vi "ParseSpec2.vi"(8 "error in (no error)":errorcluster, 11 "Spec XML":string="<?xml version=\"1.0\" encoding=\"utf-8\"?>\n<Medulla>\n  <Doctype>Result</Doctype>\n  <Checksum>Spec</Checksum>\n  <DriverKey>NA</DriverKey>\n  <SpecId>NA</SpecId>\n  <TransactionId>0</TransactionId>\n  <AccountID>Audinate</AccountID>\n  <SpecName>Fremont_PCB</SpecName>\n  <WorkflowStep>Fremont_PCB</WorkflowStep>\n  <SerialNumber></SerialNumber>\n  <BatchNumber></BatchNumber>\n  <Status></Status>\n  <Comment></Comment>\n  <FirstFail></FirstFail>\n  <Employee></Employee>\n  <LocalMachine></LocalMachine>\n  <ResourceKey></ResourceKey>\n  <Date></Date>\n  <Time></Time>\n  <Duration></Duration>\n  <DUTPosition />\n  <Components></Components>\n  <Attributes></Attributes>\n  <Tests>\n    <Test>\n      <Code>1</Code>\n      <Name>Short_Circuit</Name>\n      <Description>short circuit tests</Description>\n      <Group></Group>\n      <IsGroup>Yes</IsGroup>\n      <Tag>Short_Circuit</Tag>\n      <Method></Method>\n      <Parameter />\n      <DataType></DataType>\n      <Value></Value>\n      <Status></Status>\n      <LimitLo></LimitLo>\n      <LimitHi></LimitHi>\n      <StringMatch></StringMatch>\n      <BooleanMatch></BooleanMatch>\n      <DisplayFormat></DisplayFormat>\n      <Units></Units>\n      <TestTime></TestTime>\n    </Test>\n    <Test>\n      <Code>1.1</Code>\n      <Name>Short_Circuit_Test</Name>\n      <Description>Tests the short circuit</Description>\n      <Group>Short_Circuit</Group>\n      <IsGroup>No</IsGroup>\n      <Tag>Short_Circuit:Short_Circuit_Test</Tag>\n      <Method>Test_Short_Circuit</Method>\n      <Parameter></Parameter>\n      <DataType>Dbl</DataType>\n      <Value></Value>\n      <Status></Status>\n      <LimitLo>-0.5</LimitLo>\n      <LimitHi>2.5</LimitHi>\n      <StringMatch></StringMatch>\n      <BooleanMatch></BooleanMatch>\n      <DisplayFormat>%.1f</DisplayFormat>\n      <Units>_mA</Units>\n      <TestTime></TestTime>\n    </Test>\n    <Test>\n      <Code>2</Code>\n      <Name>Power_On_3V3</Name>\n      <Description>Power on tests</Description>\n      <Group></Group>\n      <IsGroup>Yes</IsGroup>\n      <Tag>Power_On_3V3</Tag>\n      <Method></Method>\n      <Parameter />\n      <DataType></DataType>\n      <Value></Value>\n      <Status></Status>\n      <LimitLo></LimitLo>\n      <LimitHi></LimitHi>\n      <StringMatch></StringMatch>\n      <BooleanMatch></BooleanMatch>\n      <DisplayFormat></DisplayFormat>\n      <Units></Units>\n      <TestTime></TestTime>\n    </Test>\n    <Test>\n      <Code>2.1</Code>\n      <Name>Setup</Name>\n      <Description>Setup power on 3V3</Description>\n      <Group>Power_On_3V3</Group>\n      <IsGroup>No</IsGroup>\n      <Tag>Power_On_3V3:Setup</Tag>\n      <Method>Setup_Power_On</Method>\n      <Parameter></Parameter>\n      <DataType>Boolean</DataType>\n      <Value></Value>\n      <Status></Status>\n      <LimitLo></LimitLo>\n      <LimitHi></LimitHi>\n      <StringMatch></StringMatch>\n      <BooleanMatch>1</BooleanMatch>\n      <DisplayFormat></DisplayFormat>\n      <Units></Units>\n      <TestTime></TestTime>\n    </Test>\n    <Test>\n      <Code>2.2</Code>\n      <Name>Test_3V3_I</Name>\n      <Description>Test the 3V3 line</Description>\n      <Group>Power_On_3V3</Group>\n      <IsGroup>No</IsGroup>\n      <Tag>Power_On_3V3:Test_3V3_I</Tag>\n      <Method>Test_Power_On</Method>\n      <Parameter></Parameter>\n      <DataType>Dbl</DataType>\n      <Value></Value>\n      <Status></Status>\n      <LimitLo>50</LimitLo>\n      <LimitHi>500</LimitHi>\n      <StringMatch></StringMatch>\n      <BooleanMatch></BooleanMatch>\n      <DisplayFormat>%.1f</DisplayFormat>\n      <Units>_mA</Units>\n      <TestTime></TestTime>\n    </Test>\n    <Test>\n      <Code>3</Code>\n      <Name>Program_DUT</Name>\n      <Description>Perform JTAG programming</Description>\n      <Group></Group>\n      <IsGroup>Yes</IsGroup>\n      <Tag>Program_DUT</Tag>\n      <Method></Method>\n      <Parameter />\n      <DataType></DataType>\n      <Value></Value>\n      <Status></Status>\n      <LimitLo></LimitLo>\n      <LimitHi></LimitHi>\n      <StringMatch></StringMatch>\n      <BooleanMatch></BooleanMatch>\n      <DisplayFormat></DisplayFormat>\n      <Units></Units>\n      <TestTime></TestTime>\n    </Test>\n    <Test>\n      <Code>3.1</Code>\n      <Name>JTAG_Image</Name>\n      <Description>Set the FPGA image</Description>\n      <Group>Program_DUT</Group>\n      <IsGroup>No</IsGroup>\n      <Tag>Program_DUT:JTAG_Image</Tag>\n      <Method>ProgramTestImage</Method>\n      <Parameter>fremont_tx.bit</Parameter>\n      <DataType>Boolean</DataType>\n      <Value></Value>\n      <Status></Status>\n      <LimitLo></LimitLo>\n      <LimitHi></LimitHi>\n      <StringMatch></StringMatch>\n      <BooleanMatch>1</BooleanMatch>\n      <DisplayFormat></DisplayFormat>\n      <Units></Units>\n      <TestTime></TestTime>\n    </Test>\n    <Test>\n      <Code>4</Code>\n      <Name>Operating_Current</Name>\n      <Description>Measure the operating V and I</Description>\n      <Group></Group>\n      <IsGroup>Yes</IsGroup>\n      <Tag>Operating_Current</Tag>\n      <Method></Method>\n      <Parameter />\n      <DataType></DataType>\n      <Value></Value>\n      <Status></Status>\n      <LimitLo></LimitLo>\n      <LimitHi></LimitHi>\n      <StringMatch></StringMatch>\n      <BooleanMatch></BooleanMatch>\n      <DisplayFormat></DisplayFormat>\n      <Units></Units>\n      <TestTime></TestTime>\n    </Test>\n    <Test>\n      <Code>4.1</Code>\n      <Name>Test_3V3_V</Name>\n      <Description>Test the 3V3 line V</Description>\n      <Group>Operating_Current</Group>\n      <IsGroup>No</IsGroup>\n      <Tag>Operating_Current:Test_3V3_V</Tag>\n      <Method>Test_Operating_Voltage</Method>\n      <Parameter></Parameter>\n      <DataType>Dbl</DataType>\n      <Value></Value>\n      <Status></Status>\n      <LimitLo>3.2</LimitLo>\n      <LimitHi>3.4</LimitHi>\n      <StringMatch></StringMatch>\n      <BooleanMatch></BooleanMatch>\n      <DisplayFormat>%.2f</DisplayFormat>\n      <Units>_V</Units>\n      <TestTime></TestTime>\n    </Test>\n    <Test>\n      <Code>4.2</Code>\n      <Name>Test_3V3_I</Name>\n      <Description>Test the 3V3 line V</Description>\n      <Group>Operating_Current</Group>\n      <IsGroup>No</IsGroup>\n      <Tag>Opearating_Current:Test_3V3_I</Tag>\n      <Method>Test_Operating_Current</Method>\n      <Parameter></Parameter>\n      <DataType>Dbl</DataType>\n      <Value></Value>\n      <Status></Status>\n      <LimitLo>200</LimitLo>\n      <LimitHi>500</LimitHi>\n      <StringMatch></StringMatch>\n      <BooleanMatch></BooleanMatch>\n      <DisplayFormat>%.1f</DisplayFormat>\n      <Units>_mA</Units>\n      <TestTime></TestTime>\n    </Test>\n    <Test>\n      <Code>5</Code>\n      <Name>RS232_Verification</Name>\n      <Description>Verify that can read serial</Description>\n      <Group></Group>\n      <IsGroup>Yes</IsGroup>\n      <Tag>RS232_Verification</Tag>\n      <Method></Method>\n      <Parameter />\n      <DataType></DataType>\n      <Value></Value>\n      <Status></Status>\n      <LimitLo></LimitLo>\n      <LimitHi></LimitHi>\n      <StringMatch></StringMatch>\n      <BooleanMatch></BooleanMatch>\n      <DisplayFormat></DisplayFormat>\n      <Units></Units>\n      <TestTime></TestTime>\n    </Test>\n    <Test>\n      <Code>5.1</Code>\n      <Name>Set_HIZ</Name>\n      <Description>Check HIZ response</Description>\n      <Group>RS232_Verification</Group>\n      <IsGroup>No</IsGroup>\n      <Tag>RS232_Verification:Set_HIZ</Tag>\n      <Method>RS232_Verification</Method>\n      <Parameter></Parameter>\n      <DataType>Boolean</DataType>\n      <Value></Value>\n      <Status></Status>\n      <LimitLo></LimitLo>\n      <LimitHi></LimitHi>\n      <StringMatch></StringMatch>\n      <BooleanMatch>1</BooleanMatch>\n      <DisplayFormat></DisplayFormat>\n      <Units></Units>\n      <TestTime></TestTime>\n    </Test>\n    <Test>\n      <Code>6</Code>\n      <Name>DDR2_Verification</Name>\n      <Description>DDR2 Verification</Description>\n      <Group></Group>\n      <IsGroup>Yes</IsGroup>\n      <Tag>DDR2_Verification</Tag>\n      <Method></Method>\n      <Parameter />\n      <DataType></DataType>\n      <Value></Value>\n      <Status></Status>\n      <LimitLo></LimitLo>\n      <LimitHi></LimitHi>\n      <StringMatch></StringMatch>\n      <BooleanMatch></BooleanMatch>\n      <DisplayFormat></DisplayFormat>\n      <Units></Units>\n      <TestTime></TestTime>\n    </Test>\n    <Test>\n      <Code>6.1</Code>\n      <Name>DDR2_Memory</Name>\n      <Description>Check DDR2 Mem</Description>\n      <Group>DDR2_Verification</Group>\n      <IsGroup>No</IsGroup>\n      <Tag>DDR2_Verification:DDR2_Memory</Tag>\n      <Method>DDR2_Verification</Method>\n      <Parameter></Parameter>\n      <DataType>Boolean</DataType>\n      <Value></Value>\n      <Status></Status>\n      <LimitLo></LimitLo>\n      <LimitHi></LimitHi>\n      <StringMatch></StringMatch>\n      <BooleanMatch>1</BooleanMatch>\n      <DisplayFormat></DisplayFormat>\n      <Units></Units>\n      <TestTime></TestTime>\n    </Test>\n    <Test>\n      <Code>7</Code>\n      <Name>SPI_Flash</Name>\n      <Description>SPI Flash Programing</Description>\n      <Group></Group>\n      <IsGroup>Yes</IsGroup>\n      <Tag>SPI_Flash</Tag>\n      <Method></Method>\n      <Parameter />\n      <DataType></DataType>\n      <Value></Value>\n      <Status></Status>\n      <LimitLo></LimitLo>\n      <LimitHi></LimitHi>\n      <StringMatch></StringMatch>\n      <BooleanMatch></BooleanMatch>\n      <DisplayFormat></DisplayFormat>\n      <Units></Units>\n      <TestTime></TestTime>\n    </Test>\n    <Test>\n      <Code>7.1</Code>\n      <Name>Program</Name>\n      <Description>Program the fremont</Description>\n      <Group>SPI_Flash</Group>\n      <IsGroup>No</IsGroup>\n      <Tag>SPI_Flash:Program</Tag>\n      <Method>StartFlash</Method>\n      <Parameter>ULL_FREMONT_TX.bin</Parameter>\n      <DataType>Boolean</DataType>\n      <Value></Value>\n      <Status></Status>\n      <LimitLo></LimitLo>\n      <LimitHi></LimitHi>\n      <StringMatch></StringMatch>\n      <BooleanMatch>1</BooleanMatch>\n      <DisplayFormat></DisplayFormat>\n      <Units></Units>\n      <TestTime></TestTime>\n    </Test>\n    <Test>\n      <Code>8</Code>\n      <Name>Frequency_Tests</Name>\n      <Description>Frequency tests</Description>\n      <Group></Group>\n      <IsGroup>Yes</IsGroup>\n      <Tag>Frequency_Tests</Tag>\n      <Method></Method>\n      <Parameter />\n      <DataType></DataType>\n      <Value></Value>\n      <Status></Status>\n      <LimitLo></LimitLo>\n      <LimitHi></LimitHi>\n      <StringMatch></StringMatch>\n      <BooleanMatch></BooleanMatch>\n      <DisplayFormat></DisplayFormat>\n      <Units></Units>\n      <TestTime></TestTime>\n    </Test>\n    <Test>\n      <Code>8.1</Code>\n      <Name>VCXO_0_LF</Name>\n      <Description>frequency test</Description>\n      <Group>Frequency_Tests</Group>\n      <IsGroup>No</IsGroup>\n      <Tag>Frequency_Tests:VCXO_0_LF</Tag>\n      <Method>Frequency_Test_VCXO_0_LF</Method>\n      <Parameter></Parameter>\n      <DataType>Dbl</DataType>\n      <Value></Value>\n      <Status></Status>\n      <LimitLo>983090</LimitLo>\n      <LimitHi>983094</LimitHi>\n      <StringMatch></StringMatch>\n      <BooleanMatch></BooleanMatch>\n      <DisplayFormat>%.0f</DisplayFormat>\n      <Units>_Hz</Units>\n      <TestTime></TestTime>\n    </Test>\n    <Test>\n      <Code>8.2</Code>\n      <Name>VCXO_0_HF</Name>\n      <Description>frequency test</Description>\n      <Group>Frequency_Tests</Group>\n      <IsGroup>No</IsGroup>\n      <Tag>Frequency_Tests:VCXO_0_HF</Tag>\n      <Method>Frequency_Test_VCXO_0_HF</Method>\n      <Parameter></Parameter>\n      <DataType>Dbl</DataType>\n      <Value></Value>\n      <Status></Status>\n      <LimitLo>983090</LimitLo>\n      <LimitHi>983094</LimitHi>\n      <StringMatch></StringMatch>\n      <BooleanMatch></BooleanMatch>\n      <DisplayFormat>%.0f</DisplayFormat>\n      <Units>_Hz</Units>\n      <TestTime></TestTime>\n    </Test>\n    <Test>\n      <Code>8.3</Code>\n      <Name>VCXO_M</Name>\n      <Description>frequency test</Description>\n      <Group>Frequency_Tests</Group>\n      <IsGroup>No</IsGroup>\n      <Tag>Frequency_Tests:VCXO_M</Tag>\n      <Method>Frequency_Test_VCXO_M</Method>\n      <Parameter></Parameter>\n      <DataType>Dbl</DataType>\n      <Value></Value>\n      <Status></Status>\n      <LimitLo>983090</LimitLo>\n      <LimitHi>983094</LimitHi>\n      <StringMatch></StringMatch>\n      <BooleanMatch></BooleanMatch>\n      <DisplayFormat>%.0f</DisplayFormat>\n      <Units>_Hz</Units>\n      <TestTime></TestTime>\n    </Test>\n    <Test>\n      <Code>8.4</Code>\n      <Name>VCXO_H</Name>\n      <Description>frequency test</Description>\n      <Group>Frequency_Tests</Group>\n      <IsGroup>No</IsGroup>\n      <Tag>Frequency_Tests:VCXO_H</Tag>\n      <Method>Frequency_Test_VCXO_H</Method>\n      <Parameter></Parameter>\n      <DataType>Dbl</DataType>\n      <Value></Value>\n      <Status></Status>\n      <LimitLo>983090</LimitLo>\n      <LimitHi>983094</LimitHi>\n      <StringMatch></StringMatch>\n      <BooleanMatch></BooleanMatch>\n      <DisplayFormat>%.0f</DisplayFormat>\n      <Units>_Hz</Units>\n      <TestTime></TestTime>\n    </Test>\n    <Test>\n      <Code>8.5</Code>\n      <Name>VCXO_L</Name>\n      <Description>frequency test</Description>\n      <Group>Frequency_Tests</Group>\n      <IsGroup>No</IsGroup>\n      <Tag>Frequency_Tests:VCXO_L</Tag>\n      <Method>Frequency_Test_VCXO_L</Method>\n      <Parameter></Parameter>\n      <DataType>Dbl</DataType>\n      <Value></Value>\n      <Status></Status>\n      <LimitLo>983090</LimitLo>\n      <LimitHi>983094</LimitHi>\n      <StringMatch></StringMatch>\n      <BooleanMatch></BooleanMatch>\n      <DisplayFormat>%.0f</DisplayFormat>\n      <Units>_Hz</Units>\n      <TestTime></TestTime>\n    </Test>\n    <Test>\n      <Code>8.6</Code>\n      <Name>VCXO_2</Name>\n      <Description>frequency test</Description>\n      <Group>Frequency_Tests</Group>\n      <IsGroup>No</IsGroup>\n      <Tag>Frequency_Tests:VCXO_2</Tag>\n      <Method>Frequency_Test_VCXO_2</Method>\n      <Parameter></Parameter>\n      <DataType>Dbl</DataType>\n      <Value></Value>\n      <Status></Status>\n      <LimitLo>983090</LimitLo>\n      <LimitHi>983094</LimitHi>\n      <StringMatch></StringMatch>\n      <BooleanMatch></BooleanMatch>\n      <DisplayFormat>%.0f</DisplayFormat>\n      <Units>_Hz</Units>\n      <TestTime></TestTime>\n    </Test>\n    <Test>\n      <Code>9</Code>\n      <Name>VCXO_PWM_Resistors</Name>\n      <Description>VCXO_PWM</Description>\n      <Group></Group>\n      <IsGroup>Yes</IsGroup>\n      <Tag>VCXO_PWM</Tag>\n      <Method></Method>\n      <Parameter />\n      <DataType></DataType>\n      <Value></Value>\n      <Status></Status>\n      <LimitLo></LimitLo>\n      <LimitHi></LimitHi>\n      <StringMatch></StringMatch>\n      <BooleanMatch></BooleanMatch>\n      <DisplayFormat></DisplayFormat>\n      <Units></Units>\n      <TestTime></TestTime>\n    </Test>\n    <Test>\n      <Code>9.1</Code>\n      <Name>I_H_H</Name>\n      <Description></Description>\n      <Group>VCXO_PWM</Group>\n      <IsGroup>No</IsGroup>\n      <Tag>VCXO_PWM:I_H_H</Tag>\n      <Method>Test_VCXO_PWM_I_H_H</Method>\n      <Parameter></Parameter>\n      <DataType>Dbl</DataType>\n      <Value></Value>\n      <Status></Status>\n      <LimitLo>1.5</LimitLo>\n      <LimitHi>1.7</LimitHi>\n      <StringMatch></StringMatch>\n      <BooleanMatch></BooleanMatch>\n      <DisplayFormat>%.2f</DisplayFormat>\n      <Units>_V</Units>\n      <TestTime></TestTime>\n    </Test>\n    <Test>\n      <Code>9.2</Code>\n      <Name>I_L_L</Name>\n      <Description></Description>\n      <Group>VCXO_PWM</Group>\n      <IsGroup>No</IsGroup>\n      <Tag>VCXO_PWM:I_L_L</Tag>\n      <Method>Test_VCXO_PWM_I_L_L</Method>\n      <Parameter></Parameter>\n      <DataType>Dbl</DataType>\n      <Value></Value>\n      <Status></Status>\n      <LimitLo>1.5</LimitLo>\n      <LimitHi>1.7</LimitHi>\n      <StringMatch></StringMatch>\n      <BooleanMatch></BooleanMatch>\n      <DisplayFormat>%.2f</DisplayFormat>\n      <Units>_V</Units>\n      <TestTime></TestTime>\n    </Test>\n    <Test>\n      <Code>9.3</Code>\n      <Name>I_H_L</Name>\n      <Description></Description>\n      <Group>VCXO_PWM</Group>\n      <IsGroup>No</IsGroup>\n      <Tag>VCXO_PWM:I_H_L</Tag>\n      <Method>Test_VCXO_PWM_I_H_L</Method>\n      <Parameter></Parameter>\n      <DataType>Dbl</DataType>\n      <Value></Value>\n      <Status></Status>\n      <LimitLo>1.5</LimitLo>\n      <LimitHi>1.7</LimitHi>\n      <StringMatch></StringMatch>\n      <BooleanMatch></BooleanMatch>\n      <DisplayFormat>%.2f</DisplayFormat>\n      <Units>_V</Units>\n      <TestTime></TestTime>\n    </Test>\n    <Test>\n      <Code>9.4</Code>\n      <Name>I_L_H</Name>\n      <Description></Description>\n      <Group>VCXO_PWM</Group>\n      <IsGroup>No</IsGroup>\n      <Tag>VCXO_PWM:I_L_H</Tag>\n      <Method>Test_VCXO_PWM_I_L_H</Method>\n      <Parameter></Parameter>\n      <DataType>Dbl</DataType>\n      <Value></Value>\n      <Status></Status>\n      <LimitLo>1.5</LimitLo>\n      <LimitHi>1.7</LimitHi>\n      <StringMatch></StringMatch>\n      <BooleanMatch></BooleanMatch>\n      <DisplayFormat>%.2f</DisplayFormat>\n      <Units>_V</Units>\n      <TestTime></TestTime>\n    </Test>\n    <Test>\n      <Code>10</Code>\n      <Name>Pin_Tests</Name>\n      <Description>Test all the pins for H and L</Description>\n      <Group></Group>\n      <IsGroup>Yes</IsGroup>\n      <Tag>Pin_Tests</Tag>\n      <Method></Method>\n      <Parameter />\n      <DataType></DataType>\n      <Value></Value>\n      <Status></Status>\n      <LimitLo></LimitLo>\n      <LimitHi></LimitHi>\n      <StringMatch></StringMatch>\n      <BooleanMatch></BooleanMatch>\n      <DisplayFormat></DisplayFormat>\n      <Units></Units>\n      <TestTime></TestTime>\n    </Test>\n    <Test>\n      <Code>10.1</Code>\n      <Name>Setup_Pins</Name>\n      <Description>setup the pin tests </Description>\n      <Group>Pin_Tests</Group>\n      <IsGroup>No</IsGroup>\n      <Tag>Pin_Tests:Setup_Pins</Tag>\n      <Method>Setup_Pin_Tests</Method>\n      <Parameter></Parameter>\n      <DataType>Boolean</DataType>\n      <Value></Value>\n      <Status></Status>\n      <LimitLo></LimitLo>\n      <LimitHi></LimitHi>\n      <StringMatch></StringMatch>\n      <BooleanMatch>1</BooleanMatch>\n      <DisplayFormat></DisplayFormat>\n      <Units></Units>\n      <TestTime></TestTime>\n    </Test>\n    <Test>\n      <Code>10.2</Code>\n      <Name>SELECTOR_1_H</Name>\n      <Description></Description>\n      <Group>Pin_Tests</Group>\n      <IsGroup>No</IsGroup>\n      <Tag>Pin_Tests:SELECTOR_1_H</Tag>\n      <Method>Test_Pin_N_High</Method>\n      <Parameter>CH1</Parameter>\n      <DataType>Dbl</DataType>\n      <Value></Value>\n      <Status></Status>\n      <LimitLo>3.2</LimitLo>\n      <LimitHi>3.4</LimitHi>\n      <StringMatch></StringMatch>\n      <BooleanMatch></BooleanMatch>\n      <DisplayFormat>%.2f</DisplayFormat>\n      <Units>_V</Units>\n      <TestTime></TestTime>\n    </Test>\n    <Test>\n      <Code>10.3</Code>\n      <Name>SELECTOR_1_L</Name>\n      <Description></Description>\n      <Group>Pin_Tests</Group>\n      <IsGroup>No</IsGroup>\n      <Tag>Pin_Tests:SELECTOR_1_L</Tag>\n      <Method>Test_Pin_N_Low</Method>\n      <Parameter>CH1</Parameter>\n      <DataType>Dbl</DataType>\n      <Value></Value>\n      <Status></Status>\n      <LimitLo>0</LimitLo>\n      <LimitHi>0.01</LimitHi>\n      <StringMatch></StringMatch>\n      <BooleanMatch></BooleanMatch>\n      <DisplayFormat>%.2f</DisplayFormat>\n      <Units>_V</Units>\n      <TestTime></TestTime>\n    </Test>\n    <Test>\n      <Code>10.4</Code>\n      <Name>SELECTOR_2_H</Name>\n      <Description></Description>\n      <Group>Pin_Tests</Group>\n      <IsGroup>No</IsGroup>\n      <Tag>Pin_Tests:SELECTOR_2_H</Tag>\n      <Method>Test_Pin_N_High</Method>\n      <Parameter>CH2</Parameter>\n      <DataType>Dbl</DataType>\n      <Value></Value>\n      <Status></Status>\n      <LimitLo>3.2</LimitLo>\n      <LimitHi>3.4</LimitHi>\n      <StringMatch></StringMatch>\n      <BooleanMatch></BooleanMatch>\n      <DisplayFormat>%.2f</DisplayFormat>\n      <Units>_V</Units>\n      <TestTime></TestTime>\n    </Test>\n    <Test>\n      <Code>10.5</Code>\n      <Name>SELECTOR_2_L</Name>\n      <Description></Description>\n      <Group>Pin_Tests</Group>\n      <IsGroup>No</IsGroup>\n      <Tag>Pin_Tests:SELECTOR_2_L</Tag>\n      <Method>Test_Pin_N_Low</Method>\n      <Parameter>CH2</Parameter>\n      <DataType>Dbl</DataType>\n      <Value></Value>\n      <Status></Status>\n      <LimitLo>0</LimitLo>\n      <LimitHi>0.01</LimitHi>\n      <StringMatch></StringMatch>\n      <BooleanMatch></BooleanMatch>\n      <DisplayFormat>%.2f</DisplayFormat>\n      <Units>_V</Units>\n      <TestTime></TestTime>\n    </Test>\n    <Test>\n      <Code>10.6</Code>\n      <Name>SELECTOR_3_H</Name>\n      <Description></Description>\n      <Group>Pin_Tests</Group>\n      <IsGroup>No</IsGroup>\n      <Tag>Pin_Tests:SELECTOR_3_H</Tag>\n      <Method>Test_Pin_N_High</Method>\n      <Parameter>CH3</Parameter>\n      <DataType>Dbl</DataType>\n      <Value></Value>\n      <Status></Status>\n      <LimitLo>3.2</LimitLo>\n      <LimitHi>3.4</LimitHi>\n      <StringMatch></StringMatch>\n      <BooleanMatch></BooleanMatch>\n      <DisplayFormat>%.2f</DisplayFormat>\n      <Units>_V</Units>\n      <TestTime></TestTime>\n    </Test>\n    <Test>\n      <Code>10.7</Code>\n      <Name>SELECTOR_3_L</Name>\n      <Description></Description>\n      <Group>Pin_Tests</Group>\n      <IsGroup>No</IsGroup>\n      <Tag>Pin_Tests:SELECTOR_3_L</Tag>\n      <Method>Test_Pin_N_Low</Method>\n      <Parameter>CH3</Parameter>\n      <DataType>Dbl</DataType>\n      <Value></Value>\n      <Status></Status>\n      <LimitLo>0</LimitLo>\n      <LimitHi>0.01</LimitHi>\n      <StringMatch></StringMatch>\n      <BooleanMatch></BooleanMatch>\n      <DisplayFormat>%.2f</DisplayFormat>\n      <Units>_V</Units>\n      <TestTime></TestTime>\n    </Test>\n    <Test>\n      <Code>10.8</Code>\n      <Name>SELECTOR_4_H</Name>\n      <Description></Description>\n      <Group>Pin_Tests</Group>\n      <IsGroup>No</IsGroup>\n      <Tag>Pin_Tests:SELECTOR_4_H</Tag>\n      <Method>Test_Pin_N_High</Method>\n      <Parameter>CH4</Parameter>\n      <DataType>Dbl</DataType>\n      <Value></Value>\n      <Status></Status>\n      <LimitLo>3.2</LimitLo>\n      <LimitHi>3.4</LimitHi>\n      <StringMatch></StringMatch>\n      <BooleanMatch></BooleanMatch>\n      <DisplayFormat>%.2f</DisplayFormat>\n      <Units>_V</Units>\n      <TestTime></TestTime>\n    </Test>\n    <Test>\n      <Code>10.9</Code>\n      <Name>SELECTOR_4_L</Name>\n      <Description></Description>\n      <Group>Pin_Tests</Group>\n      <IsGroup>No</IsGroup>\n      <Tag>Pin_Tests:SELECTOR_4_L</Tag>\n      <Method>Test_Pin_N_Low</Method>\n      <Parameter>CH4</Parameter>\n      <DataType>Dbl</DataType>\n      <Value></Value>\n      <Status></Status>\n      <LimitLo>0</LimitLo>\n      <LimitHi>0.01</LimitHi>\n      <StringMatch></StringMatch>\n      <BooleanMatch></BooleanMatch>\n      <DisplayFormat>%.2f</DisplayFormat>\n      <Units>_V</Units>\n      <TestTime></TestTime>\n    </Test>\n    <Test>\n      <Code>10.10</Code>\n      <Name>SELECTOR_5_H</Name>\n      <Description></Description>\n      <Group>Pin_Tests</Group>\n      <IsGroup>No</IsGroup>\n      <Tag>Pin_Tests:SELECTOR_5_H</Tag>\n      <Method>Test_Pin_N_High</Method>\n      <Parameter>CH5</Parameter>\n      <DataType>Dbl</DataType>\n      <Value></Value>\n      <Status></Status>\n      <LimitLo>3.2</LimitLo>\n      <LimitHi>3.4</LimitHi>\n      <StringMatch></StringMatch>\n      <BooleanMatch></BooleanMatch>\n      <DisplayFormat>%.2f</DisplayFormat>\n      <Units>_V</Units>\n      <TestTime></TestTime>\n    </Test>\n    <Test>\n      <Code>10.11</Code>\n      <Name>SELECTOR_5_L</Name>\n      <Description></Description>\n      <Group>Pin_Tests</Group>\n      <IsGroup>No</IsGroup>\n      <Tag>Pin_Tests:SELECTOR_5_L</Tag>\n      <Method>Test_Pin_N_Low</Method>\n      <Parameter>CH5</Parameter>\n      <DataType>Dbl</DataType>\n      <Value></Value>\n      <Status></Status>\n      <LimitLo>0</LimitLo>\n      <LimitHi>0.01</LimitHi>\n      <StringMatch></StringMatch>\n      <BooleanMatch></BooleanMatch>\n      <DisplayFormat>%.2f</DisplayFormat>\n      <Units>_V</Units>\n      <TestTime></TestTime>\n    </Test>\n    <Test>\n      <Code>10.12</Code>\n      <Name>SELECTOR_6_H</Name>\n      <Description></Description>\n      <Group>Pin_Tests</Group>\n      <IsGroup>No</IsGroup>\n      <Tag>Pin_Tests:SELECTOR_6_H</Tag>\n      <Method>Test_Pin_N_High</Method>\n      <Parameter>CH6</Parameter>\n      <DataType>Dbl</DataType>\n      <Value></Value>\n      <Status></Status>\n      <LimitLo>3.2</LimitLo>\n      <LimitHi>3.4</LimitHi>\n      <StringMatch></StringMatch>\n      <BooleanMatch></BooleanMatch>\n      <DisplayFormat>%.2f</DisplayFormat>\n      <Units>_V</Units>\n      <TestTime></TestTime>\n    </Test>\n    <Test>\n      <Code>10.13</Code>\n      <Name>SELECTOR_6_L</Name>\n      <Description></Description>\n      <Group>Pin_Tests</Group>\n      <IsGroup>No</IsGroup>\n      <Tag>Pin_Tests:SELECTOR_6_L</Tag>\n      <Method>Test_Pin_N_Low</Method>\n      <Parameter>CH6</Parameter>\n      <DataType>Dbl</DataType>\n      <Value></Value>\n      <Status></Status>\n      <LimitLo>0</LimitLo>\n      <LimitHi>0.01</LimitHi>\n      <StringMatch></StringMatch>\n      <BooleanMatch></BooleanMatch>\n      <DisplayFormat>%.2f</DisplayFormat>\n      <Units>_V</Units>\n      <TestTime></TestTime>\n    </Test>\n    <Test>\n      <Code>10.14</Code>\n      <Name>SELECTOR_7_H</Name>\n      <Description></Description>\n      <Group>Pin_Tests</Group>\n      <IsGroup>No</IsGroup>\n      <Tag>Pin_Tests:SELECTOR_7_H</Tag>\n      <Method>Test_Pin_N_High</Method>\n      <Parameter>CH7</Parameter>\n      <DataType>Dbl</DataType>\n      <Value></Value>\n      <Status></Status>\n      <LimitLo>3.2</LimitLo>\n      <LimitHi>3.4</LimitHi>\n      <StringMatch></StringMatch>\n      <BooleanMatch></BooleanMatch>\n      <DisplayFormat>%.2f</DisplayFormat>\n      <Units>_V</Units>\n      <TestTime></TestTime>\n    </Test>\n    <Test>\n      <Code>10.15</Code>\n      <Name>SELECTOR_7_L</Name>\n      <Description></Description>\n      <Group>Pin_Tests</Group>\n      <IsGroup>No</IsGroup>\n      <Tag>Pin_Tests:SELECTOR_7_L</Tag>\n      <Method>Test_Pin_N_Low</Method>\n      <Parameter>CH7</Parameter>\n      <DataType>Dbl</DataType>\n      <Value></Value>\n      <Status></Status>\n      <LimitLo>0</LimitLo>\n      <LimitHi>0.01</LimitHi>\n      <StringMatch></StringMatch>\n      <BooleanMatch></BooleanMatch>\n      <DisplayFormat>%.2f</DisplayFormat>\n      <Units>_V</Units>\n      <TestTime></TestTime>\n    </Test>\n    <Test>\n      <Code>10.16</Code>\n      <Name>SELECTOR_8_H</Name>\n      <Description></Description>\n      <Group>Pin_Tests</Group>\n      <IsGroup>No</IsGroup>\n      <Tag>Pin_Tests:SELECTOR_8_H</Tag>\n      <Method>Test_Pin_N_High</Method>\n      <Parameter>CH8</Parameter>\n      <DataType>Dbl</DataType>\n      <Value></Value>\n      <Status></Status>\n      <LimitLo>3.2</LimitLo>\n      <LimitHi>3.4</LimitHi>\n      <StringMatch></StringMatch>\n      <BooleanMatch></BooleanMatch>\n      <DisplayFormat>%.2f</DisplayFormat>\n      <Units>_V</Units>\n      <TestTime></TestTime>\n    </Test>\n    <Test>\n      <Code>10.17</Code>\n      <Name>SELECTOR_8_L</Name>\n      <Description></Description>\n      <Group>Pin_Tests</Group>\n      <IsGroup>No</IsGroup>\n      <Tag>Pin_Tests:SELECTOR_8_L</Tag>\n      <Method>Test_Pin_N_Low</Method>\n      <Parameter>CH8</Parameter>\n      <DataType>Dbl</DataType>\n      <Value></Value>\n      <Status></Status>\n      <LimitLo>0</LimitLo>\n      <LimitHi>0.01</LimitHi>\n      <StringMatch></StringMatch>\n      <BooleanMatch></BooleanMatch>\n      <DisplayFormat>%.2f</DisplayFormat>\n      <Units>_V</Units>\n      <TestTime></TestTime>\n    </Test>\n    <Test>\n      <Code>10.18</Code>\n      <Name>SELECTOR_9_H</Name>\n      <Description></Description>\n      <Group>Pin_Tests</Group>\n      <IsGroup>No</IsGroup>\n      <Tag>Pin_Tests:SELECTOR_9_H</Tag>\n      <Method>Test_Pin_N_High</Method>\n      <Parameter>CH9</Parameter>\n      <DataType>Dbl</DataType>\n      <Value></Value>\n      <Status></Status>\n      <LimitLo>3.2</LimitLo>\n      <LimitHi>3.4</LimitHi>\n      <StringMatch></StringMatch>\n      <BooleanMatch></BooleanMatch>\n      <DisplayFormat>%.2f</DisplayFormat>\n      <Units>_V</Units>\n      <TestTime></TestTime>\n    </Test>\n    <Test>\n      <Code>10.19</Code>\n      <Name>SELECTOR_9_L</Name>\n      <Description></Description>\n      <Group>Pin_Tests</Group>\n      <IsGroup>No</IsGroup>\n      <Tag>Pin_Tests:SELECTOR_9_L</Tag>\n      <Method>Test_Pin_N_Low</Method>\n      <Parameter>CH9</Parameter>\n      <DataType>Dbl</DataType>\n      <Value></Value>\n      <Status></Status>\n      <LimitLo>0</LimitLo>\n      <LimitHi>0.01</LimitHi>\n      <StringMatch></StringMatch>\n      <BooleanMatch></BooleanMatch>\n      <DisplayFormat>%.2f</DisplayFormat>\n      <Units>_V</Units>\n      <TestTime></TestTime>\n    </Test>\n    <Test>\n      <Code>10.20</Code>\n      <Name>SELECTOR_10_H</Name>\n      <Description></Description>\n      <Group>Pin_Tests</Group>\n      <IsGroup>No</IsGroup>\n      <Tag>Pin_Tests:SELECTOR_10_H</Tag>\n      <Method>Test_Pin_N_High</Method>\n      <Parameter>CH10</Parameter>\n      <DataType>Dbl</DataType>\n      <Value></Value>\n      <Status></Status>\n      <LimitLo>3.2</LimitLo>\n      <LimitHi>3.4</LimitHi>\n      <StringMatch></StringMatch>\n      <BooleanMatch></BooleanMatch>\n      <DisplayFormat>%.2f</DisplayFormat>\n      <Units>_V</Units>\n      <TestTime></TestTime>\n    </Test>\n    <Test>\n      <Code>10.21</Code>\n      <Name>SELECTOR_10_L</Name>\n      <Description></Description>\n      <Group>Pin_Tests</Group>\n      <IsGroup>No</IsGroup>\n      <Tag>Pin_Tests:SELECTOR_10_L</Tag>\n      <Method>Test_Pin_N_Low</Method>\n      <Parameter>CH10</Parameter>\n      <DataType>Dbl</DataType>\n      <Value></Value>\n      <Status></Status>\n      <LimitLo>0</LimitLo>\n      <LimitHi>0.01</LimitHi>\n      <StringMatch></StringMatch>\n      <BooleanMatch></BooleanMatch>\n      <DisplayFormat>%.2f</DisplayFormat>\n      <Units>_V</Units>\n      <TestTime></TestTime>\n    </Test>\n    <Test>\n      <Code>10.22</Code>\n      <Name>SELECTOR_11_H</Name>\n      <Description></Description>\n      <Group>Pin_Tests</Group>\n      <IsGroup>No</IsGroup>\n      <Tag>Pin_Tests:SELECTOR_11_H</Tag>\n      <Method>Test_Pin_N_High</Method>\n      <Parameter>CH11</Parameter>\n      <DataType>Dbl</DataType>\n      <Value></Value>\n      <Status></Status>\n      <LimitLo>3.2</LimitLo>\n      <LimitHi>3.4</LimitHi>\n      <StringMatch></StringMatch>\n      <BooleanMatch></BooleanMatch>\n      <DisplayFormat>%.2f</DisplayFormat>\n      <Units>_V</Units>\n      <TestTime></TestTime>\n    </Test>\n    <Test>\n      <Code>10.23</Code>\n      <Name>SELECTOR_11_L</Name>\n      <Description></Description>\n      <Group>Pin_Tests</Group>\n      <IsGroup>No</IsGroup>\n      <Tag>Pin_Tests:SELECTOR_11_L</Tag>\n      <Method>Test_Pin_N_Low</Method>\n      <Parameter>CH11</Parameter>\n      <DataType>Dbl</DataType>\n      <Value></Value>\n      <Status></Status>\n      <LimitLo>0</LimitLo>\n      <LimitHi>0.01</LimitHi>\n      <StringMatch></StringMatch>\n      <BooleanMatch></BooleanMatch>\n      <DisplayFormat>%.2f</DisplayFormat>\n      <Units>_V</Units>\n      <TestTime></TestTime>\n    </Test>\n    <Test>\n      <Code>10.24</Code>\n      <Name>SELECTOR_12_H</Name>\n      <Description></Description>\n      <Group>Pin_Tests</Group>\n      <IsGroup>No</IsGroup>\n      <Tag>Pin_Tests:SELECTOR_12_H</Tag>\n      <Method>Test_Pin_N_High</Method>\n      <Parameter>CH12</Parameter>\n      <DataType>Dbl</DataType>\n      <Value></Value>\n      <Status></Status>\n      <LimitLo>3.2</LimitLo>\n      <LimitHi>3.4</LimitHi>\n      <StringMatch></StringMatch>\n      <BooleanMatch></BooleanMatch>\n      <DisplayFormat>%.2f</DisplayFormat>\n      <Units>_V</Units>\n      <TestTime></TestTime>\n    </Test>\n    <Test>\n      <Code>10.25</Code>\n      <Name>SELECTOR_12_L</Name>\n      <Description></Description>\n      <Group>Pin_Tests</Group>\n      <IsGroup>No</IsGroup>\n      <Tag>Pin_Tests:SELECTOR_12_L</Tag>\n      <Method>Test_Pin_N_Low</Method>\n      <Parameter>CH12</Parameter>\n      <DataType>Dbl</DataType>\n      <Value></Value>\n      <Status></Status>\n      <LimitLo>0</LimitLo>\n      <LimitHi>0.01</LimitHi>\n      <StringMatch></StringMatch>\n      <BooleanMatch></BooleanMatch>\n      <DisplayFormat>%.2f</DisplayFormat>\n      <Units>_V</Units>\n      <TestTime></TestTime>\n    </Test>\n    <Test>\n      <Code>10.26</Code>\n      <Name>SELECTOR_13_H</Name>\n      <Description></Description>\n      <Group>Pin_Tests</Group>\n      <IsGroup>No</IsGroup>\n      <Tag>Pin_Tests:SELECTOR_13_H</Tag>\n      <Method>Test_Pin_N_High</Method>\n      <Parameter>CH13</Parameter>\n      <DataType>Dbl</DataType>\n      <Value></Value>\n      <Status></Status>\n      <LimitLo>3.2</LimitLo>\n      <LimitHi>3.4</LimitHi>\n      <StringMatch></StringMatch>\n      <BooleanMatch></BooleanMatch>\n      <DisplayFormat>%.2f</DisplayFormat>\n      <Units>_V</Units>\n      <TestTime></TestTime>\n    </Test>\n    <Test>\n      <Code>10.27</Code>\n      <Name>SELECTOR_13_L</Name>\n      <Description></Description>\n      <Group>Pin_Tests</Group>\n      <IsGroup>No</IsGroup>\n      <Tag>Pin_Tests:SELECTOR_13_L</Tag>\n      <Method>Test_Pin_N_Low</Method>\n      <Parameter>CH13</Parameter>\n      <DataType>Dbl</DataType>\n      <Value></Value>\n      <Status></Status>\n      <LimitLo>0</LimitLo>\n      <LimitHi>0.01</LimitHi>\n      <StringMatch></StringMatch>\n      <BooleanMatch></BooleanMatch>\n      <DisplayFormat>%.2f</DisplayFormat>\n      <Units>_V</Units>\n      <TestTime></TestTime>\n    </Test>\n    <Test>\n      <Code>10.28</Code>\n      <Name>SELECTOR_14_H</Name>\n      <Description></Description>\n      <Group>Pin_Tests</Group>\n      <IsGroup>No</IsGroup>\n      <Tag>Pin_Tests:SELECTOR_14_H</Tag>\n      <Method>Test_Pin_N_High</Method>\n      <Parameter>CH14</Parameter>\n      <DataType>Dbl</DataType>\n      <Value></Value>\n      <Status></Status>\n      <LimitLo>3.2</LimitLo>\n      <LimitHi>3.4</LimitHi>\n      <StringMatch></StringMatch>\n      <BooleanMatch></BooleanMatch>\n      <DisplayFormat>%.2f</DisplayFormat>\n      <Units>_V</Units>\n      <TestTime></TestTime>\n    </Test>\n    <Test>\n      <Code>10.29</Code>\n      <Name>SELECTOR_14_L</Name>\n      <Description></Description>\n      <Group>Pin_Tests</Group>\n      <IsGroup>No</IsGroup>\n      <Tag>Pin_Tests:SELECTOR_14_L</Tag>\n      <Method>Test_Pin_N_Low</Method>\n      <Parameter>CH14</Parameter>\n      <DataType>Dbl</DataType>\n      <Value></Value>\n      <Status></Status>\n      <LimitLo>0</LimitLo>\n      <LimitHi>0.01</LimitHi>\n      <StringMatch></StringMatch>\n      <BooleanMatch></BooleanMatch>\n      <DisplayFormat>%.2f</DisplayFormat>\n      <Units>_V</Units>\n      <TestTime></TestTime>\n    </Test>\n    <Test>\n      <Code>10.30</Code>\n      <Name>SELECTOR_15_H</Name>\n      <Description></Description>\n      <Group>Pin_Tests</Group>\n      <IsGroup>No</IsGroup>\n      <Tag>Pin_Tests:SELECTOR_15_H</Tag>\n      <Method>Test_Pin_N_High</Method>\n      <Parameter>CH15</Parameter>\n      <DataType>Dbl</DataType>\n      <Value></Value>\n      <Status></Status>\n      <LimitLo>3.2</LimitLo>\n      <LimitHi>3.4</LimitHi>\n      <StringMatch></StringMatch>\n      <BooleanMatch></BooleanMatch>\n      <DisplayFormat>%.2f</DisplayFormat>\n      <Units>_V</Units>\n      <TestTime></TestTime>\n    </Test>\n    <Test>\n      <Code>10.31</Code>\n      <Name>SELECTOR_15_L</Name>\n      <Description></Description>\n      <Group>Pin_Tests</Group>\n      <IsGroup>No</IsGroup>\n      <Tag>Pin_Tests:SELECTOR_15_L</Tag>\n      <Method>Test_Pin_N_Low</Method>\n      <Parameter>CH15</Parameter>\n      <DataType>Dbl</DataType>\n      <Value></Value>\n      <Status></Status>\n      <LimitLo>0</LimitLo>\n      <LimitHi>0.01</LimitHi>\n      <StringMatch></StringMatch>\n      <BooleanMatch></BooleanMatch>\n      <DisplayFormat>%.2f</DisplayFormat>\n      <Units>_V</Units>\n      <TestTime></TestTime>\n    </Test>\n    <Test>\n      <Code>10.32</Code>\n      <Name>SELECTOR_16_H</Name>\n      <Description></Description>\n      <Group>Pin_Tests</Group>\n      <IsGroup>No</IsGroup>\n      <Tag>Pin_Tests:SELECTOR_16_H</Tag>\n      <Method>Test_Pin_N_High</Method>\n      <Parameter>CH16</Parameter>\n      <DataType>Dbl</DataType>\n      <Value></Value>\n      <Status></Status>\n      <LimitLo>3.2</LimitLo>\n      <LimitHi>3.4</LimitHi>\n      <StringMatch></StringMatch>\n      <BooleanMatch></BooleanMatch>\n      <DisplayFormat>%.2f</DisplayFormat>\n      <Units>_V</Units>\n      <TestTime></TestTime>\n    </Test>\n    <Test>\n      <Code>10.33</Code>\n      <Name>SELECTOR_16_L</Name>\n      <Description></Description>\n      <Group>Pin_Tests</Group>\n      <IsGroup>No</IsGroup>\n      <Tag>Pin_Tests:SELECTOR_16_L</Tag>\n      <Method>Test_Pin_N_Low</Method>\n      <Parameter>CH16</Parameter>\n      <DataType>Dbl</DataType>\n      <Value></Value>\n      <Status></Status>\n      <LimitLo>0</LimitLo>\n      <LimitHi>0.01</LimitHi>\n      <StringMatch></StringMatch>\n      <BooleanMatch></BooleanMatch>\n      <DisplayFormat>%.2f</DisplayFormat>\n      <Units>_V</Units>\n      <TestTime></TestTime>\n    </Test>\n    <Test>\n      <Code>10.34</Code>\n      <Name>SELECTOR_17_H</Name>\n      <Description></Description>\n      <Group>Pin_Tests</Group>\n      <IsGroup>No</IsGroup>\n      <Tag>Pin_Tests:SELECTOR_17_H</Tag>\n      <Method>Test_Pin_N_High</Method>\n      <Parameter>CH17</Parameter>\n      <DataType>Dbl</DataType>\n      <Value></Value>\n      <Status></Status>\n      <LimitLo>3.2</LimitLo>\n      <LimitHi>3.4</LimitHi>\n      <StringMatch></StringMatch>\n      <BooleanMatch></BooleanMatch>\n      <DisplayFormat>%.2f</DisplayFormat>\n      <Units>_V</Units>\n      <TestTime></TestTime>\n    </Test>\n    <Test>\n      <Code>10.35</Code>\n      <Name>SELECTOR_17_L</Name>\n      <Description></Description>\n      <Group>Pin_Tests</Group>\n      <IsGroup>No</IsGroup>\n      <Tag>Pin_Tests:SELECTOR_17_L</Tag>\n      <Method>Test_Pin_N_Low</Method>\n      <Parameter>CH17</Parameter>\n      <DataType>Dbl</DataType>\n      <Value></Value>\n      <Status></Status>\n      <LimitLo>0</LimitLo>\n      <LimitHi>0.01</LimitHi>\n      <StringMatch></StringMatch>\n      <BooleanMatch></BooleanMatch>\n      <DisplayFormat>%.2f</DisplayFormat>\n      <Units>_V</Units>\n      <TestTime></TestTime>\n    </Test>\n    <Test>\n      <Code>10.36</Code>\n      <Name>SELECTOR_18_H</Name>\n      <Description></Description>\n      <Group>Pin_Tests</Group>\n      <IsGroup>No</IsGroup>\n      <Tag>Pin_Tests:SELECTOR_18_H</Tag>\n      <Method>Test_Pin_N_High</Method>\n      <Parameter>CH18</Parameter>\n      <DataType>Dbl</DataType>\n      <Value></Value>\n      <Status></Status>\n      <LimitLo>3.2</LimitLo>\n      <LimitHi>3.4</LimitHi>\n      <StringMatch></StringMatch>\n      <BooleanMatch></BooleanMatch>\n      <DisplayFormat>%.2f</DisplayFormat>\n      <Units>_V</Units>\n      <TestTime></TestTime>\n    </Test>\n    <Test>\n      <Code>10.37</Code>\n      <Name>SELECTOR_18_L</Name>\n      <Description></Description>\n      <Group>Pin_Tests</Group>\n      <IsGroup>No</IsGroup>\n      <Tag>Pin_Tests:SELECTOR_18_L</Tag>\n      <Method>Test_Pin_N_Low</Method>\n      <Parameter>CH18</Parameter>\n      <DataType>Dbl</DataType>\n      <Value></Value>\n      <Status></Status>\n      <LimitLo>0</LimitLo>\n      <LimitHi>0.01</LimitHi>\n      <StringMatch></StringMatch>\n      <BooleanMatch></BooleanMatch>\n      <DisplayFormat>%.2f</DisplayFormat>\n      <Units>_V</Units>\n      <TestTime></TestTime>\n    </Test>\n    <Test>\n      <Code>10.38</Code>\n      <Name>SELECTOR_19_H</Name>\n      <Description></Description>\n      <Group>Pin_Tests</Group>\n      <IsGroup>No</IsGroup>\n      <Tag>Pin_Tests:SELECTOR_19_H</Tag>\n      <Method>Test_Pin_N_High</Method>\n      <Parameter>CH19</Parameter>\n      <DataType>Dbl</DataType>\n      <Value></Value>\n      <Status></Status>\n      <LimitLo>3.2</LimitLo>\n      <LimitHi>3.4</LimitHi>\n      <StringMatch></StringMatch>\n      <BooleanMatch></BooleanMatch>\n      <DisplayFormat>%.2f</DisplayFormat>\n      <Units>_V</Units>\n      <TestTime></TestTime>\n    </Test>\n    <Test>\n      <Code>10.39</Code>\n      <Name>SELECTOR_19_L</Name>\n      <Description></Description>\n      <Group>Pin_Tests</Group>\n      <IsGroup>No</IsGroup>\n      <Tag>Pin_Tests:SELECTOR_19_L</Tag>\n      <Method>Test_Pin_N_Low</Method>\n      <Parameter>CH19</Parameter>\n      <DataType>Dbl</DataType>\n      <Value></Value>\n      <Status></Status>\n      <LimitLo>0</LimitLo>\n      <LimitHi>0.01</LimitHi>\n      <StringMatch></StringMatch>\n      <BooleanMatch></BooleanMatch>\n      <DisplayFormat>%.2f</DisplayFormat>\n      <Units>_V</Units>\n      <TestTime></TestTime>\n    </Test>\n    <Test>\n      <Code>10.40</Code>\n      <Name>SELECTOR_20_H</Name>\n      <Description></Description>\n      <Group>Pin_Tests</Group>\n      <IsGroup>No</IsGroup>\n      <Tag>Pin_Tests:SELECTOR_20_H</Tag>\n      <Method>Test_Pin_N_High</Method>\n      <Parameter>CH20</Parameter>\n      <DataType>Dbl</DataType>\n      <Value></Value>\n      <Status></Status>\n      <LimitLo>3.2</LimitLo>\n      <LimitHi>3.4</LimitHi>\n      <StringMatch></StringMatch>\n      <BooleanMatch></BooleanMatch>\n      <DisplayFormat>%.2f</DisplayFormat>\n      <Units>_V</Units>\n      <TestTime></TestTime>\n    </Test>\n    <Test>\n      <Code>10.41</Code>\n      <Name>SELECTOR_20_L</Name>\n      <Description></Description>\n      <Group>Pin_Tests</Group>\n      <IsGroup>No</IsGroup>\n      <Tag>Pin_Tests:SELECTOR_20_L</Tag>\n      <Method>Test_Pin_N_Low</Method>\n      <Parameter>CH20</Parameter>\n      <DataType>Dbl</DataType>\n      <Value></Value>\n      <Status></Status>\n      <LimitLo>0</LimitLo>\n      <LimitHi>0.01</LimitHi>\n      <StringMatch></StringMatch>\n      <BooleanMatch></BooleanMatch>\n      <DisplayFormat>%.2f</DisplayFormat>\n      <Units>_V</Units>\n      <TestTime></TestTime>\n    </Test>\n    <Test>\n      <Code>10.42</Code>\n      <Name>SELECTOR_21_H</Name>\n      <Description></Description>\n      <Group>Pin_Tests</Group>\n      <IsGroup>No</IsGroup>\n      <Tag>Pin_Tests:SELECTOR_21_H</Tag>\n      <Method>Test_Pin_N_High</Method>\n      <Parameter>CH21</Parameter>\n      <DataType>Dbl</DataType>\n      <Value></Value>\n      <Status></Status>\n      <LimitLo>3.2</LimitLo>\n      <LimitHi>3.4</LimitHi>\n      <StringMatch></StringMatch>\n      <BooleanMatch></BooleanMatch>\n      <DisplayFormat>%.2f</DisplayFormat>\n      <Units>_V</Units>\n      <TestTime></TestTime>\n    </Test>\n    <Test>\n      <Code>10.43</Code>\n      <Name>SELECTOR_21_L</Name>\n      <Description></Description>\n      <Group>Pin_Tests</Group>\n      <IsGroup>No</IsGroup>\n      <Tag>Pin_Tests:SELECTOR_21_L</Tag>\n      <Method>Test_Pin_N_Low</Method>\n      <Parameter>CH21</Parameter>\n      <DataType>Dbl</DataType>\n      <Value></Value>\n      <Status></Status>\n      <LimitLo>0</LimitLo>\n      <LimitHi>0.01</LimitHi>\n      <StringMatch></StringMatch>\n      <BooleanMatch></BooleanMatch>\n      <DisplayFormat>%.2f</DisplayFormat>\n      <Units>_V</Units>\n      <TestTime></TestTime>\n    </Test>\n    <Test>\n      <Code>10.44</Code>\n      <Name>SELECTOR_22_H</Name>\n      <Description></Description>\n      <Group>Pin_Tests</Group>\n      <IsGroup>No</IsGroup>\n      <Tag>Pin_Tests:SELECTOR_22_H</Tag>\n      <Method>Test_Pin_N_High</Method>\n      <Parameter>CH22</Parameter>\n      <DataType>Dbl</DataType>\n      <Value></Value>\n      <Status></Status>\n      <LimitLo>3.2</LimitLo>\n      <LimitHi>3.4</LimitHi>\n      <StringMatch></StringMatch>\n      <BooleanMatch></BooleanMatch>\n      <DisplayFormat>%.2f</DisplayFormat>\n      <Units>_V</Units>\n      <TestTime></TestTime>\n    </Test>\n    <Test>\n      <Code>10.45</Code>\n      <Name>SELECTOR_22_L</Name>\n      <Description></Description>\n      <Group>Pin_Tests</Group>\n      <IsGroup>No</IsGroup>\n      <Tag>Pin_Tests:SELECTOR_22_L</Tag>\n      <Method>Test_Pin_N_Low</Method>\n      <Parameter>CH22</Parameter>\n      <DataType>Dbl</DataType>\n      <Value></Value>\n      <Status></Status>\n      <LimitLo>0</LimitLo>\n      <LimitHi>0.01</LimitHi>\n      <StringMatch></StringMatch>\n      <BooleanMatch></BooleanMatch>\n      <DisplayFormat>%.2f</DisplayFormat>\n      <Units>_V</Units>\n      <TestTime></TestTime>\n    </Test>\n    <Test>\n      <Code>10.46</Code>\n      <Name>SELECTOR_23_H</Name>\n      <Description></Description>\n      <Group>Pin_Tests</Group>\n      <IsGroup>No</IsGroup>\n      <Tag>Pin_Tests:SELECTOR_23_H</Tag>\n      <Method>Test_Pin_N_High</Method>\n      <Parameter>CH23</Parameter>\n      <DataType>Dbl</DataType>\n      <Value></Value>\n      <Status></Status>\n      <LimitLo>3.2</LimitLo>\n      <LimitHi>3.4</LimitHi>\n      <StringMatch></StringMatch>\n      <BooleanMatch></BooleanMatch>\n      <DisplayFormat>%.2f</DisplayFormat>\n      <Units>_V</Units>\n      <TestTime></TestTime>\n    </Test>\n    <Test>\n      <Code>10.47</Code>\n      <Name>SELECTOR_23_L</Name>\n      <Description></Description>\n      <Group>Pin_Tests</Group>\n      <IsGroup>No</IsGroup>\n      <Tag>Pin_Tests:SELECTOR_23_L</Tag>\n      <Method>Test_Pin_N_Low</Method>\n      <Parameter>CH23</Parameter>\n      <DataType>Dbl</DataType>\n      <Value></Value>\n      <Status></Status>\n      <LimitLo>0</LimitLo>\n      <LimitHi>0.01</LimitHi>\n      <StringMatch></StringMatch>\n      <BooleanMatch></BooleanMatch>\n      <DisplayFormat>%.2f</DisplayFormat>\n      <Units>_V</Units>\n      <TestTime></TestTime>\n    </Test>\n    <Test>\n      <Code>10.48</Code>\n      <Name>SELECTOR_24_H</Name>\n      <Description></Description>\n      <Group>Pin_Tests</Group>\n      <IsGroup>No</IsGroup>\n      <Tag>Pin_Tests:SELECTOR_24_H</Tag>\n      <Method>Test_Pin_N_High</Method>\n      <Parameter>CH24</Parameter>\n      <DataType>Dbl</DataType>\n      <Value></Value>\n      <Status></Status>\n      <LimitLo>3.2</LimitLo>\n      <LimitHi>3.4</LimitHi>\n      <StringMatch></StringMatch>\n      <BooleanMatch></BooleanMatch>\n      <DisplayFormat>%.2f</DisplayFormat>\n      <Units>_V</Units>\n      <TestTime></TestTime>\n    </Test>\n    <Test>\n      <Code>10.49</Code>\n      <Name>SELECTOR_24_L</Name>\n      <Description></Description>\n      <Group>Pin_Tests</Group>\n      <IsGroup>No</IsGroup>\n      <Tag>Pin_Tests:SELECTOR_24_L</Tag>\n      <Method>Test_Pin_N_Low</Method>\n      <Parameter>CH24</Parameter>\n      <DataType>Dbl</DataType>\n      <Value></Value>\n      <Status></Status>\n      <LimitLo>0</LimitLo>\n      <LimitHi>0.01</LimitHi>\n      <StringMatch></StringMatch>\n      <BooleanMatch></BooleanMatch>\n      <DisplayFormat>%.2f</DisplayFormat>\n      <Units>_V</Units>\n      <TestTime></TestTime>\n    </Test>\n    <Test>\n      <Code>10.50</Code>\n      <Name>SELECTOR_25_H</Name>\n      <Description></Description>\n      <Group>Pin_Tests</Group>\n      <IsGroup>No</IsGroup>\n      <Tag>Pin_Tests:SELECTOR_25_H</Tag>\n      <Method>Test_Pin_N_High</Method>\n      <Parameter>CH25</Parameter>\n      <DataType>Dbl</DataType>\n      <Value></Value>\n      <Status></Status>\n      <LimitLo>3.2</LimitLo>\n      <LimitHi>3.4</LimitHi>\n      <StringMatch></StringMatch>\n      <BooleanMatch></BooleanMatch>\n      <DisplayFormat>%.2f</DisplayFormat>\n      <Units>_V</Units>\n      <TestTime></TestTime>\n    </Test>\n    <Test>\n      <Code>10.51</Code>\n      <Name>SELECTOR_25_L</Name>\n      <Description></Description>\n      <Group>Pin_Tests</Group>\n      <IsGroup>No</IsGroup>\n      <Tag>Pin_Tests:SELECTOR_25_L</Tag>\n      <Method>Test_Pin_N_Low</Method>\n      <Parameter>CH25</Parameter>\n      <DataType>Dbl</DataType>\n      <Value></Value>\n      <Status></Status>\n      <LimitLo>0</LimitLo>\n      <LimitHi>0.01</LimitHi>\n      <StringMatch></StringMatch>\n      <BooleanMatch></BooleanMatch>\n      <DisplayFormat>%.2f</DisplayFormat>\n      <Units>_V</Units>\n      <TestTime></TestTime>\n    </Test>\n    <Test>\n      <Code>10.52</Code>\n      <Name>SELECTOR_26_H</Name>\n      <Description></Description>\n      <Group>Pin_Tests</Group>\n      <IsGroup>No</IsGroup>\n      <Tag>Pin_Tests:SELECTOR_26_H</Tag>\n      <Method>Test_Pin_N_High</Method>\n      <Parameter>CH26</Parameter>\n      <DataType>Dbl</DataType>\n      <Value></Value>\n      <Status></Status>\n      <LimitLo>3.2</LimitLo>\n      <LimitHi>3.4</LimitHi>\n      <StringMatch></StringMatch>\n      <BooleanMatch></BooleanMatch>\n      <DisplayFormat>%.2f</DisplayFormat>\n      <Units>_V</Units>\n      <TestTime></TestTime>\n    </Test>\n    <Test>\n      <Code>10.53</Code>\n      <Name>SELECTOR_26_L</Name>\n      <Description></Description>\n      <Group>Pin_Tests</Group>\n      <IsGroup>No</IsGroup>\n      <Tag>Pin_Tests:SELECTOR_26_L</Tag>\n      <Method>Test_Pin_N_Low</Method>\n      <Parameter>CH26</Parameter>\n      <DataType>Dbl</DataType>\n      <Value></Value>\n      <Status></Status>\n      <LimitLo>0</LimitLo>\n      <LimitHi>0.01</LimitHi>\n      <StringMatch></StringMatch>\n      <BooleanMatch></BooleanMatch>\n      <DisplayFormat>%.2f</DisplayFormat>\n      <Units>_V</Units>\n      <TestTime></TestTime>\n    </Test>\n    <Test>\n      <Code>10.54</Code>\n      <Name>SELECTOR_27_H</Name>\n      <Description></Description>\n      <Group>Pin_Tests</Group>\n      <IsGroup>No</IsGroup>\n      <Tag>Pin_Tests:SELECTOR_27_H</Tag>\n      <Method>Test_Pin_N_High</Method>\n      <Parameter>CH27</Parameter>\n      <DataType>Dbl</DataType>\n      <Value></Value>\n      <Status></Status>\n      <LimitLo>3.2</LimitLo>\n      <LimitHi>3.4</LimitHi>\n      <StringMatch></StringMatch>\n      <BooleanMatch></BooleanMatch>\n      <DisplayFormat>%.2f</DisplayFormat>\n      <Units>_V</Units>\n      <TestTime></TestTime>\n    </Test>\n    <Test>\n      <Code>10.55</Code>\n      <Name>SELECTOR_27_L</Name>\n      <Description></Description>\n      <Group>Pin_Tests</Group>\n      <IsGroup>No</IsGroup>\n      <Tag>Pin_Tests:SELECTOR_27_L</Tag>\n      <Method>Test_Pin_N_Low</Method>\n      <Parameter>CH27</Parameter>\n      <DataType>Dbl</DataType>\n      <Value></Value>\n      <Status></Status>\n      <LimitLo>0</LimitLo>\n      <LimitHi>0.01</LimitHi>\n      <StringMatch></StringMatch>\n      <BooleanMatch></BooleanMatch>\n      <DisplayFormat>%.2f</DisplayFormat>\n      <Units>_V</Units>\n      <TestTime></TestTime>\n    </Test>\n    <Test>\n      <Code>10.56</Code>\n      <Name>SELECTOR_28_H</Name>\n      <Description></Description>\n      <Group>Pin_Tests</Group>\n      <IsGroup>No</IsGroup>\n      <Tag>Pin_Tests:SELECTOR_28_H</Tag>\n      <Method>Test_Pin_N_High</Method>\n      <Parameter>CH28</Parameter>\n      <DataType>Dbl</DataType>\n      <Value></Value>\n      <Status></Status>\n      <LimitLo>3.2</LimitLo>\n      <LimitHi>3.4</LimitHi>\n      <StringMatch></StringMatch>\n      <BooleanMatch></BooleanMatch>\n      <DisplayFormat>%.2f</DisplayFormat>\n      <Units>_V</Units>\n      <TestTime></TestTime>\n    </Test>\n    <Test>\n      <Code>10.57</Code>\n      <Name>SELECTOR_28_L</Name>\n      <Description></Description>\n      <Group>Pin_Tests</Group>\n      <IsGroup>No</IsGroup>\n      <Tag>Pin_Tests:SELECTOR_28_L</Tag>\n      <Method>Test_Pin_N_Low</Method>\n      <Parameter>CH28</Parameter>\n      <DataType>Dbl</DataType>\n      <Value></Value>\n      <Status></Status>\n      <LimitLo>0</LimitLo>\n      <LimitHi>0.01</LimitHi>\n      <StringMatch></StringMatch>\n      <BooleanMatch></BooleanMatch>\n      <DisplayFormat>%.2f</DisplayFormat>\n      <Units>_V</Units>\n      <TestTime></TestTime>\n    </Test>\n    <Test>\n      <Code>10.58</Code>\n      <Name>SELECTOR_29_H</Name>\n      <Description></Description>\n      <Group>Pin_Tests</Group>\n      <IsGroup>No</IsGroup>\n      <Tag>Pin_Tests:SELECTOR_29_H</Tag>\n      <Method>Test_Pin_N_High</Method>\n      <Parameter>CH29</Parameter>\n      <DataType>Dbl</DataType>\n      <Value></Value>\n      <Status></Status>\n      <LimitLo>3.2</LimitLo>\n      <LimitHi>3.4</LimitHi>\n      <StringMatch></StringMatch>\n      <BooleanMatch></BooleanMatch>\n      <DisplayFormat>%.2f</DisplayFormat>\n      <Units>_V</Units>\n      <TestTime></TestTime>\n    </Test>\n    <Test>\n      <Code>10.59</Code>\n      <Name>SELECTOR_29_L</Name>\n      <Description></Description>\n      <Group>Pin_Tests</Group>\n      <IsGroup>No</IsGroup>\n      <Tag>Pin_Tests:SELECTOR_29_L</Tag>\n      <Method>Test_Pin_N_Low</Method>\n      <Parameter>CH29</Parameter>\n      <DataType>Dbl</DataType>\n      <Value></Value>\n      <Status></Status>\n      <LimitLo>0</LimitLo>\n      <LimitHi>0.01</LimitHi>\n      <StringMatch></StringMatch>\n      <BooleanMatch></BooleanMatch>\n      <DisplayFormat>%.2f</DisplayFormat>\n      <Units>_V</Units>\n      <TestTime></TestTime>\n    </Test>\n    <Test>\n      <Code>10.60</Code>\n      <Name>SELECTOR_30_H</Name>\n      <Description></Description>\n      <Group>Pin_Tests</Group>\n      <IsGroup>No</IsGroup>\n      <Tag>Pin_Tests:SELECTOR_30_H</Tag>\n      <Method>Test_Pin_N_High</Method>\n      <Parameter>CH30</Parameter>\n      <DataType>Dbl</DataType>\n      <Value></Value>\n      <Status></Status>\n      <LimitLo>3.2</LimitLo>\n      <LimitHi>3.4</LimitHi>\n      <StringMatch></StringMatch>\n      <BooleanMatch></BooleanMatch>\n      <DisplayFormat>%.2f</DisplayFormat>\n      <Units>_V</Units>\n      <TestTime></TestTime>\n    </Test>\n    <Test>\n      <Code>10.61</Code>\n      <Name>SELECTOR_30_L</Name>\n      <Description></Description>\n      <Group>Pin_Tests</Group>\n      <IsGroup>No</IsGroup>\n      <Tag>Pin_Tests:SELECTOR_30_L</Tag>\n      <Method>Test_Pin_N_Low</Method>\n      <Parameter>CH30</Parameter>\n      <DataType>Dbl</DataType>\n      <Value></Value>\n      <Status></Status>\n      <LimitLo>0</LimitLo>\n      <LimitHi>0.01</LimitHi>\n      <StringMatch></StringMatch>\n      <BooleanMatch></BooleanMatch>\n      <DisplayFormat>%.2f</DisplayFormat>\n      <Units>_V</Units>\n      <TestTime></TestTime>\n    </Test>\n    <Test>\n      <Code>10.62</Code>\n      <Name>SELECTOR_31_H</Name>\n      <Description></Description>\n      <Group>Pin_Tests</Group>\n      <IsGroup>No</IsGroup>\n      <Tag>Pin_Tests:SELECTOR_31_H</Tag>\n      <Method>Test_Pin_N_High</Method>\n      <Parameter>CH31</Parameter>\n      <DataType>Dbl</DataType>\n      <Value></Value>\n      <Status></Status>\n      <LimitLo>3.2</LimitLo>\n      <LimitHi>3.4</LimitHi>\n      <StringMatch></StringMatch>\n      <BooleanMatch></BooleanMatch>\n      <DisplayFormat>%.2f</DisplayFormat>\n      <Units>_V</Units>\n      <TestTime></TestTime>\n    </Test>\n    <Test>\n      <Code>10.63</Code>\n      <Name>SELECTOR_31_L</Name>\n      <Description></Description>\n      <Group>Pin_Tests</Group>\n      <IsGroup>No</IsGroup>\n      <Tag>Pin_Tests:SELECTOR_31_L</Tag>\n      <Method>Test_Pin_N_Low</Method>\n      <Parameter>CH31</Parameter>\n      <DataType>Dbl</DataType>\n      <Value></Value>\n      <Status></Status>\n      <LimitLo>0</LimitLo>\n      <LimitHi>0.01</LimitHi>\n      <StringMatch></StringMatch>\n      <BooleanMatch></BooleanMatch>\n      <DisplayFormat>%.2f</DisplayFormat>\n      <Units>_V</Units>\n      <TestTime></TestTime>\n    </Test>\n    <Test>\n      <Code>10.64</Code>\n      <Name>SELECTOR_32_H</Name>\n      <Description></Description>\n      <Group>Pin_Tests</Group>\n      <IsGroup>No</IsGroup>\n      <Tag>Pin_Tests:SELECTOR_32_H</Tag>\n      <Method>Test_Pin_N_High</Method>\n      <Parameter>CH32</Parameter>\n      <DataType>Dbl</DataType>\n      <Value></Value>\n      <Status></Status>\n      <LimitLo>3.2</LimitLo>\n      <LimitHi>3.4</LimitHi>\n      <StringMatch></StringMatch>\n      <BooleanMatch></BooleanMatch>\n      <DisplayFormat>%.2f</DisplayFormat>\n      <Units>_V</Units>\n      <TestTime></TestTime>\n    </Test>\n    <Test>\n      <Code>10.65</Code>\n      <Name>SELECTOR_32_L</Name>\n      <Description></Description>\n      <Group>Pin_Tests</Group>\n      <IsGroup>No</IsGroup>\n      <Tag>Pin_Tests:SELECTOR_32_L</Tag>\n      <Method>Test_Pin_N_Low</Method>\n      <Parameter>CH32</Parameter>\n      <DataType>Dbl</DataType>\n      <Value></Value>\n      <Status></Status>\n      <LimitLo>0</LimitLo>\n      <LimitHi>0.01</LimitHi>\n      <StringMatch></StringMatch>\n      <BooleanMatch></BooleanMatch>\n      <DisplayFormat>%.2f</DisplayFormat>\n      <Units>_V</Units>\n      <TestTime></TestTime>\n    </Test>\n    <Test>\n      <Code>10.66</Code>\n      <Name>SELECTOR_33_H</Name>\n      <Description></Description>\n      <Group>Pin_Tests</Group>\n      <IsGroup>No</IsGroup>\n      <Tag>Pin_Tests:SELECTOR_33_H</Tag>\n      <Method>Test_Pin_N_High</Method>\n      <Parameter>CH33</Parameter>\n      <DataType>Dbl</DataType>\n      <Value></Value>\n      <Status></Status>\n      <LimitLo>3.2</LimitLo>\n      <LimitHi>3.4</LimitHi>\n      <StringMatch></StringMatch>\n      <BooleanMatch></BooleanMatch>\n      <DisplayFormat>%.2f</DisplayFormat>\n      <Units>_V</Units>\n      <TestTime></TestTime>\n    </Test>\n    <Test>\n      <Code>10.67</Code>\n      <Name>SELECTOR_33_L</Name>\n      <Description></Description>\n      <Group>Pin_Tests</Group>\n      <IsGroup>No</IsGroup>\n      <Tag>Pin_Tests:SELECTOR_33_L</Tag>\n      <Method>Test_Pin_N_Low</Method>\n      <Parameter>CH33</Parameter>\n      <DataType>Dbl</DataType>\n      <Value></Value>\n      <Status></Status>\n      <LimitLo>0</LimitLo>\n      <LimitHi>0.01</LimitHi>\n      <StringMatch></StringMatch>\n      <BooleanMatch></BooleanMatch>\n      <DisplayFormat>%.2f</DisplayFormat>\n      <Units>_V</Units>\n      <TestTime></TestTime>\n    </Test>\n    <Test>\n      <Code>10.68</Code>\n      <Name>SELECTOR_34_H</Name>\n      <Description></Description>\n      <Group>Pin_Tests</Group>\n      <IsGroup>No</IsGroup>\n      <Tag>Pin_Tests:SELECTOR_34_H</Tag>\n      <Method>Test_Pin_N_High</Method>\n      <Parameter>CH34</Parameter>\n      <DataType>Dbl</DataType>\n      <Value></Value>\n      <Status></Status>\n      <LimitLo>3.2</LimitLo>\n      <LimitHi>3.4</LimitHi>\n      <StringMatch></StringMatch>\n      <BooleanMatch></BooleanMatch>\n      <DisplayFormat>%.2f</DisplayFormat>\n      <Units>_V</Units>\n      <TestTime></TestTime>\n    </Test>\n    <Test>\n      <Code>10.69</Code>\n      <Name>SELECTOR_34_L</Name>\n      <Description></Description>\n      <Group>Pin_Tests</Group>\n      <IsGroup>No</IsGroup>\n      <Tag>Pin_Tests:SELECTOR_34_L</Tag>\n      <Method>Test_Pin_N_Low</Method>\n      <Parameter>CH34</Parameter>\n      <DataType>Dbl</DataType>\n      <Value></Value>\n      <Status></Status>\n      <LimitLo>0</LimitLo>\n      <LimitHi>0.01</LimitHi>\n      <StringMatch></StringMatch>\n      <BooleanMatch></BooleanMatch>\n      <DisplayFormat>%.2f</DisplayFormat>\n      <Units>_V</Units>\n      <TestTime></TestTime>\n    </Test>\n    <Test>\n      <Code>10.70</Code>\n      <Name>SELECTOR_35_H</Name>\n      <Description></Description>\n      <Group>Pin_Tests</Group>\n      <IsGroup>No</IsGroup>\n      <Tag>Pin_Tests:SELECTOR_35_H</Tag>\n      <Method>Test_Pin_N_High</Method>\n      <Parameter>CH35</Parameter>\n      <DataType>Dbl</DataType>\n      <Value></Value>\n      <Status></Status>\n      <LimitLo>3.2</LimitLo>\n      <LimitHi>3.4</LimitHi>\n      <StringMatch></StringMatch>\n      <BooleanMatch></BooleanMatch>\n      <DisplayFormat>%.2f</DisplayFormat>\n      <Units>_V</Units>\n      <TestTime></TestTime>\n    </Test>\n    <Test>\n      <Code>10.71</Code>\n      <Name>SELECTOR_35_L</Name>\n      <Description></Description>\n      <Group>Pin_Tests</Group>\n      <IsGroup>No</IsGroup>\n      <Tag>Pin_Tests:SELECTOR_35_L</Tag>\n      <Method>Test_Pin_N_Low</Method>\n      <Parameter>CH35</Parameter>\n      <DataType>Dbl</DataType>\n      <Value></Value>\n      <Status></Status>\n      <LimitLo>0</LimitLo>\n      <LimitHi>0.01</LimitHi>\n      <StringMatch></StringMatch>\n      <BooleanMatch></BooleanMatch>\n      <DisplayFormat>%.2f</DisplayFormat>\n      <Units>_V</Units>\n      <TestTime></TestTime>\n    </Test>\n    <Test>\n      <Code>10.72</Code>\n      <Name>SELECTOR_36_H</Name>\n      <Description></Description>\n      <Group>Pin_Tests</Group>\n      <IsGroup>No</IsGroup>\n      <Tag>Pin_Tests:SELECTOR_36_H</Tag>\n      <Method>Test_Pin_N_High</Method>\n      <Parameter>CH36</Parameter>\n      <DataType>Dbl</DataType>\n      <Value></Value>\n      <Status></Status>\n      <LimitLo>3.2</LimitLo>\n      <LimitHi>3.4</LimitHi>\n      <StringMatch></StringMatch>\n      <BooleanMatch></BooleanMatch>\n      <DisplayFormat>%.2f</DisplayFormat>\n      <Units>_V</Units>\n      <TestTime></TestTime>\n    </Test>\n    <Test>\n      <Code>10.73</Code>\n      <Name>SELECTOR_36_L</Name>\n      <Description></Description>\n      <Group>Pin_Tests</Group>\n      <IsGroup>No</IsGroup>\n      <Tag>Pin_Tests:SELECTOR_36_L</Tag>\n      <Method>Test_Pin_N_Low</Method>\n      <Parameter>CH36</Parameter>\n      <DataType>Dbl</DataType>\n      <Value></Value>\n      <Status></Status>\n      <LimitLo>0</LimitLo>\n      <LimitHi>0.01</LimitHi>\n      <StringMatch></StringMatch>\n      <BooleanMatch></BooleanMatch>\n      <DisplayFormat>%.2f</DisplayFormat>\n      <Units>_V</Units>\n      <TestTime></TestTime>\n    </Test>\n    <Test>\n      <Code>10.74</Code>\n      <Name>SELECTOR_37_H</Name>\n      <Description></Description>\n      <Group>Pin_Tests</Group>\n      <IsGroup>No</IsGroup>\n      <Tag>Pin_Tests:SELECTOR_37_H</Tag>\n      <Method>Test_Pin_N_High</Method>\n      <Parameter>CH37</Parameter>\n      <DataType>Dbl</DataType>\n      <Value></Value>\n      <Status></Status>\n      <LimitLo>3.2</LimitLo>\n      <LimitHi>3.4</LimitHi>\n      <StringMatch></StringMatch>\n      <BooleanMatch></BooleanMatch>\n      <DisplayFormat>%.2f</DisplayFormat>\n      <Units>_V</Units>\n      <TestTime></TestTime>\n    </Test>\n    <Test>\n      <Code>10.75</Code>\n      <Name>SELECTOR_37_L</Name>\n      <Description></Description>\n      <Group>Pin_Tests</Group>\n      <IsGroup>No</IsGroup>\n      <Tag>Pin_Tests:SELECTOR_37_L</Tag>\n      <Method>Test_Pin_N_Low</Method>\n      <Parameter>CH37</Parameter>\n      <DataType>Dbl</DataType>\n      <Value></Value>\n      <Status></Status>\n      <LimitLo>0</LimitLo>\n      <LimitHi>0.01</LimitHi>\n      <StringMatch></StringMatch>\n      <BooleanMatch></BooleanMatch>\n      <DisplayFormat>%.2f</DisplayFormat>\n      <Units>_V</Units>\n      <TestTime></TestTime>\n    </Test>\n    <Test>\n      <Code>10.76</Code>\n      <Name>SELECTOR_38_H</Name>\n      <Description></Description>\n      <Group>Pin_Tests</Group>\n      <IsGroup>No</IsGroup>\n      <Tag>Pin_Tests:SELECTOR_38_H</Tag>\n      <Method>Test_Pin_N_High</Method>\n      <Parameter>CH38</Parameter>\n      <DataType>Dbl</DataType>\n      <Value></Value>\n      <Status></Status>\n      <LimitLo>3.2</LimitLo>\n      <LimitHi>3.4</LimitHi>\n      <StringMatch></StringMatch>\n      <BooleanMatch></BooleanMatch>\n      <DisplayFormat>%.2f</DisplayFormat>\n      <Units>_V</Units>\n      <TestTime></TestTime>\n    </Test>\n    <Test>\n      <Code>10.77</Code>\n      <Name>SELECTOR_38_L</Name>\n      <Description></Description>\n      <Group>Pin_Tests</Group>\n      <IsGroup>No</IsGroup>\n      <Tag>Pin_Tests:SELECTOR_38_L</Tag>\n      <Method>Test_Pin_N_Low</Method>\n      <Parameter>CH38</Parameter>\n      <DataType>Dbl</DataType>\n      <Value></Value>\n      <Status></Status>\n      <LimitLo>0</LimitLo>\n      <LimitHi>0.01</LimitHi>\n      <StringMatch></StringMatch>\n      <BooleanMatch></BooleanMatch>\n      <DisplayFormat>%.2f</DisplayFormat>\n      <Units>_V</Units>\n      <TestTime></TestTime>\n    </Test>\n    <Test>\n      <Code>10.78</Code>\n      <Name>SELECTOR_39_H</Name>\n      <Description></Description>\n      <Group>Pin_Tests</Group>\n      <IsGroup>No</IsGroup>\n      <Tag>Pin_Tests:SELECTOR_39_H</Tag>\n      <Method>Test_Pin_N_High</Method>\n      <Parameter>CH39</Parameter>\n      <DataType>Dbl</DataType>\n      <Value></Value>\n      <Status></Status>\n      <LimitLo>3.2</LimitLo>\n      <LimitHi>3.4</LimitHi>\n      <StringMatch></StringMatch>\n      <BooleanMatch></BooleanMatch>\n      <DisplayFormat>%.2f</DisplayFormat>\n      <Units>_V</Units>\n      <TestTime></TestTime>\n    </Test>\n    <Test>\n      <Code>10.79</Code>\n      <Name>SELECTOR_39_L</Name>\n      <Description></Description>\n      <Group>Pin_Tests</Group>\n      <IsGroup>No</IsGroup>\n      <Tag>Pin_Tests:SELECTOR_39_L</Tag>\n      <Method>Test_Pin_N_Low</Method>\n      <Parameter>CH39</Parameter>\n      <DataType>Dbl</DataType>\n      <Value></Value>\n      <Status></Status>\n      <LimitLo>0</LimitLo>\n      <LimitHi>0.01</LimitHi>\n      <StringMatch></StringMatch>\n      <BooleanMatch></BooleanMatch>\n      <DisplayFormat>%.2f</DisplayFormat>\n      <Units>_V</Units>\n      <TestTime></TestTime>\n    </Test>\n    <Test>\n      <Code>10.80</Code>\n      <Name>SELECTOR_40_H</Name>\n      <Description></Description>\n      <Group>Pin_Tests</Group>\n      <IsGroup>No</IsGroup>\n      <Tag>Pin_Tests:SELECTOR_40_H</Tag>\n      <Method>Test_Pin_N_High</Method>\n      <Parameter>CH40</Parameter>\n      <DataType>Dbl</DataType>\n      <Value></Value>\n      <Status></Status>\n      <LimitLo>3.2</LimitLo>\n      <LimitHi>3.4</LimitHi>\n      <StringMatch></StringMatch>\n      <BooleanMatch></BooleanMatch>\n      <DisplayFormat>%.2f</DisplayFormat>\n      <Units>_V</Units>\n      <TestTime></TestTime>\n    </Test>\n    <Test>\n      <Code>10.81</Code>\n      <Name>SELECTOR_40_L</Name>\n      <Description></Description>\n      <Group>Pin_Tests</Group>\n      <IsGroup>No</IsGroup>\n      <Tag>Pin_Tests:SELECTOR_40_L</Tag>\n      <Method>Test_Pin_N_Low</Method>\n      <Parameter>CH40</Parameter>\n      <DataType>Dbl</DataType>\n      <Value></Value>\n      <Status></Status>\n      <LimitLo>0</LimitLo>\n      <LimitHi>0.01</LimitHi>\n      <StringMatch></StringMatch>\n      <BooleanMatch></BooleanMatch>\n      <DisplayFormat>%.2f</DisplayFormat>\n      <Units>_V</Units>\n      <TestTime></TestTime>\n    </Test>\n    <Test>\n      <Code>10.82</Code>\n      <Name>SELECTOR_41_H</Name>\n      <Description></Description>\n      <Group>Pin_Tests</Group>\n      <IsGroup>No</IsGroup>\n      <Tag>Pin_Tests:SELECTOR_41_H</Tag>\n      <Method>Test_Pin_N_High</Method>\n      <Parameter>CH41</Parameter>\n      <DataType>Dbl</DataType>\n      <Value></Value>\n      <Status></Status>\n      <LimitLo>3.2</LimitLo>\n      <LimitHi>3.4</LimitHi>\n      <StringMatch></StringMatch>\n      <BooleanMatch></BooleanMatch>\n      <DisplayFormat>%.2f</DisplayFormat>\n      <Units>_V</Units>\n      <TestTime></TestTime>\n    </Test>\n    <Test>\n      <Code>10.83</Code>\n      <Name>SELECTOR_41_L</Name>\n      <Description></Description>\n      <Group>Pin_Tests</Group>\n      <IsGroup>No</IsGroup>\n      <Tag>Pin_Tests:SELECTOR_41_L</Tag>\n      <Method>Test_Pin_N_Low</Method>\n      <Parameter>CH41</Parameter>\n      <DataType>Dbl</DataType>\n      <Value></Value>\n      <Status></Status>\n      <LimitLo>0</LimitLo>\n      <LimitHi>0.01</LimitHi>\n      <StringMatch></StringMatch>\n      <BooleanMatch></BooleanMatch>\n      <DisplayFormat>%.2f</DisplayFormat>\n      <Units>_V</Units>\n      <TestTime></TestTime>\n    </Test>\n    <Test>\n      <Code>10.84</Code>\n      <Name>SELECTOR_42_H</Name>\n      <Description></Description>\n      <Group>Pin_Tests</Group>\n      <IsGroup>No</IsGroup>\n      <Tag>Pin_Tests:SELECTOR_42_H</Tag>\n      <Method>Test_Pin_N_High</Method>\n      <Parameter>CH42</Parameter>\n      <DataType>Dbl</DataType>\n      <Value></Value>\n      <Status></Status>\n      <LimitLo>3.2</LimitLo>\n      <LimitHi>3.4</LimitHi>\n      <StringMatch></StringMatch>\n      <BooleanMatch></BooleanMatch>\n      <DisplayFormat>%.2f</DisplayFormat>\n      <Units>_V</Units>\n      <TestTime></TestTime>\n    </Test>\n    <Test>\n      <Code>10.85</Code>\n      <Name>SELECTOR_42_L</Name>\n      <Description></Description>\n      <Group>Pin_Tests</Group>\n      <IsGroup>No</IsGroup>\n      <Tag>Pin_Tests:SELECTOR_42_L</Tag>\n      <Method>Test_Pin_N_Low</Method>\n      <Parameter>CH42</Parameter>\n      <DataType>Dbl</DataType>\n      <Value></Value>\n      <Status></Status>\n      <LimitLo>0</LimitLo>\n      <LimitHi>0.01</LimitHi>\n      <StringMatch></StringMatch>\n      <BooleanMatch></BooleanMatch>\n      <DisplayFormat>%.2f</DisplayFormat>\n      <Units>_V</Units>\n      <TestTime></TestTime>\n    </Test>\n    <Test>\n      <Code>10.86</Code>\n      <Name>SELECTOR_43_H</Name>\n      <Description></Description>\n      <Group>Pin_Tests</Group>\n      <IsGroup>No</IsGroup>\n      <Tag>Pin_Tests:SELECTOR_43_H</Tag>\n      <Method>Test_Pin_N_High</Method>\n      <Parameter>CH43</Parameter>\n      <DataType>Dbl</DataType>\n      <Value></Value>\n      <Status></Status>\n      <LimitLo>3.2</LimitLo>\n      <LimitHi>3.4</LimitHi>\n      <StringMatch></StringMatch>\n      <BooleanMatch></BooleanMatch>\n      <DisplayFormat>%.2f</DisplayFormat>\n      <Units>_V</Units>\n      <TestTime></TestTime>\n    </Test>\n    <Test>\n      <Code>10.87</Code>\n      <Name>SELECTOR_43_L</Name>\n      <Description></Description>\n      <Group>Pin_Tests</Group>\n      <IsGroup>No</IsGroup>\n      <Tag>Pin_Tests:SELECTOR_43_L</Tag>\n      <Method>Test_Pin_N_Low</Method>\n      <Parameter>CH43</Parameter>\n      <DataType>Dbl</DataType>\n      <Value></Value>\n      <Status></Status>\n      <LimitLo>0</LimitLo>\n      <LimitHi>0.01</LimitHi>\n      <StringMatch></StringMatch>\n      <BooleanMatch></BooleanMatch>\n      <DisplayFormat>%.2f</DisplayFormat>\n      <Units>_V</Units>\n      <TestTime></TestTime>\n    </Test>\n    <Test>\n      <Code>10.88</Code>\n      <Name>SELECTOR_44_H</Name>\n      <Description></Description>\n      <Group>Pin_Tests</Group>\n      <IsGroup>No</IsGroup>\n      <Tag>Pin_Tests:SELECTOR_44_H</Tag>\n      <Method>Test_Pin_N_High</Method>\n      <Parameter>CH44</Parameter>\n      <DataType>Dbl</DataType>\n      <Value></Value>\n      <Status></Status>\n      <LimitLo>3.2</LimitLo>\n      <LimitHi>3.4</LimitHi>\n      <StringMatch></StringMatch>\n      <BooleanMatch></BooleanMatch>\n      <DisplayFormat>%.2f</DisplayFormat>\n      <Units>_V</Units>\n      <TestTime></TestTime>\n    </Test>\n    <Test>\n      <Code>10.89</Code>\n      <Name>SELECTOR_44_L</Name>\n      <Description></Description>\n      <Group>Pin_Tests</Group>\n      <IsGroup>No</IsGroup>\n      <Tag>Pin_Tests:SELECTOR_44_L</Tag>\n      <Method>Test_Pin_N_Low</Method>\n      <Parameter>CH44</Parameter>\n      <DataType>Dbl</DataType>\n      <Value></Value>\n      <Status></Status>\n      <LimitLo>0</LimitLo>\n      <LimitHi>0.01</LimitHi>\n      <StringMatch></StringMatch>\n      <BooleanMatch></BooleanMatch>\n      <DisplayFormat>%.2f</DisplayFormat>\n      <Units>_V</Units>\n      <TestTime></TestTime>\n    </Test>\n    <Test>\n      <Code>10.90</Code>\n      <Name>SELECTOR_45_H</Name>\n      <Description></Description>\n      <Group>Pin_Tests</Group>\n      <IsGroup>No</IsGroup>\n      <Tag>Pin_Tests:SELECTOR_45_H</Tag>\n      <Method>Test_Pin_N_High</Method>\n      <Parameter>CH45</Parameter>\n      <DataType>Dbl</DataType>\n      <Value></Value>\n      <Status></Status>\n      <LimitLo>3.2</LimitLo>\n      <LimitHi>3.4</LimitHi>\n      <StringMatch></StringMatch>\n      <BooleanMatch></BooleanMatch>\n      <DisplayFormat>%.2f</DisplayFormat>\n      <Units>_V</Units>\n      <TestTime></TestTime>\n    </Test>\n    <Test>\n      <Code>10.91</Code>\n      <Name>SELECTOR_45_L</Name>\n      <Description></Description>\n      <Group>Pin_Tests</Group>\n      <IsGroup>No</IsGroup>\n      <Tag>Pin_Tests:SELECTOR_45_L</Tag>\n      <Method>Test_Pin_N_Low</Method>\n      <Parameter>CH45</Parameter>\n      <DataType>Dbl</DataType>\n      <Value></Value>\n      <Status></Status>\n      <LimitLo>0</LimitLo>\n      <LimitHi>0.01</LimitHi>\n      <StringMatch></StringMatch>\n      <BooleanMatch></BooleanMatch>\n      <DisplayFormat>%.2f</DisplayFormat>\n      <Units>_V</Units>\n      <TestTime></TestTime>\n    </Test>\n    <Test>\n      <Code>10.92</Code>\n      <Name>SELECTOR_46_H</Name>\n      <Description></Description>\n      <Group>Pin_Tests</Group>\n      <IsGroup>No</IsGroup>\n      <Tag>Pin_Tests:SELECTOR_46_H</Tag>\n      <Method>Test_Pin_N_High</Method>\n      <Parameter>CH46</Parameter>\n      <DataType>Dbl</DataType>\n      <Value></Value>\n      <Status></Status>\n      <LimitLo>3.2</LimitLo>\n      <LimitHi>3.4</LimitHi>\n      <StringMatch></StringMatch>\n      <BooleanMatch></BooleanMatch>\n      <DisplayFormat>%.2f</DisplayFormat>\n      <Units>_V</Units>\n      <TestTime></TestTime>\n    </Test>\n    <Test>\n      <Code>10.93</Code>\n      <Name>SELECTOR_46_L</Name>\n      <Description></Description>\n      <Group>Pin_Tests</Group>\n      <IsGroup>No</IsGroup>\n      <Tag>Pin_Tests:SELECTOR_46_L</Tag>\n      <Method>Test_Pin_N_Low</Method>\n      <Parameter>CH46</Parameter>\n      <DataType>Dbl</DataType>\n      <Value></Value>\n      <Status></Status>\n      <LimitLo>0</LimitLo>\n      <LimitHi>0.01</LimitHi>\n      <StringMatch></StringMatch>\n      <BooleanMatch></BooleanMatch>\n      <DisplayFormat>%.2f</DisplayFormat>\n      <Units>_V</Units>\n      <TestTime></TestTime>\n    </Test>\n    <Test>\n      <Code>10.94</Code>\n      <Name>SELECTOR_47_H</Name>\n      <Description></Description>\n      <Group>Pin_Tests</Group>\n      <IsGroup>No</IsGroup>\n      <Tag>Pin_Tests:SELECTOR_47_H</Tag>\n      <Method>Test_Pin_N_High</Method>\n      <Parameter>CH47</Parameter>\n      <DataType>Dbl</DataType>\n      <Value></Value>\n      <Status></Status>\n      <LimitLo>3.2</LimitLo>\n      <LimitHi>3.4</LimitHi>\n      <StringMatch></StringMatch>\n      <BooleanMatch></BooleanMatch>\n      <DisplayFormat>%.2f</DisplayFormat>\n      <Units>_V</Units>\n      <TestTime></TestTime>\n    </Test>\n    <Test>\n      <Code>10.95</Code>\n      <Name>SELECTOR_47_L</Name>\n      <Description></Description>\n      <Group>Pin_Tests</Group>\n      <IsGroup>No</IsGroup>\n      <Tag>Pin_Tests:SELECTOR_47_L</Tag>\n      <Method>Test_Pin_N_Low</Method>\n      <Parameter>CH47</Parameter>\n      <DataType>Dbl</DataType>\n      <Value></Value>\n      <Status></Status>\n      <LimitLo>0</LimitLo>\n      <LimitHi>0.01</LimitHi>\n      <StringMatch></StringMatch>\n      <BooleanMatch></BooleanMatch>\n      <DisplayFormat>%.2f</DisplayFormat>\n      <Units>_V</Units>\n      <TestTime></TestTime>\n    </Test>\n    <Test>\n      <Code>10.96</Code>\n      <Name>SELECTOR_48_H</Name>\n      <Description></Description>\n      <Group>Pin_Tests</Group>\n      <IsGroup>No</IsGroup>\n      <Tag>Pin_Tests:SELECTOR_48_H</Tag>\n      <Method>Test_Pin_N_High</Method>\n      <Parameter>CH48</Parameter>\n      <DataType>Dbl</DataType>\n      <Value></Value>\n      <Status></Status>\n      <LimitLo>3.2</LimitLo>\n      <LimitHi>3.4</LimitHi>\n      <StringMatch></StringMatch>\n      <BooleanMatch></BooleanMatch>\n      <DisplayFormat>%.2f</DisplayFormat>\n      <Units>_V</Units>\n      <TestTime></TestTime>\n    </Test>\n    <Test>\n      <Code>10.97</Code>\n      <Name>SELECTOR_48_L</Name>\n      <Description></Description>\n      <Group>Pin_Tests</Group>\n      <IsGroup>No</IsGroup>\n      <Tag>Pin_Tests:SELECTOR_48_L</Tag>\n      <Method>Test_Pin_N_Low</Method>\n      <Parameter>CH48</Parameter>\n      <DataType>Dbl</DataType>\n      <Value></Value>\n      <Status></Status>\n      <LimitLo>0</LimitLo>\n      <LimitHi>0.01</LimitHi>\n      <StringMatch></StringMatch>\n      <BooleanMatch></BooleanMatch>\n      <DisplayFormat>%.2f</DisplayFormat>\n      <Units>_V</Units>\n      <TestTime></TestTime>\n    </Test>\n    <Test>\n      <Code>10.98</Code>\n      <Name>SELECTOR_49_H</Name>\n      <Description></Description>\n      <Group>Pin_Tests</Group>\n      <IsGroup>No</IsGroup>\n      <Tag>Pin_Tests:SELECTOR_49_H</Tag>\n      <Method>Test_Pin_N_High</Method>\n      <Parameter>CH49</Parameter>\n      <DataType>Dbl</DataType>\n      <Value></Value>\n      <Status></Status>\n      <LimitLo>3.2</LimitLo>\n      <LimitHi>3.4</LimitHi>\n      <StringMatch></StringMatch>\n      <BooleanMatch></BooleanMatch>\n      <DisplayFormat>%.2f</DisplayFormat>\n      <Units>_V</Units>\n      <TestTime></TestTime>\n    </Test>\n    <Test>\n      <Code>10.99</Code>\n      <Name>SELECTOR_49_L</Name>\n      <Description></Description>\n      <Group>Pin_Tests</Group>\n      <IsGroup>No</IsGroup>\n      <Tag>Pin_Tests:SELECTOR_49_L</Tag>\n      <Method>Test_Pin_N_Low</Method>\n      <Parameter>CH49</Parameter>\n      <DataType>Dbl</DataType>\n      <Value></Value>\n      <Status></Status>\n      <LimitLo>0</LimitLo>\n      <LimitHi>0.01</LimitHi>\n      <StringMatch></StringMatch>\n      <BooleanMatch></BooleanMatch>\n      <DisplayFormat>%.2f</DisplayFormat>\n      <Units>_V</Units>\n      <TestTime></TestTime>\n    </Test>\n    <Test>\n      <Code>10.100</Code>\n      <Name>SELECTOR_50_H</Name>\n      <Description></Description>\n      <Group>Pin_Tests</Group>\n      <IsGroup>No</IsGroup>\n      <Tag>Pin_Tests:SELECTOR_50_H</Tag>\n      <Method>Test_Pin_N_High</Method>\n      <Parameter>CH50</Parameter>\n      <DataType>Dbl</DataType>\n      <Value></Value>\n      <Status></Status>\n      <LimitLo>3.2</LimitLo>\n      <LimitHi>3.4</LimitHi>\n      <StringMatch></StringMatch>\n      <BooleanMatch></BooleanMatch>\n      <DisplayFormat>%.2f</DisplayFormat>\n      <Units>_V</Units>\n      <TestTime></TestTime>\n    </Test>\n    <Test>\n      <Code>10.101</Code>\n      <Name>SELECTOR_50_L</Name>\n      <Description></Description>\n      <Group>Pin_Tests</Group>\n      <IsGroup>No</IsGroup>\n      <Tag>Pin_Tests:SELECTOR_50_L</Tag>\n      <Method>Test_Pin_N_Low</Method>\n      <Parameter>CH50</Parameter>\n      <DataType>Dbl</DataType>\n      <Value></Value>\n      <Status></Status>\n      <LimitLo>0</LimitLo>\n      <LimitHi>0.01</LimitHi>\n      <StringMatch></StringMatch>\n      <BooleanMatch></BooleanMatch>\n      <DisplayFormat>%.2f</DisplayFormat>\n      <Units>_V</Units>\n      <TestTime></TestTime>\n    </Test>\n    <Test>\n      <Code>10.102</Code>\n      <Name>SELECTOR_51_H</Name>\n      <Description></Description>\n      <Group>Pin_Tests</Group>\n      <IsGroup>No</IsGroup>\n      <Tag>Pin_Tests:SELECTOR_51_H</Tag>\n      <Method>Test_Pin_N_High</Method>\n      <Parameter>CH51</Parameter>\n      <DataType>Dbl</DataType>\n      <Value></Value>\n      <Status></Status>\n      <LimitLo>3.2</LimitLo>\n      <LimitHi>3.4</LimitHi>\n      <StringMatch></StringMatch>\n      <BooleanMatch></BooleanMatch>\n      <DisplayFormat>%.2f</DisplayFormat>\n      <Units>_V</Units>\n      <TestTime></TestTime>\n    </Test>\n    <Test>\n      <Code>10.103</Code>\n      <Name>SELECTOR_51_L</Name>\n      <Description></Description>\n      <Group>Pin_Tests</Group>\n      <IsGroup>No</IsGroup>\n      <Tag>Pin_Tests:SELECTOR_51_L</Tag>\n      <Method>Test_Pin_N_Low</Method>\n      <Parameter>CH51</Parameter>\n      <DataType>Dbl</DataType>\n      <Value></Value>\n      <Status></Status>\n      <LimitLo>0</LimitLo>\n      <LimitHi>0.01</LimitHi>\n      <StringMatch></StringMatch>\n      <BooleanMatch></BooleanMatch>\n      <DisplayFormat>%.2f</DisplayFormat>\n      <Units>_V</Units>\n      <TestTime></TestTime>\n    </Test>\n    <Test>\n      <Code>10.104</Code>\n      <Name>SELECTOR_52_H</Name>\n      <Description></Description>\n      <Group>Pin_Tests</Group>\n      <IsGroup>No</IsGroup>\n      <Tag>Pin_Tests:SELECTOR_52_H</Tag>\n      <Method>Test_Pin_N_High</Method>\n      <Parameter>CH52</Parameter>\n      <DataType>Dbl</DataType>\n      <Value></Value>\n      <Status></Status>\n      <LimitLo>3.2</LimitLo>\n      <LimitHi>3.4</LimitHi>\n      <StringMatch></StringMatch>\n      <BooleanMatch></BooleanMatch>\n      <DisplayFormat>%.2f</DisplayFormat>\n      <Units>_V</Units>\n      <TestTime></TestTime>\n    </Test>\n    <Test>\n      <Code>10.105</Code>\n      <Name>SELECTOR_52_L</Name>\n      <Description></Description>\n      <Group>Pin_Tests</Group>\n      <IsGroup>No</IsGroup>\n      <Tag>Pin_Tests:SELECTOR_52_L</Tag>\n      <Method>Test_Pin_N_Low</Method>\n      <Parameter>CH52</Parameter>\n      <DataType>Dbl</DataType>\n      <Value></Value>\n      <Status></Status>\n      <LimitLo>0</LimitLo>\n      <LimitHi>0.01</LimitHi>\n      <StringMatch></StringMatch>\n      <BooleanMatch></BooleanMatch>\n      <DisplayFormat>%.2f</DisplayFormat>\n      <Units>_V</Units>\n      <TestTime></TestTime>\n    </Test>\n    <Test>\n      <Code>10.106</Code>\n      <Name>SELECTOR_53_H</Name>\n      <Description></Description>\n      <Group>Pin_Tests</Group>\n      <IsGroup>No</IsGroup>\n      <Tag>Pin_Tests:SELECTOR_53_H</Tag>\n      <Method>Test_Pin_N_High</Method>\n      <Parameter>CH53</Parameter>\n      <DataType>Dbl</DataType>\n      <Value></Value>\n      <Status></Status>\n      <LimitLo>3.2</LimitLo>\n      <LimitHi>3.4</LimitHi>\n      <StringMatch></StringMatch>\n      <BooleanMatch></BooleanMatch>\n      <DisplayFormat>%.2f</DisplayFormat>\n      <Units>_V</Units>\n      <TestTime></TestTime>\n    </Test>\n    <Test>\n      <Code>10.107</Code>\n      <Name>SELECTOR_53_L</Name>\n      <Description></Description>\n      <Group>Pin_Tests</Group>\n      <IsGroup>No</IsGroup>\n      <Tag>Pin_Tests:SELECTOR_53_L</Tag>\n      <Method>Test_Pin_N_Low</Method>\n      <Parameter>CH53</Parameter>\n      <DataType>Dbl</DataType>\n      <Value></Value>\n      <Status></Status>\n      <LimitLo>0</LimitLo>\n      <LimitHi>0.01</LimitHi>\n      <StringMatch></StringMatch>\n      <BooleanMatch></BooleanMatch>\n      <DisplayFormat>%.2f</DisplayFormat>\n      <Units>_V</Units>\n      <TestTime></TestTime>\n    </Test>\n    <Test>\n      <Code>10.108</Code>\n      <Name>SELECTOR_54_H</Name>\n      <Description></Description>\n      <Group>Pin_Tests</Group>\n      <IsGroup>No</IsGroup>\n      <Tag>Pin_Tests:SELECTOR_54_H</Tag>\n      <Method>Test_Pin_N_High</Method>\n      <Parameter>CH54</Parameter>\n      <DataType>Dbl</DataType>\n      <Value></Value>\n      <Status></Status>\n      <LimitLo>3.2</LimitLo>\n      <LimitHi>3.4</LimitHi>\n      <StringMatch></StringMatch>\n      <BooleanMatch></BooleanMatch>\n      <DisplayFormat>%.2f</DisplayFormat>\n      <Units>_V</Units>\n      <TestTime></TestTime>\n    </Test>\n    <Test>\n      <Code>10.109</Code>\n      <Name>SELECTOR_54_L</Name>\n      <Description></Description>\n      <Group>Pin_Tests</Group>\n      <IsGroup>No</IsGroup>\n      <Tag>Pin_Tests:SELECTOR_54_L</Tag>\n      <Method>Test_Pin_N_Low</Method>\n      <Parameter>CH54</Parameter>\n      <DataType>Dbl</DataType>\n      <Value></Value>\n      <Status></Status>\n      <LimitLo>0</LimitLo>\n      <LimitHi>0.01</LimitHi>\n      <StringMatch></StringMatch>\n      <BooleanMatch></BooleanMatch>\n      <DisplayFormat>%.2f</DisplayFormat>\n      <Units>_V</Units>\n      <TestTime></TestTime>\n    </Test>\n    <Test>\n      <Code>10.110</Code>\n      <Name>SELECTOR_55_H</Name>\n      <Description></Description>\n      <Group>Pin_Tests</Group>\n      <IsGroup>No</IsGroup>\n      <Tag>Pin_Tests:SELECTOR_55_H</Tag>\n      <Method>Test_Pin_N_High</Method>\n      <Parameter>CH55</Parameter>\n      <DataType>Dbl</DataType>\n      <Value></Value>\n      <Status></Status>\n      <LimitLo>3.2</LimitLo>\n      <LimitHi>3.4</LimitHi>\n      <StringMatch></StringMatch>\n      <BooleanMatch></BooleanMatch>\n      <DisplayFormat>%.2f</DisplayFormat>\n      <Units>_V</Units>\n      <TestTime></TestTime>\n    </Test>\n    <Test>\n      <Code>10.111</Code>\n      <Name>SELECTOR_55_L</Name>\n      <Description></Description>\n      <Group>Pin_Tests</Group>\n      <IsGroup>No</IsGroup>\n      <Tag>Pin_Tests:SELECTOR_55_L</Tag>\n      <Method>Test_Pin_N_Low</Method>\n      <Parameter>CH55</Parameter>\n      <DataType>Dbl</DataType>\n      <Value></Value>\n      <Status></Status>\n      <LimitLo>0</LimitLo>\n      <LimitHi>0.01</LimitHi>\n      <StringMatch></StringMatch>\n      <BooleanMatch></BooleanMatch>\n      <DisplayFormat>%.2f</DisplayFormat>\n      <Units>_V</Units>\n      <TestTime></TestTime>\n    </Test>\n    <Test>\n      <Code>10.112</Code>\n      <Name>SELECTOR_56_H</Name>\n      <Description></Description>\n      <Group>Pin_Tests</Group>\n      <IsGroup>No</IsGroup>\n      <Tag>Pin_Tests:SELECTOR_56_H</Tag>\n      <Method>Test_Pin_N_High</Method>\n      <Parameter>CH56</Parameter>\n      <DataType>Dbl</DataType>\n      <Value></Value>\n      <Status></Status>\n      <LimitLo>3.2</LimitLo>\n      <LimitHi>3.4</LimitHi>\n      <StringMatch></StringMatch>\n      <BooleanMatch></BooleanMatch>\n      <DisplayFormat>%.2f</DisplayFormat>\n      <Units>_V</Units>\n      <TestTime></TestTime>\n    </Test>\n    <Test>\n      <Code>10.113</Code>\n      <Name>SELECTOR_56_L</Name>\n      <Description></Description>\n      <Group>Pin_Tests</Group>\n      <IsGroup>No</IsGroup>\n      <Tag>Pin_Tests:SELECTOR_56_L</Tag>\n      <Method>Test_Pin_N_Low</Method>\n      <Parameter>CH56</Parameter>\n      <DataType>Dbl</DataType>\n      <Value></Value>\n      <Status></Status>\n      <LimitLo>0</LimitLo>\n      <LimitHi>0.01</LimitHi>\n      <StringMatch></StringMatch>\n      <BooleanMatch></BooleanMatch>\n      <DisplayFormat>%.2f</DisplayFormat>\n      <Units>_V</Units>\n      <TestTime></TestTime>\n    </Test>\n    <Test>\n      <Code>10.114</Code>\n      <Name>SELECTOR_57_H</Name>\n      <Description></Description>\n      <Group>Pin_Tests</Group>\n      <IsGroup>No</IsGroup>\n      <Tag>Pin_Tests:SELECTOR_57_H</Tag>\n      <Method>Test_Pin_N_High</Method>\n      <Parameter>CH57</Parameter>\n      <DataType>Dbl</DataType>\n      <Value></Value>\n      <Status></Status>\n      <LimitLo>3.2</LimitLo>\n      <LimitHi>3.4</LimitHi>\n      <StringMatch></StringMatch>\n      <BooleanMatch></BooleanMatch>\n      <DisplayFormat>%.2f</DisplayFormat>\n      <Units>_V</Units>\n      <TestTime></TestTime>\n    </Test>\n    <Test>\n      <Code>10.115</Code>\n      <Name>SELECTOR_57_L</Name>\n      <Description></Description>\n      <Group>Pin_Tests</Group>\n      <IsGroup>No</IsGroup>\n      <Tag>Pin_Tests:SELECTOR_57_L</Tag>\n      <Method>Test_Pin_N_Low</Method>\n      <Parameter>CH57</Parameter>\n      <DataType>Dbl</DataType>\n      <Value></Value>\n      <Status></Status>\n      <LimitLo>0</LimitLo>\n      <LimitHi>0.01</LimitHi>\n      <StringMatch></StringMatch>\n      <BooleanMatch></BooleanMatch>\n      <DisplayFormat>%.2f</DisplayFormat>\n      <Units>_V</Units>\n      <TestTime></TestTime>\n    </Test>\n    <Test>\n      <Code>10.116</Code>\n      <Name>SELECTOR_58_H</Name>\n      <Description></Description>\n      <Group>Pin_Tests</Group>\n      <IsGroup>No</IsGroup>\n      <Tag>Pin_Tests:SELECTOR_58_H</Tag>\n      <Method>Test_Pin_N_High</Method>\n      <Parameter>CH58</Parameter>\n      <DataType>Dbl</DataType>\n      <Value></Value>\n      <Status></Status>\n      <LimitLo>3.2</LimitLo>\n      <LimitHi>3.4</LimitHi>\n      <StringMatch></StringMatch>\n      <BooleanMatch></BooleanMatch>\n      <DisplayFormat>%.2f</DisplayFormat>\n      <Units>_V</Units>\n      <TestTime></TestTime>\n    </Test>\n    <Test>\n      <Code>10.117</Code>\n      <Name>SELECTOR_58_L</Name>\n      <Description></Description>\n      <Group>Pin_Tests</Group>\n      <IsGroup>No</IsGroup>\n      <Tag>Pin_Tests:SELECTOR_58_L</Tag>\n      <Method>Test_Pin_N_Low</Method>\n      <Parameter>CH58</Parameter>\n      <DataType>Dbl</DataType>\n      <Value></Value>\n      <Status></Status>\n      <LimitLo>0</LimitLo>\n      <LimitHi>0.01</LimitHi>\n      <StringMatch></StringMatch>\n      <BooleanMatch></BooleanMatch>\n      <DisplayFormat>%.2f</DisplayFormat>\n      <Units>_V</Units>\n      <TestTime></TestTime>\n    </Test>\n    <Test>\n      <Code>10.118</Code>\n      <Name>SELECTOR_59_H</Name>\n      <Description></Description>\n      <Group>Pin_Tests</Group>\n      <IsGroup>No</IsGroup>\n      <Tag>Pin_Tests:SELECTOR_59_H</Tag>\n      <Method>Test_Pin_N_High</Method>\n      <Parameter>CH59</Parameter>\n      <DataType>Dbl</DataType>\n      <Value></Value>\n      <Status></Status>\n      <LimitLo>3.2</LimitLo>\n      <LimitHi>3.4</LimitHi>\n      <StringMatch></StringMatch>\n      <BooleanMatch></BooleanMatch>\n      <DisplayFormat>%.2f</DisplayFormat>\n      <Units>_V</Units>\n      <TestTime></TestTime>\n    </Test>\n    <Test>\n      <Code>10.119</Code>\n      <Name>SELECTOR_59_L</Name>\n      <Description></Description>\n      <Group>Pin_Tests</Group>\n      <IsGroup>No</IsGroup>\n      <Tag>Pin_Tests:SELECTOR_59_L</Tag>\n      <Method>Test_Pin_N_Low</Method>\n      <Parameter>CH59</Parameter>\n      <DataType>Dbl</DataType>\n      <Value></Value>\n      <Status></Status>\n      <LimitLo>0</LimitLo>\n      <LimitHi>0.01</LimitHi>\n      <StringMatch></StringMatch>\n      <BooleanMatch></BooleanMatch>\n      <DisplayFormat>%.2f</DisplayFormat>\n      <Units>_V</Units>\n      <TestTime></TestTime>\n    </Test>\n    <Test>\n      <Code>10.120</Code>\n      <Name>SELECTOR_60_H</Name>\n      <Description></Description>\n      <Group>Pin_Tests</Group>\n      <IsGroup>No</IsGroup>\n      <Tag>Pin_Tests:SELECTOR_60_H</Tag>\n      <Method>Test_Pin_N_High</Method>\n      <Parameter>CH60</Parameter>\n      <DataType>Dbl</DataType>\n      <Value></Value>\n      <Status></Status>\n      <LimitLo>3.2</LimitLo>\n      <LimitHi>3.4</LimitHi>\n      <StringMatch></StringMatch>\n      <BooleanMatch></BooleanMatch>\n      <DisplayFormat>%.2f</DisplayFormat>\n      <Units>_V</Units>\n      <TestTime></TestTime>\n    </Test>\n    <Test>\n      <Code>10.121</Code>\n      <Name>SELECTOR_60_L</Name>\n      <Description></Description>\n      <Group>Pin_Tests</Group>\n      <IsGroup>No</IsGroup>\n      <Tag>Pin_Tests:SELECTOR_60_L</Tag>\n      <Method>Test_Pin_N_Low</Method>\n      <Parameter>CH60</Parameter>\n      <DataType>Dbl</DataType>\n      <Value></Value>\n      <Status></Status>\n      <LimitLo>0</LimitLo>\n      <LimitHi>0.01</LimitHi>\n      <StringMatch></StringMatch>\n      <BooleanMatch></BooleanMatch>\n      <DisplayFormat>%.2f</DisplayFormat>\n      <Units>_V</Units>\n      <TestTime></TestTime>\n    </Test>\n    <Test>\n      <Code>10.122</Code>\n      <Name>SELECTOR_61_H</Name>\n      <Description></Description>\n      <Group>Pin_Tests</Group>\n      <IsGroup>No</IsGroup>\n      <Tag>Pin_Tests:SELECTOR_61_H</Tag>\n      <Method>Test_Pin_N_High</Method>\n      <Parameter>CH61</Parameter>\n      <DataType>Dbl</DataType>\n      <Value></Value>\n      <Status></Status>\n      <LimitLo>3.2</LimitLo>\n      <LimitHi>3.4</LimitHi>\n      <StringMatch></StringMatch>\n      <BooleanMatch></BooleanMatch>\n      <DisplayFormat>%.2f</DisplayFormat>\n      <Units>_V</Units>\n      <TestTime></TestTime>\n    </Test>\n    <Test>\n      <Code>10.123</Code>\n      <Name>SELECTOR_61_L</Name>\n      <Description></Description>\n      <Group>Pin_Tests</Group>\n      <IsGroup>No</IsGroup>\n      <Tag>Pin_Tests:SELECTOR_61_L</Tag>\n      <Method>Test_Pin_N_Low</Method>\n      <Parameter>CH61</Parameter>\n      <DataType>Dbl</DataType>\n      <Value></Value>\n      <Status></Status>\n      <LimitLo>0</LimitLo>\n      <LimitHi>0.01</LimitHi>\n      <StringMatch></StringMatch>\n      <BooleanMatch></BooleanMatch>\n      <DisplayFormat>%.2f</DisplayFormat>\n      <Units>_V</Units>\n      <TestTime></TestTime>\n    </Test>\n    <Test>\n      <Code>10.124</Code>\n      <Name>SELECTOR_62_H</Name>\n      <Description></Description>\n      <Group>Pin_Tests</Group>\n      <IsGroup>No</IsGroup>\n      <Tag>Pin_Tests:SELECTOR_62_H</Tag>\n      <Method>Test_Pin_N_High</Method>\n      <Parameter>CH62</Parameter>\n      <DataType>Dbl</DataType>\n      <Value></Value>\n      <Status></Status>\n      <LimitLo>3.2</LimitLo>\n      <LimitHi>3.4</LimitHi>\n      <StringMatch></StringMatch>\n      <BooleanMatch></BooleanMatch>\n      <DisplayFormat>%.2f</DisplayFormat>\n      <Units>_V</Units>\n      <TestTime></TestTime>\n    </Test>\n    <Test>\n      <Code>10.125</Code>\n      <Name>SELECTOR_62_L</Name>\n      <Description></Description>\n      <Group>Pin_Tests</Group>\n      <IsGroup>No</IsGroup>\n      <Tag>Pin_Tests:SELECTOR_62_L</Tag>\n      <Method>Test_Pin_N_Low</Method>\n      <Parameter>CH62</Parameter>\n      <DataType>Dbl</DataType>\n      <Value></Value>\n      <Status></Status>\n      <LimitLo>0</LimitLo>\n      <LimitHi>0.01</LimitHi>\n      <StringMatch></StringMatch>\n      <BooleanMatch></BooleanMatch>\n      <DisplayFormat>%.2f</DisplayFormat>\n      <Units>_V</Units>\n      <TestTime></TestTime>\n    </Test>\n    <Test>\n      <Code>10.126</Code>\n      <Name>SELECTOR_63_H</Name>\n      <Description></Description>\n      <Group>Pin_Tests</Group>\n      <IsGroup>No</IsGroup>\n      <Tag>Pin_Tests:SELECTOR_63_H</Tag>\n      <Method>Test_Pin_N_High</Method>\n      <Parameter>CH63</Parameter>\n      <DataType>Dbl</DataType>\n      <Value></Value>\n      <Status></Status>\n      <LimitLo>3.2</LimitLo>\n      <LimitHi>3.4</LimitHi>\n      <StringMatch></StringMatch>\n      <BooleanMatch></BooleanMatch>\n      <DisplayFormat>%.2f</DisplayFormat>\n      <Units>_V</Units>\n      <TestTime></TestTime>\n    </Test>\n    <Test>\n      <Code>10.127</Code>\n      <Name>SELECTOR_63_L</Name>\n      <Description></Description>\n      <Group>Pin_Tests</Group>\n      <IsGroup>No</IsGroup>\n      <Tag>Pin_Tests:SELECTOR_63_L</Tag>\n      <Method>Test_Pin_N_Low</Method>\n      <Parameter>CH63</Parameter>\n      <DataType>Dbl</DataType>\n      <Value></Value>\n      <Status></Status>\n      <LimitLo>0</LimitLo>\n      <LimitHi>0.01</LimitHi>\n      <StringMatch></StringMatch>\n      <BooleanMatch></BooleanMatch>\n      <DisplayFormat>%.2f</DisplayFormat>\n      <Units>_V</Units>\n      <TestTime></TestTime>\n    </Test>\n    <Test>\n      <Code>10.128</Code>\n      <Name>SELECTOR_64_H</Name>\n      <Description></Description>\n      <Group>Pin_Tests</Group>\n      <IsGroup>No</IsGroup>\n      <Tag>Pin_Tests:SELECTOR_64_H</Tag>\n      <Method>Test_Pin_N_High</Method>\n      <Parameter>CH64</Parameter>\n      <DataType>Dbl</DataType>\n      <Value></Value>\n      <Status></Status>\n      <LimitLo>3.2</LimitLo>\n      <LimitHi>3.4</LimitHi>\n      <StringMatch></StringMatch>\n      <BooleanMatch></BooleanMatch>\n      <DisplayFormat>%.2f</DisplayFormat>\n      <Units>_V</Units>\n      <TestTime></TestTime>\n    </Test>\n    <Test>\n      <Code>10.129</Code>\n      <Name>SELECTOR_64_L</Name>\n      <Description></Description>\n      <Group>Pin_Tests</Group>\n      <IsGroup>No</IsGroup>\n      <Tag>Pin_Tests:SELECTOR_64_L</Tag>\n      <Method>Test_Pin_N_Low</Method>\n      <Parameter>CH64</Parameter>\n      <DataType>Dbl</DataType>\n      <Value></Value>\n      <Status></Status>\n      <LimitLo>0</LimitLo>\n      <LimitHi>0.01</LimitHi>\n      <StringMatch></StringMatch>\n      <BooleanMatch></BooleanMatch>\n      <DisplayFormat>%.2f</DisplayFormat>\n      <Units>_V</Units>\n      <TestTime></TestTime>\n    </Test>\n    <Test>\n      <Code>10.130</Code>\n      <Name>SELECTOR_65_H</Name>\n      <Description></Description>\n      <Group>Pin_Tests</Group>\n      <IsGroup>No</IsGroup>\n      <Tag>Pin_Tests:SELECTOR_65_H</Tag>\n      <Method>Test_Pin_N_High</Method>\n      <Parameter>CH65</Parameter>\n      <DataType>Dbl</DataType>\n      <Value></Value>\n      <Status></Status>\n      <LimitLo>3.2</LimitLo>\n      <LimitHi>3.4</LimitHi>\n      <StringMatch></StringMatch>\n      <BooleanMatch></BooleanMatch>\n      <DisplayFormat>%.2f</DisplayFormat>\n      <Units>_V</Units>\n      <TestTime></TestTime>\n    </Test>\n    <Test>\n      <Code>10.131</Code>\n      <Name>SELECTOR_65_L</Name>\n      <Description></Description>\n      <Group>Pin_Tests</Group>\n      <IsGroup>No</IsGroup>\n      <Tag>Pin_Tests:SELECTOR_65_L</Tag>\n      <Method>Test_Pin_N_Low</Method>\n      <Parameter>CH65</Parameter>\n      <DataType>Dbl</DataType>\n      <Value></Value>\n      <Status></Status>\n      <LimitLo>0</LimitLo>\n      <LimitHi>0.01</LimitHi>\n      <StringMatch></StringMatch>\n      <BooleanMatch></BooleanMatch>\n      <DisplayFormat>%.2f</DisplayFormat>\n      <Units>_V</Units>\n      <TestTime></TestTime>\n    </Test>\n    <Test>\n      <Code>10.132</Code>\n      <Name>SELECTOR_66_H</Name>\n      <Description></Description>\n      <Group>Pin_Tests</Group>\n      <IsGroup>No</IsGroup>\n      <Tag>Pin_Tests:SELECTOR_66_H</Tag>\n      <Method>Test_Pin_N_High</Method>\n      <Parameter>CH66</Parameter>\n      <DataType>Dbl</DataType>\n      <Value></Value>\n      <Status></Status>\n      <LimitLo>3.2</LimitLo>\n      <LimitHi>3.4</LimitHi>\n      <StringMatch></StringMatch>\n      <BooleanMatch></BooleanMatch>\n      <DisplayFormat>%.2f</DisplayFormat>\n      <Units>_V</Units>\n      <TestTime></TestTime>\n    </Test>\n    <Test>\n      <Code>10.133</Code>\n      <Name>SELECTOR_66_L</Name>\n      <Description></Description>\n      <Group>Pin_Tests</Group>\n      <IsGroup>No</IsGroup>\n      <Tag>Pin_Tests:SELECTOR_66_L</Tag>\n      <Method>Test_Pin_N_Low</Method>\n      <Parameter>CH66</Parameter>\n      <DataType>Dbl</DataType>\n      <Value></Value>\n      <Status></Status>\n      <LimitLo>0</LimitLo>\n      <LimitHi>0.01</LimitHi>\n      <StringMatch></StringMatch>\n      <BooleanMatch></BooleanMatch>\n      <DisplayFormat>%.2f</DisplayFormat>\n      <Units>_V</Units>\n      <TestTime></TestTime>\n    </Test>\n    <Test>\n      <Code>10.134</Code>\n      <Name>SELECTOR_67_H</Name>\n      <Description></Description>\n      <Group>Pin_Tests</Group>\n      <IsGroup>No</IsGroup>\n      <Tag>Pin_Tests:SELECTOR_67_H</Tag>\n      <Method>Test_Pin_N_High</Method>\n      <Parameter>CH67</Parameter>\n      <DataType>Dbl</DataType>\n      <Value></Value>\n      <Status></Status>\n      <LimitLo>3.2</LimitLo>\n      <LimitHi>3.4</LimitHi>\n      <StringMatch></StringMatch>\n      <BooleanMatch></BooleanMatch>\n      <DisplayFormat>%.2f</DisplayFormat>\n      <Units>_V</Units>\n      <TestTime></TestTime>\n    </Test>\n    <Test>\n      <Code>10.135</Code>\n      <Name>SELECTOR_67_L</Name>\n      <Description></Description>\n      <Group>Pin_Tests</Group>\n      <IsGroup>No</IsGroup>\n      <Tag>Pin_Tests:SELECTOR_67_L</Tag>\n      <Method>Test_Pin_N_Low</Method>\n      <Parameter>CH67</Parameter>\n      <DataType>Dbl</DataType>\n      <Value></Value>\n      <Status></Status>\n      <LimitLo>0</LimitLo>\n      <LimitHi>0.01</LimitHi>\n      <StringMatch></StringMatch>\n      <BooleanMatch></BooleanMatch>\n      <DisplayFormat>%.2f</DisplayFormat>\n      <Units>_V</Units>\n      <TestTime></TestTime>\n    </Test>\n    <Test>\n      <Code>10.136</Code>\n      <Name>SELECTOR_68_H</Name>\n      <Description></Description>\n      <Group>Pin_Tests</Group>\n      <IsGroup>No</IsGroup>\n      <Tag>Pin_Tests:SELECTOR_68_H</Tag>\n      <Method>Test_Pin_N_High</Method>\n      <Parameter>CH68</Parameter>\n      <DataType>Dbl</DataType>\n      <Value></Value>\n      <Status></Status>\n      <LimitLo>3.2</LimitLo>\n      <LimitHi>3.4</LimitHi>\n      <StringMatch></StringMatch>\n      <BooleanMatch></BooleanMatch>\n      <DisplayFormat>%.2f</DisplayFormat>\n      <Units>_V</Units>\n      <TestTime></TestTime>\n    </Test>\n    <Test>\n      <Code>10.137</Code>\n      <Name>SELECTOR_68_L</Name>\n      <Description></Description>\n      <Group>Pin_Tests</Group>\n      <IsGroup>No</IsGroup>\n      <Tag>Pin_Tests:SELECTOR_68_L</Tag>\n      <Method>Test_Pin_N_Low</Method>\n      <Parameter>CH68</Parameter>\n      <DataType>Dbl</DataType>\n      <Value></Value>\n      <Status></Status>\n      <LimitLo>0</LimitLo>\n      <LimitHi>0.01</LimitHi>\n      <StringMatch></StringMatch>\n      <BooleanMatch></BooleanMatch>\n      <DisplayFormat>%.2f</DisplayFormat>\n      <Units>_V</Units>\n      <TestTime></TestTime>\n    </Test>\n    <Test>\n      <Code>10.138</Code>\n      <Name>SELECTOR_69_H</Name>\n      <Description></Description>\n      <Group>Pin_Tests</Group>\n      <IsGroup>No</IsGroup>\n      <Tag>Pin_Tests:SELECTOR_69_H</Tag>\n      <Method>Test_Pin_N_High</Method>\n      <Parameter>CH69</Parameter>\n      <DataType>Dbl</DataType>\n      <Value></Value>\n      <Status></Status>\n      <LimitLo>3.2</LimitLo>\n      <LimitHi>3.4</LimitHi>\n      <StringMatch></StringMatch>\n      <BooleanMatch></BooleanMatch>\n      <DisplayFormat>%.2f</DisplayFormat>\n      <Units>_V</Units>\n      <TestTime></TestTime>\n    </Test>\n    <Test>\n      <Code>10.139</Code>\n      <Name>SELECTOR_69_L</Name>\n      <Description></Description>\n      <Group>Pin_Tests</Group>\n      <IsGroup>No</IsGroup>\n      <Tag>Pin_Tests:SELECTOR_69_L</Tag>\n      <Method>Test_Pin_N_Low</Method>\n      <Parameter>CH69</Parameter>\n      <DataType>Dbl</DataType>\n      <Value></Value>\n      <Status></Status>\n      <LimitLo>0</LimitLo>\n      <LimitHi>0.01</LimitHi>\n      <StringMatch></StringMatch>\n      <BooleanMatch></BooleanMatch>\n      <DisplayFormat>%.2f</DisplayFormat>\n      <Units>_V</Units>\n      <TestTime></TestTime>\n    </Test>\n    <Test>\n      <Code>10.140</Code>\n      <Name>SELECTOR_70_H</Name>\n      <Description></Description>\n      <Group>Pin_Tests</Group>\n      <IsGroup>No</IsGroup>\n      <Tag>Pin_Tests:SELECTOR_70_H</Tag>\n      <Method>Test_Pin_N_High</Method>\n      <Parameter>CH70</Parameter>\n      <DataType>Dbl</DataType>\n      <Value></Value>\n      <Status></Status>\n      <LimitLo>3.2</LimitLo>\n      <LimitHi>3.4</LimitHi>\n      <StringMatch></StringMatch>\n      <BooleanMatch></BooleanMatch>\n      <DisplayFormat>%.2f</DisplayFormat>\n      <Units>_V</Units>\n      <TestTime></TestTime>\n    </Test>\n    <Test>\n      <Code>10.141</Code>\n      <Name>SELECTOR_70_L</Name>\n      <Description></Description>\n      <Group>Pin_Tests</Group>\n      <IsGroup>No</IsGroup>\n      <Tag>Pin_Tests:SELECTOR_70_L</Tag>\n      <Method>Test_Pin_N_Low</Method>\n      <Parameter>CH70</Parameter>\n      <DataType>Dbl</DataType>\n      <Value></Value>\n      <Status></Status>\n      <LimitLo>0</LimitLo>\n      <LimitHi>0.01</LimitHi>\n      <StringMatch></StringMatch>\n      <BooleanMatch></BooleanMatch>\n      <DisplayFormat>%.2f</DisplayFormat>\n      <Units>_V</Units>\n      <TestTime></TestTime>\n    </Test>\n    <Test>\n      <Code>10.142</Code>\n      <Name>SELECTOR_71_H</Name>\n      <Description></Description>\n      <Group>Pin_Tests</Group>\n      <IsGroup>No</IsGroup>\n      <Tag>Pin_Tests:SELECTOR_71_H</Tag>\n      <Method>Test_Pin_N_High</Method>\n      <Parameter>CH71</Parameter>\n      <DataType>Dbl</DataType>\n      <Value></Value>\n      <Status></Status>\n      <LimitLo>3.2</LimitLo>\n      <LimitHi>3.4</LimitHi>\n      <StringMatch></StringMatch>\n      <BooleanMatch></BooleanMatch>\n      <DisplayFormat>%.2f</DisplayFormat>\n      <Units>_V</Units>\n      <TestTime></TestTime>\n    </Test>\n    <Test>\n      <Code>10.143</Code>\n      <Name>SELECTOR_71_L</Name>\n      <Description></Description>\n      <Group>Pin_Tests</Group>\n      <IsGroup>No</IsGroup>\n      <Tag>Pin_Tests:SELECTOR_71_L</Tag>\n      <Method>Test_Pin_N_Low</Method>\n      <Parameter>CH71</Parameter>\n      <DataType>Dbl</DataType>\n      <Value></Value>\n      <Status></Status>\n      <LimitLo>0</LimitLo>\n      <LimitHi>0.01</LimitHi>\n      <StringMatch></StringMatch>\n      <BooleanMatch></BooleanMatch>\n      <DisplayFormat>%.2f</DisplayFormat>\n      <Units>_V</Units>\n      <TestTime></TestTime>\n    </Test>\n    <Test>\n      <Code>10.144</Code>\n      <Name>SELECTOR_72_H</Name>\n      <Description></Description>\n      <Group>Pin_Tests</Group>\n      <IsGroup>No</IsGroup>\n      <Tag>Pin_Tests:SELECTOR_72_H</Tag>\n      <Method>Test_Pin_N_High</Method>\n      <Parameter>CH72</Parameter>\n      <DataType>Dbl</DataType>\n      <Value></Value>\n      <Status></Status>\n      <LimitLo>3.2</LimitLo>\n      <LimitHi>3.4</LimitHi>\n      <StringMatch></StringMatch>\n      <BooleanMatch></BooleanMatch>\n      <DisplayFormat>%.2f</DisplayFormat>\n      <Units>_V</Units>\n      <TestTime></TestTime>\n    </Test>\n    <Test>\n      <Code>10.145</Code>\n      <Name>SELECTOR_72_L</Name>\n      <Description></Description>\n      <Group>Pin_Tests</Group>\n      <IsGroup>No</IsGroup>\n      <Tag>Pin_Tests:SELECTOR_72_L</Tag>\n      <Method>Test_Pin_N_Low</Method>\n      <Parameter>CH72</Parameter>\n      <DataType>Dbl</DataType>\n      <Value></Value>\n      <Status></Status>\n      <LimitLo>0</LimitLo>\n      <LimitHi>0.01</LimitHi>\n      <StringMatch></StringMatch>\n      <BooleanMatch></BooleanMatch>\n      <DisplayFormat>%.2f</DisplayFormat>\n      <Units>_V</Units>\n      <TestTime></TestTime>\n    </Test>\n    <Test>\n      <Code>10.146</Code>\n      <Name>SELECTOR_73_H</Name>\n      <Description></Description>\n      <Group>Pin_Tests</Group>\n      <IsGroup>No</IsGroup>\n      <Tag>Pin_Tests:SELECTOR_73_H</Tag>\n      <Method>Test_Pin_N_High</Method>\n      <Parameter>CH73</Parameter>\n      <DataType>Dbl</DataType>\n      <Value></Value>\n      <Status></Status>\n      <LimitLo>3.2</LimitLo>\n      <LimitHi>3.4</LimitHi>\n      <StringMatch></StringMatch>\n      <BooleanMatch></BooleanMatch>\n      <DisplayFormat>%.2f</DisplayFormat>\n      <Units>_V</Units>\n      <TestTime></TestTime>\n    </Test>\n    <Test>\n      <Code>10.147</Code>\n      <Name>SELECTOR_73_L</Name>\n      <Description></Description>\n      <Group>Pin_Tests</Group>\n      <IsGroup>No</IsGroup>\n      <Tag>Pin_Tests:SELECTOR_73_L</Tag>\n      <Method>Test_Pin_N_Low</Method>\n      <Parameter>CH73</Parameter>\n      <DataType>Dbl</DataType>\n      <Value></Value>\n      <Status></Status>\n      <LimitLo>0</LimitLo>\n      <LimitHi>0.01</LimitHi>\n      <StringMatch></StringMatch>\n      <BooleanMatch></BooleanMatch>\n      <DisplayFormat>%.2f</DisplayFormat>\n      <Units>_V</Units>\n      <TestTime></TestTime>\n    </Test>\n    <Test>\n      <Code>10.148</Code>\n      <Name>SELECTOR_74_H</Name>\n      <Description></Description>\n      <Group>Pin_Tests</Group>\n      <IsGroup>No</IsGroup>\n      <Tag>Pin_Tests:SELECTOR_74_H</Tag>\n      <Method>Test_Pin_N_High</Method>\n      <Parameter>CH74</Parameter>\n      <DataType>Dbl</DataType>\n      <Value></Value>\n      <Status></Status>\n      <LimitLo>3.2</LimitLo>\n      <LimitHi>3.4</LimitHi>\n      <StringMatch></StringMatch>\n      <BooleanMatch></BooleanMatch>\n      <DisplayFormat>%.2f</DisplayFormat>\n      <Units>_V</Units>\n      <TestTime></TestTime>\n    </Test>\n    <Test>\n      <Code>10.149</Code>\n      <Name>SELECTOR_74_L</Name>\n      <Description></Description>\n      <Group>Pin_Tests</Group>\n      <IsGroup>No</IsGroup>\n      <Tag>Pin_Tests:SELECTOR_74_L</Tag>\n      <Method>Test_Pin_N_Low</Method>\n      <Parameter>CH74</Parameter>\n      <DataType>Dbl</DataType>\n      <Value></Value>\n      <Status></Status>\n      <LimitLo>0</LimitLo>\n      <LimitHi>0.01</LimitHi>\n      <StringMatch></StringMatch>\n      <BooleanMatch></BooleanMatch>\n      <DisplayFormat>%.2f</DisplayFormat>\n      <Units>_V</Units>\n      <TestTime></TestTime>\n    </Test>\n    <Test>\n      <Code>10.150</Code>\n      <Name>SELECTOR_75_H</Name>\n      <Description></Description>\n      <Group>Pin_Tests</Group>\n      <IsGroup>No</IsGroup>\n      <Tag>Pin_Tests:SELECTOR_75_H</Tag>\n      <Method>Test_Pin_N_High</Method>\n      <Parameter>CH75</Parameter>\n      <DataType>Dbl</DataType>\n      <Value></Value>\n      <Status></Status>\n      <LimitLo>3.2</LimitLo>\n      <LimitHi>3.4</LimitHi>\n      <StringMatch></StringMatch>\n      <BooleanMatch></BooleanMatch>\n      <DisplayFormat>%.2f</DisplayFormat>\n      <Units>_V</Units>\n      <TestTime></TestTime>\n    </Test>\n    <Test>\n      <Code>10.151</Code>\n      <Name>SELECTOR_75_L</Name>\n      <Description></Description>\n      <Group>Pin_Tests</Group>\n      <IsGroup>No</IsGroup>\n      <Tag>Pin_Tests:SELECTOR_75_L</Tag>\n      <Method>Test_Pin_N_Low</Method>\n      <Parameter>CH75</Parameter>\n      <DataType>Dbl</DataType>\n      <Value></Value>\n      <Status></Status>\n      <LimitLo>0</LimitLo>\n      <LimitHi>0.01</LimitHi>\n      <StringMatch></StringMatch>\n      <BooleanMatch></BooleanMatch>\n      <DisplayFormat>%.2f</DisplayFormat>\n      <Units>_V</Units>\n      <TestTime></TestTime>\n    </Test>\n    <Test>\n      <Code>10.152</Code>\n      <Name>SELECTOR_76_H</Name>\n      <Description></Description>\n      <Group>Pin_Tests</Group>\n      <IsGroup>No</IsGroup>\n      <Tag>Pin_Tests:SELECTOR_76_H</Tag>\n      <Method>Test_Pin_N_High</Method>\n      <Parameter>CH76</Parameter>\n      <DataType>Dbl</DataType>\n      <Value></Value>\n      <Status></Status>\n      <LimitLo>3.2</LimitLo>\n      <LimitHi>3.4</LimitHi>\n      <StringMatch></StringMatch>\n      <BooleanMatch></BooleanMatch>\n      <DisplayFormat>%.2f</DisplayFormat>\n      <Units>_V</Units>\n      <TestTime></TestTime>\n    </Test>\n    <Test>\n      <Code>10.153</Code>\n      <Name>SELECTOR_76_L</Name>\n      <Description></Description>\n      <Group>Pin_Tests</Group>\n      <IsGroup>No</IsGroup>\n      <Tag>Pin_Tests:SELECTOR_76_L</Tag>\n      <Method>Test_Pin_N_Low</Method>\n      <Parameter>CH76</Parameter>\n      <DataType>Dbl</DataType>\n      <Value></Value>\n      <Status></Status>\n      <LimitLo>0</LimitLo>\n      <LimitHi>0.01</LimitHi>\n      <StringMatch></StringMatch>\n      <BooleanMatch></BooleanMatch>\n      <DisplayFormat>%.2f</DisplayFormat>\n      <Units>_V</Units>\n      <TestTime></TestTime>\n    </Test>\n    <Test>\n      <Code>10.154</Code>\n      <Name>SELECTOR_77_H</Name>\n      <Description></Description>\n      <Group>Pin_Tests</Group>\n      <IsGroup>No</IsGroup>\n      <Tag>Pin_Tests:SELECTOR_77_H</Tag>\n      <Method>Test_Pin_N_High</Method>\n      <Parameter>CH77</Parameter>\n      <DataType>Dbl</DataType>\n      <Value></Value>\n      <Status></Status>\n      <LimitLo>3.2</LimitLo>\n      <LimitHi>3.4</LimitHi>\n      <StringMatch></StringMatch>\n      <BooleanMatch></BooleanMatch>\n      <DisplayFormat>%.2f</DisplayFormat>\n      <Units>_V</Units>\n      <TestTime></TestTime>\n    </Test>\n    <Test>\n      <Code>10.155</Code>\n      <Name>SELECTOR_77_L</Name>\n      <Description></Description>\n      <Group>Pin_Tests</Group>\n      <IsGroup>No</IsGroup>\n      <Tag>Pin_Tests:SELECTOR_77_L</Tag>\n      <Method>Test_Pin_N_Low</Method>\n      <Parameter>CH77</Parameter>\n      <DataType>Dbl</DataType>\n      <Value></Value>\n      <Status></Status>\n      <LimitLo>0</LimitLo>\n      <LimitHi>0.01</LimitHi>\n      <StringMatch></StringMatch>\n      <BooleanMatch></BooleanMatch>\n      <DisplayFormat>%.2f</DisplayFormat>\n      <Units>_V</Units>\n      <TestTime></TestTime>\n    </Test>\n    <Test>\n      <Code>10.156</Code>\n      <Name>SELECTOR_78_H</Name>\n      <Description></Description>\n      <Group>Pin_Tests</Group>\n      <IsGroup>No</IsGroup>\n      <Tag>Pin_Tests:SELECTOR_78_H</Tag>\n      <Method>Test_Pin_N_High</Method>\n      <Parameter>CH78</Parameter>\n      <DataType>Dbl</DataType>\n      <Value></Value>\n      <Status></Status>\n      <LimitLo>3.2</LimitLo>\n      <LimitHi>3.4</LimitHi>\n      <StringMatch></StringMatch>\n      <BooleanMatch></BooleanMatch>\n      <DisplayFormat>%.2f</DisplayFormat>\n      <Units>_V</Units>\n      <TestTime></TestTime>\n    </Test>\n    <Test>\n      <Code>10.157</Code>\n      <Name>SELECTOR_78_L</Name>\n      <Description></Description>\n      <Group>Pin_Tests</Group>\n      <IsGroup>No</IsGroup>\n      <Tag>Pin_Tests:SELECTOR_78_L</Tag>\n      <Method>Test_Pin_N_Low</Method>\n      <Parameter>CH78</Parameter>\n      <DataType>Dbl</DataType>\n      <Value></Value>\n      <Status></Status>\n      <LimitLo>0</LimitLo>\n      <LimitHi>0.01</LimitHi>\n      <StringMatch></StringMatch>\n      <BooleanMatch></BooleanMatch>\n      <DisplayFormat>%.2f</DisplayFormat>\n      <Units>_V</Units>\n      <TestTime></TestTime>\n    </Test>\n    <Test>\n      <Code>10.158</Code>\n      <Name>SELECTOR_79_H</Name>\n      <Description></Description>\n      <Group>Pin_Tests</Group>\n      <IsGroup>No</IsGroup>\n      <Tag>Pin_Tests:SELECTOR_79_H</Tag>\n      <Method>Test_Pin_N_High</Method>\n      <Parameter>CH79</Parameter>\n      <DataType>Dbl</DataType>\n      <Value></Value>\n      <Status></Status>\n      <LimitLo>3.2</LimitLo>\n      <LimitHi>3.4</LimitHi>\n      <StringMatch></StringMatch>\n      <BooleanMatch></BooleanMatch>\n      <DisplayFormat>%.2f</DisplayFormat>\n      <Units>_V</Units>\n      <TestTime></TestTime>\n    </Test>\n    <Test>\n      <Code>10.159</Code>\n      <Name>SELECTOR_79_L</Name>\n      <Description></Description>\n      <Group>Pin_Tests</Group>\n      <IsGroup>No</IsGroup>\n      <Tag>Pin_Tests:SELECTOR_79_L</Tag>\n      <Method>Test_Pin_N_Low</Method>\n      <Parameter>CH79</Parameter>\n      <DataType>Dbl</DataType>\n      <Value></Value>\n      <Status></Status>\n      <LimitLo>0</LimitLo>\n      <LimitHi>0.01</LimitHi>\n      <StringMatch></StringMatch>\n      <BooleanMatch></BooleanMatch>\n      <DisplayFormat>%.2f</DisplayFormat>\n      <Units>_V</Units>\n      <TestTime></TestTime>\n    </Test>\n    <Test>\n      <Code>10.160</Code>\n      <Name>SELECTOR_80_H</Name>\n      <Description></Description>\n      <Group>Pin_Tests</Group>\n      <IsGroup>No</IsGroup>\n      <Tag>Pin_Tests:SELECTOR_80_H</Tag>\n      <Method>Test_Pin_N_High</Method>\n      <Parameter>CH80</Parameter>\n      <DataType>Dbl</DataType>\n      <Value></Value>\n      <Status></Status>\n      <LimitLo>3.2</LimitLo>\n      <LimitHi>3.4</LimitHi>\n      <StringMatch></StringMatch>\n      <BooleanMatch></BooleanMatch>\n      <DisplayFormat>%.2f</DisplayFormat>\n      <Units>_V</Units>\n      <TestTime></TestTime>\n    </Test>\n    <Test>\n      <Code>10.161</Code>\n      <Name>SELECTOR_80_L</Name>\n      <Description></Description>\n      <Group>Pin_Tests</Group>\n      <IsGroup>No</IsGroup>\n      <Tag>Pin_Tests:SELECTOR_80_L</Tag>\n      <Method>Test_Pin_N_Low</Method>\n      <Parameter>CH80</Parameter>\n      <DataType>Dbl</DataType>\n      <Value></Value>\n      <Status></Status>\n      <LimitLo>0</LimitLo>\n      <LimitHi>0.01</LimitHi>\n      <StringMatch></StringMatch>\n      <BooleanMatch></BooleanMatch>\n      <DisplayFormat>%.2f</DisplayFormat>\n      <Units>_V</Units>\n      <TestTime></TestTime>\n    </Test>\n    <Test>\n      <Code>10.162</Code>\n      <Name>SELECTOR_81_H</Name>\n      <Description></Description>\n      <Group>Pin_Tests</Group>\n      <IsGroup>No</IsGroup>\n      <Tag>Pin_Tests:SELECTOR_81_H</Tag>\n      <Method>Test_Pin_N_High</Method>\n      <Parameter>CH81</Parameter>\n      <DataType>Dbl</DataType>\n      <Value></Value>\n      <Status></Status>\n      <LimitLo>3.2</LimitLo>\n      <LimitHi>3.4</LimitHi>\n      <StringMatch></StringMatch>\n      <BooleanMatch></BooleanMatch>\n      <DisplayFormat>%.2f</DisplayFormat>\n      <Units>_V</Units>\n      <TestTime></TestTime>\n    </Test>\n    <Test>\n      <Code>10.163</Code>\n      <Name>SELECTOR_81_L</Name>\n      <Description></Description>\n      <Group>Pin_Tests</Group>\n      <IsGroup>No</IsGroup>\n      <Tag>Pin_Tests:SELECTOR_81_L</Tag>\n      <Method>Test_Pin_N_Low</Method>\n      <Parameter>CH81</Parameter>\n      <DataType>Dbl</DataType>\n      <Value></Value>\n      <Status></Status>\n      <LimitLo>0</LimitLo>\n      <LimitHi>0.01</LimitHi>\n      <StringMatch></StringMatch>\n      <BooleanMatch></BooleanMatch>\n      <DisplayFormat>%.2f</DisplayFormat>\n      <Units>_V</Units>\n      <TestTime></TestTime>\n    </Test>\n    <Test>\n      <Code>10.164</Code>\n      <Name>SELECTOR_82_H</Name>\n      <Description></Description>\n      <Group>Pin_Tests</Group>\n      <IsGroup>No</IsGroup>\n      <Tag>Pin_Tests:SELECTOR_82_H</Tag>\n      <Method>Test_Pin_N_High</Method>\n      <Parameter>CH82</Parameter>\n      <DataType>Dbl</DataType>\n      <Value></Value>\n      <Status></Status>\n      <LimitLo>3.2</LimitLo>\n      <LimitHi>3.4</LimitHi>\n      <StringMatch></StringMatch>\n      <BooleanMatch></BooleanMatch>\n      <DisplayFormat>%.2f</DisplayFormat>\n      <Units>_V</Units>\n      <TestTime></TestTime>\n    </Test>\n    <Test>\n      <Code>10.165</Code>\n      <Name>SELECTOR_82_L</Name>\n      <Description></Description>\n      <Group>Pin_Tests</Group>\n      <IsGroup>No</IsGroup>\n      <Tag>Pin_Tests:SELECTOR_82_L</Tag>\n      <Method>Test_Pin_N_Low</Method>\n      <Parameter>CH82</Parameter>\n      <DataType>Dbl</DataType>\n      <Value></Value>\n      <Status></Status>\n      <LimitLo>0</LimitLo>\n      <LimitHi>0.01</LimitHi>\n      <StringMatch></StringMatch>\n      <BooleanMatch></BooleanMatch>\n      <DisplayFormat>%.2f</DisplayFormat>\n      <Units>_V</Units>\n      <TestTime></TestTime>\n    </Test>\n    <Test>\n      <Code>10.166</Code>\n      <Name>SELECTOR_83_H</Name>\n      <Description></Description>\n      <Group>Pin_Tests</Group>\n      <IsGroup>No</IsGroup>\n      <Tag>Pin_Tests:SELECTOR_83_H</Tag>\n      <Method>Test_Pin_N_High</Method>\n      <Parameter>CH83</Parameter>\n      <DataType>Dbl</DataType>\n      <Value></Value>\n      <Status></Status>\n      <LimitLo>3.2</LimitLo>\n      <LimitHi>3.4</LimitHi>\n      <StringMatch></StringMatch>\n      <BooleanMatch></BooleanMatch>\n      <DisplayFormat>%.2f</DisplayFormat>\n      <Units>_V</Units>\n      <TestTime></TestTime>\n    </Test>\n    <Test>\n      <Code>10.167</Code>\n      <Name>SELECTOR_83_L</Name>\n      <Description></Description>\n      <Group>Pin_Tests</Group>\n      <IsGroup>No</IsGroup>\n      <Tag>Pin_Tests:SELECTOR_83_L</Tag>\n      <Method>Test_Pin_N_Low</Method>\n      <Parameter>CH83</Parameter>\n      <DataType>Dbl</DataType>\n      <Value></Value>\n      <Status></Status>\n      <LimitLo>0</LimitLo>\n      <LimitHi>0.01</LimitHi>\n      <StringMatch></StringMatch>\n      <BooleanMatch></BooleanMatch>\n      <DisplayFormat>%.2f</DisplayFormat>\n      <Units>_V</Units>\n      <TestTime></TestTime>\n    </Test>\n    <Test>\n      <Code>10.168</Code>\n      <Name>SELECTOR_84_H</Name>\n      <Description></Description>\n      <Group>Pin_Tests</Group>\n      <IsGroup>No</IsGroup>\n      <Tag>Pin_Tests:SELECTOR_84_H</Tag>\n      <Method>Test_Pin_N_High</Method>\n      <Parameter>CH84</Parameter>\n      <DataType>Dbl</DataType>\n      <Value></Value>\n      <Status></Status>\n      <LimitLo>3.2</LimitLo>\n      <LimitHi>3.4</LimitHi>\n      <StringMatch></StringMatch>\n      <BooleanMatch></BooleanMatch>\n      <DisplayFormat>%.2f</DisplayFormat>\n      <Units>_V</Units>\n      <TestTime></TestTime>\n    </Test>\n    <Test>\n      <Code>10.169</Code>\n      <Name>SELECTOR_84_L</Name>\n      <Description></Description>\n      <Group>Pin_Tests</Group>\n      <IsGroup>No</IsGroup>\n      <Tag>Pin_Tests:SELECTOR_84_L</Tag>\n      <Method>Test_Pin_N_Low</Method>\n      <Parameter>CH84</Parameter>\n      <DataType>Dbl</DataType>\n      <Value></Value>\n      <Status></Status>\n      <LimitLo>0</LimitLo>\n      <LimitHi>0.01</LimitHi>\n      <StringMatch></StringMatch>\n      <BooleanMatch></BooleanMatch>\n      <DisplayFormat>%.2f</DisplayFormat>\n      <Units>_V</Units>\n      <TestTime></TestTime>\n    </Test>\n    <Test>\n      <Code>10.170</Code>\n      <Name>SELECTOR_85_H</Name>\n      <Description></Description>\n      <Group>Pin_Tests</Group>\n      <IsGroup>No</IsGroup>\n      <Tag>Pin_Tests:SELECTOR_85_H</Tag>\n      <Method>Test_Pin_N_High</Method>\n      <Parameter>CH85</Parameter>\n      <DataType>Dbl</DataType>\n      <Value></Value>\n      <Status></Status>\n      <LimitLo>3.2</LimitLo>\n      <LimitHi>3.4</LimitHi>\n      <StringMatch></StringMatch>\n      <BooleanMatch></BooleanMatch>\n      <DisplayFormat>%.2f</DisplayFormat>\n      <Units>_V</Units>\n      <TestTime></TestTime>\n    </Test>\n    <Test>\n      <Code>10.171</Code>\n      <Name>SELECTOR_85_L</Name>\n      <Description></Description>\n      <Group>Pin_Tests</Group>\n      <IsGroup>No</IsGroup>\n      <Tag>Pin_Tests:SELECTOR_85_L</Tag>\n      <Method>Test_Pin_N_Low</Method>\n      <Parameter>CH85</Parameter>\n      <DataType>Dbl</DataType>\n      <Value></Value>\n      <Status></Status>\n      <LimitLo>0</LimitLo>\n      <LimitHi>0.01</LimitHi>\n      <StringMatch></StringMatch>\n      <BooleanMatch></BooleanMatch>\n      <DisplayFormat>%.2f</DisplayFormat>\n      <Units>_V</Units>\n      <TestTime></TestTime>\n    </Test>\n    <Test>\n      <Code>10.172</Code>\n      <Name>SELECTOR_86_H</Name>\n      <Description></Description>\n      <Group>Pin_Tests</Group>\n      <IsGroup>No</IsGroup>\n      <Tag>Pin_Tests:SELECTOR_86_H</Tag>\n      <Method>Test_Pin_N_High</Method>\n      <Parameter>CH86</Parameter>\n      <DataType>Dbl</DataType>\n      <Value></Value>\n      <Status></Status>\n      <LimitLo>3.2</LimitLo>\n      <LimitHi>3.4</LimitHi>\n      <StringMatch></StringMatch>\n      <BooleanMatch></BooleanMatch>\n      <DisplayFormat>%.2f</DisplayFormat>\n      <Units>_V</Units>\n      <TestTime></TestTime>\n    </Test>\n    <Test>\n      <Code>10.173</Code>\n      <Name>SELECTOR_86_L</Name>\n      <Description></Description>\n      <Group>Pin_Tests</Group>\n      <IsGroup>No</IsGroup>\n      <Tag>Pin_Tests:SELECTOR_86_L</Tag>\n      <Method>Test_Pin_N_Low</Method>\n      <Parameter>CH86</Parameter>\n      <DataType>Dbl</DataType>\n      <Value></Value>\n      <Status></Status>\n      <LimitLo>0</LimitLo>\n      <LimitHi>0.01</LimitHi>\n      <StringMatch></StringMatch>\n      <BooleanMatch></BooleanMatch>\n      <DisplayFormat>%.2f</DisplayFormat>\n      <Units>_V</Units>\n      <TestTime></TestTime>\n    </Test>\n    <Test>\n      <Code>10.174</Code>\n      <Name>SELECTOR_87_H</Name>\n      <Description></Description>\n      <Group>Pin_Tests</Group>\n      <IsGroup>No</IsGroup>\n      <Tag>Pin_Tests:SELECTOR_87_H</Tag>\n      <Method>Test_Pin_N_High</Method>\n      <Parameter>CH87</Parameter>\n      <DataType>Dbl</DataType>\n      <Value></Value>\n      <Status></Status>\n      <LimitLo>3.2</LimitLo>\n      <LimitHi>3.4</LimitHi>\n      <StringMatch></StringMatch>\n      <BooleanMatch></BooleanMatch>\n      <DisplayFormat>%.2f</DisplayFormat>\n      <Units>_V</Units>\n      <TestTime></TestTime>\n    </Test>\n    <Test>\n      <Code>10.175</Code>\n      <Name>SELECTOR_87_L</Name>\n      <Description></Description>\n      <Group>Pin_Tests</Group>\n      <IsGroup>No</IsGroup>\n      <Tag>Pin_Tests:SELECTOR_87_L</Tag>\n      <Method>Test_Pin_N_Low</Method>\n      <Parameter>CH87</Parameter>\n      <DataType>Dbl</DataType>\n      <Value></Value>\n      <Status></Status>\n      <LimitLo>0</LimitLo>\n      <LimitHi>0.01</LimitHi>\n      <StringMatch></StringMatch>\n      <BooleanMatch></BooleanMatch>\n      <DisplayFormat>%.2f</DisplayFormat>\n      <Units>_V</Units>\n      <TestTime></TestTime>\n    </Test>\n    <Test>\n      <Code>10.176</Code>\n      <Name>SELECTOR_88_H</Name>\n      <Description></Description>\n      <Group>Pin_Tests</Group>\n      <IsGroup>No</IsGroup>\n      <Tag>Pin_Tests:SELECTOR_88_H</Tag>\n      <Method>Test_Pin_N_High</Method>\n      <Parameter>CH88</Parameter>\n      <DataType>Dbl</DataType>\n      <Value></Value>\n      <Status></Status>\n      <LimitLo>3.2</LimitLo>\n      <LimitHi>3.4</LimitHi>\n      <StringMatch></StringMatch>\n      <BooleanMatch></BooleanMatch>\n      <DisplayFormat>%.2f</DisplayFormat>\n      <Units>_V</Units>\n      <TestTime></TestTime>\n    </Test>\n    <Test>\n      <Code>10.177</Code>\n      <Name>SELECTOR_88_L</Name>\n      <Description></Description>\n      <Group>Pin_Tests</Group>\n      <IsGroup>No</IsGroup>\n      <Tag>Pin_Tests:SELECTOR_88_L</Tag>\n      <Method>Test_Pin_N_Low</Method>\n      <Parameter>CH88</Parameter>\n      <DataType>Dbl</DataType>\n      <Value></Value>\n      <Status></Status>\n      <LimitLo>0</LimitLo>\n      <LimitHi>0.01</LimitHi>\n      <StringMatch></StringMatch>\n      <BooleanMatch></BooleanMatch>\n      <DisplayFormat>%.2f</DisplayFormat>\n      <Units>_V</Units>\n      <TestTime></TestTime>\n    </Test>\n    <Test>\n      <Code>10.178</Code>\n      <Name>SELECTOR_89_H</Name>\n      <Description></Description>\n      <Group>Pin_Tests</Group>\n      <IsGroup>No</IsGroup>\n      <Tag>Pin_Tests:SELECTOR_89_H</Tag>\n      <Method>Test_Pin_N_High</Method>\n      <Parameter>CH89</Parameter>\n      <DataType>Dbl</DataType>\n      <Value></Value>\n      <Status></Status>\n      <LimitLo>3.2</LimitLo>\n      <LimitHi>3.4</LimitHi>\n      <StringMatch></StringMatch>\n      <BooleanMatch></BooleanMatch>\n      <DisplayFormat>%.2f</DisplayFormat>\n      <Units>_V</Units>\n      <TestTime></TestTime>\n    </Test>\n    <Test>\n      <Code>10.179</Code>\n      <Name>SELECTOR_89_L</Name>\n      <Description></Description>\n      <Group>Pin_Tests</Group>\n      <IsGroup>No</IsGroup>\n      <Tag>Pin_Tests:SELECTOR_89_L</Tag>\n      <Method>Test_Pin_N_Low</Method>\n      <Parameter>CH89</Parameter>\n      <DataType>Dbl</DataType>\n      <Value></Value>\n      <Status></Status>\n      <LimitLo>0</LimitLo>\n      <LimitHi>0.01</LimitHi>\n      <StringMatch></StringMatch>\n      <BooleanMatch></BooleanMatch>\n      <DisplayFormat>%.2f</DisplayFormat>\n      <Units>_V</Units>\n      <TestTime></TestTime>\n    </Test>\n    <Test>\n      <Code>10.180</Code>\n      <Name>SELECTOR_90_H</Name>\n      <Description></Description>\n      <Group>Pin_Tests</Group>\n      <IsGroup>No</IsGroup>\n      <Tag>Pin_Tests:SELECTOR_90_H</Tag>\n      <Method>Test_Pin_N_High</Method>\n      <Parameter>CH90</Parameter>\n      <DataType>Dbl</DataType>\n      <Value></Value>\n      <Status></Status>\n      <LimitLo>3.2</LimitLo>\n      <LimitHi>3.4</LimitHi>\n      <StringMatch></StringMatch>\n      <BooleanMatch></BooleanMatch>\n      <DisplayFormat>%.2f</DisplayFormat>\n      <Units>_V</Units>\n      <TestTime></TestTime>\n    </Test>\n    <Test>\n      <Code>10.181</Code>\n      <Name>SELECTOR_90_L</Name>\n      <Description></Description>\n      <Group>Pin_Tests</Group>\n      <IsGroup>No</IsGroup>\n      <Tag>Pin_Tests:SELECTOR_90_L</Tag>\n      <Method>Test_Pin_N_Low</Method>\n      <Parameter>CH90</Parameter>\n      <DataType>Dbl</DataType>\n      <Value></Value>\n      <Status></Status>\n      <LimitLo>0</LimitLo>\n      <LimitHi>0.01</LimitHi>\n      <StringMatch></StringMatch>\n      <BooleanMatch></BooleanMatch>\n      <DisplayFormat>%.2f</DisplayFormat>\n      <Units>_V</Units>\n      <TestTime></TestTime>\n    </Test>\n    <Test>\n      <Code>10.182</Code>\n      <Name>SELECTOR_91_H</Name>\n      <Description></Description>\n      <Group>Pin_Tests</Group>\n      <IsGroup>No</IsGroup>\n      <Tag>Pin_Tests:SELECTOR_91_H</Tag>\n      <Method>Test_Pin_N_High</Method>\n      <Parameter>CH91</Parameter>\n      <DataType>Dbl</DataType>\n      <Value></Value>\n      <Status></Status>\n      <LimitLo>3.2</LimitLo>\n      <LimitHi>3.4</LimitHi>\n      <StringMatch></StringMatch>\n      <BooleanMatch></BooleanMatch>\n      <DisplayFormat>%.2f</DisplayFormat>\n      <Units>_V</Units>\n      <TestTime></TestTime>\n    </Test>\n    <Test>\n      <Code>10.183</Code>\n      <Name>SELECTOR_91_L</Name>\n      <Description></Description>\n      <Group>Pin_Tests</Group>\n      <IsGroup>No</IsGroup>\n      <Tag>Pin_Tests:SELECTOR_91_L</Tag>\n      <Method>Test_Pin_N_Low</Method>\n      <Parameter>CH91</Parameter>\n      <DataType>Dbl</DataType>\n      <Value></Value>\n      <Status></Status>\n      <LimitLo>0</LimitLo>\n      <LimitHi>0.01</LimitHi>\n      <StringMatch></StringMatch>\n      <BooleanMatch></BooleanMatch>\n      <DisplayFormat>%.2f</DisplayFormat>\n      <Units>_V</Units>\n      <TestTime></TestTime>\n    </Test>\n    <Test>\n      <Code>10.184</Code>\n      <Name>SELECTOR_92_H</Name>\n      <Description></Description>\n      <Group>Pin_Tests</Group>\n      <IsGroup>No</IsGroup>\n      <Tag>Pin_Tests:SELECTOR_92_H</Tag>\n      <Method>Test_Pin_N_High</Method>\n      <Parameter>CH92</Parameter>\n      <DataType>Dbl</DataType>\n      <Value></Value>\n      <Status></Status>\n      <LimitLo>3.2</LimitLo>\n      <LimitHi>3.4</LimitHi>\n      <StringMatch></StringMatch>\n      <BooleanMatch></BooleanMatch>\n      <DisplayFormat>%.2f</DisplayFormat>\n      <Units>_V</Units>\n      <TestTime></TestTime>\n    </Test>\n    <Test>\n      <Code>10.185</Code>\n      <Name>SELECTOR_92_L</Name>\n      <Description></Description>\n      <Group>Pin_Tests</Group>\n      <IsGroup>No</IsGroup>\n      <Tag>Pin_Tests:SELECTOR_92_L</Tag>\n      <Method>Test_Pin_N_Low</Method>\n      <Parameter>CH92</Parameter>\n      <DataType>Dbl</DataType>\n      <Value></Value>\n      <Status></Status>\n      <LimitLo>0</LimitLo>\n      <LimitHi>0.01</LimitHi>\n      <StringMatch></StringMatch>\n      <BooleanMatch></BooleanMatch>\n      <DisplayFormat>%.2f</DisplayFormat>\n      <Units>_V</Units>\n      <TestTime></TestTime>\n    </Test>\n    <Test>\n      <Code>10.186</Code>\n      <Name>SELECTOR_93_H</Name>\n      <Description></Description>\n      <Group>Pin_Tests</Group>\n      <IsGroup>No</IsGroup>\n      <Tag>Pin_Tests:SELECTOR_93_H</Tag>\n      <Method>Test_Pin_N_High</Method>\n      <Parameter>CH93</Parameter>\n      <DataType>Dbl</DataType>\n      <Value></Value>\n      <Status></Status>\n      <LimitLo>3.2</LimitLo>\n      <LimitHi>3.4</LimitHi>\n      <StringMatch></StringMatch>\n      <BooleanMatch></BooleanMatch>\n      <DisplayFormat>%.2f</DisplayFormat>\n      <Units>_V</Units>\n      <TestTime></TestTime>\n    </Test>\n    <Test>\n      <Code>10.187</Code>\n      <Name>SELECTOR_93_L</Name>\n      <Description></Description>\n      <Group>Pin_Tests</Group>\n      <IsGroup>No</IsGroup>\n      <Tag>Pin_Tests:SELECTOR_93_L</Tag>\n      <Method>Test_Pin_N_Low</Method>\n      <Parameter>CH93</Parameter>\n      <DataType>Dbl</DataType>\n      <Value></Value>\n      <Status></Status>\n      <LimitLo>0</LimitLo>\n      <LimitHi>0.01</LimitHi>\n      <StringMatch></StringMatch>\n      <BooleanMatch></BooleanMatch>\n      <DisplayFormat>%.2f</DisplayFormat>\n      <Units>_V</Units>\n      <TestTime></TestTime>\n    </Test>\n    <Test>\n      <Code>10.188</Code>\n      <Name>SELECTOR_94_H</Name>\n      <Description></Description>\n      <Group>Pin_Tests</Group>\n      <IsGroup>No</IsGroup>\n      <Tag>Pin_Tests:SELECTOR_94_H</Tag>\n      <Method>Test_Pin_N_High</Method>\n      <Parameter>CH94</Parameter>\n      <DataType>Dbl</DataType>\n      <Value></Value>\n      <Status></Status>\n      <LimitLo>3.2</LimitLo>\n      <LimitHi>3.4</LimitHi>\n      <StringMatch></StringMatch>\n      <BooleanMatch></BooleanMatch>\n      <DisplayFormat>%.2f</DisplayFormat>\n      <Units>_V</Units>\n      <TestTime></TestTime>\n    </Test>\n    <Test>\n      <Code>10.189</Code>\n      <Name>SELECTOR_94_L</Name>\n      <Description></Description>\n      <Group>Pin_Tests</Group>\n      <IsGroup>No</IsGroup>\n      <Tag>Pin_Tests:SELECTOR_94_L</Tag>\n      <Method>Test_Pin_N_Low</Method>\n      <Parameter>CH94</Parameter>\n      <DataType>Dbl</DataType>\n      <Value></Value>\n      <Status></Status>\n      <LimitLo>0</LimitLo>\n      <LimitHi>0.01</LimitHi>\n      <StringMatch></StringMatch>\n      <BooleanMatch></BooleanMatch>\n      <DisplayFormat>%.2f</DisplayFormat>\n      <Units>_V</Units>\n      <TestTime></TestTime>\n    </Test>\n    <Test>\n      <Code>10.190</Code>\n      <Name>SELECTOR_95_H</Name>\n      <Description></Description>\n      <Group>Pin_Tests</Group>\n      <IsGroup>No</IsGroup>\n      <Tag>Pin_Tests:SELECTOR_95_H</Tag>\n      <Method>Test_Pin_N_High</Method>\n      <Parameter>CH95</Parameter>\n      <DataType>Dbl</DataType>\n      <Value></Value>\n      <Status></Status>\n      <LimitLo>3.2</LimitLo>\n      <LimitHi>3.4</LimitHi>\n      <StringMatch></StringMatch>\n      <BooleanMatch></BooleanMatch>\n      <DisplayFormat>%.2f</DisplayFormat>\n      <Units>_V</Units>\n      <TestTime></TestTime>\n    </Test>\n    <Test>\n      <Code>10.191</Code>\n      <Name>SELECTOR_95_L</Name>\n      <Description></Description>\n      <Group>Pin_Tests</Group>\n      <IsGroup>No</IsGroup>\n      <Tag>Pin_Tests:SELECTOR_95_L</Tag>\n      <Method>Test_Pin_N_Low</Method>\n      <Parameter>CH95</Parameter>\n      <DataType>Dbl</DataType>\n      <Value></Value>\n      <Status></Status>\n      <LimitLo>0</LimitLo>\n      <LimitHi>0.01</LimitHi>\n      <StringMatch></StringMatch>\n      <BooleanMatch></BooleanMatch>\n      <DisplayFormat>%.2f</DisplayFormat>\n      <Units>_V</Units>\n      <TestTime></TestTime>\n    </Test>\n    <Test>\n      <Code>10.192</Code>\n      <Name>SELECTOR_96_H</Name>\n      <Description></Description>\n      <Group>Pin_Tests</Group>\n      <IsGroup>No</IsGroup>\n      <Tag>Pin_Tests:SELECTOR_96_H</Tag>\n      <Method>Test_Pin_N_High</Method>\n      <Parameter>CH96</Parameter>\n      <DataType>Dbl</DataType>\n      <Value></Value>\n      <Status></Status>\n      <LimitLo>3.2</LimitLo>\n      <LimitHi>3.4</LimitHi>\n      <StringMatch></StringMatch>\n      <BooleanMatch></BooleanMatch>\n      <DisplayFormat>%.2f</DisplayFormat>\n      <Units>_V</Units>\n      <TestTime></TestTime>\n    </Test>\n    <Test>\n      <Code>10.193</Code>\n      <Name>SELECTOR_96_L</Name>\n      <Description></Description>\n      <Group>Pin_Tests</Group>\n      <IsGroup>No</IsGroup>\n      <Tag>Pin_Tests:SELECTOR_96_L</Tag>\n      <Method>Test_Pin_N_Low</Method>\n      <Parameter>CH96</Parameter>\n      <DataType>Dbl</DataType>\n      <Value></Value>\n      <Status></Status>\n      <LimitLo>0</LimitLo>\n      <LimitHi>0.01</LimitHi>\n      <StringMatch></StringMatch>\n      <BooleanMatch></BooleanMatch>\n      <DisplayFormat>%.2f</DisplayFormat>\n      <Units>_V</Units>\n      <TestTime></TestTime>\n    </Test>\n    <Test>\n      <Code>10.194</Code>\n      <Name>SELECTOR_97_H</Name>\n      <Description></Description>\n      <Group>Pin_Tests</Group>\n      <IsGroup>No</IsGroup>\n      <Tag>Pin_Tests:SELECTOR_97_H</Tag>\n      <Method>Test_Pin_N_High</Method>\n      <Parameter>CH97</Parameter>\n      <DataType>Dbl</DataType>\n      <Value></Value>\n      <Status></Status>\n      <LimitLo>3.2</LimitLo>\n      <LimitHi>3.4</LimitHi>\n      <StringMatch></StringMatch>\n      <BooleanMatch></BooleanMatch>\n      <DisplayFormat>%.2f</DisplayFormat>\n      <Units>_V</Units>\n      <TestTime></TestTime>\n    </Test>\n    <Test>\n      <Code>10.195</Code>\n      <Name>SELECTOR_97_L</Name>\n      <Description></Description>\n      <Group>Pin_Tests</Group>\n      <IsGroup>No</IsGroup>\n      <Tag>Pin_Tests:SELECTOR_97_L</Tag>\n      <Method>Test_Pin_N_Low</Method>\n      <Parameter>CH97</Parameter>\n      <DataType>Dbl</DataType>\n      <Value></Value>\n      <Status></Status>\n      <LimitLo>0</LimitLo>\n      <LimitHi>0.01</LimitHi>\n      <StringMatch></StringMatch>\n      <BooleanMatch></BooleanMatch>\n      <DisplayFormat>%.2f</DisplayFormat>\n      <Units>_V</Units>\n      <TestTime></TestTime>\n    </Test>\n    <Test>\n      <Code>10.196</Code>\n      <Name>SELECTOR_98_H</Name>\n      <Description></Description>\n      <Group>Pin_Tests</Group>\n      <IsGroup>No</IsGroup>\n      <Tag>Pin_Tests:SELECTOR_98_H</Tag>\n      <Method>Test_Pin_N_High</Method>\n      <Parameter>CH98</Parameter>\n      <DataType>Dbl</DataType>\n      <Value></Value>\n      <Status></Status>\n      <LimitLo>3.2</LimitLo>\n      <LimitHi>3.4</LimitHi>\n      <StringMatch></StringMatch>\n      <BooleanMatch></BooleanMatch>\n      <DisplayFormat>%.2f</DisplayFormat>\n      <Units>_V</Units>\n      <TestTime></TestTime>\n    </Test>\n    <Test>\n      <Code>10.197</Code>\n      <Name>SELECTOR_98_L</Name>\n      <Description></Description>\n      <Group>Pin_Tests</Group>\n      <IsGroup>No</IsGroup>\n      <Tag>Pin_Tests:SELECTOR_98_L</Tag>\n      <Method>Test_Pin_N_Low</Method>\n      <Parameter>CH98</Parameter>\n      <DataType>Dbl</DataType>\n      <Value></Value>\n      <Status></Status>\n      <LimitLo>0</LimitLo>\n      <LimitHi>0.01</LimitHi>\n      <StringMatch></StringMatch>\n      <BooleanMatch></BooleanMatch>\n      <DisplayFormat>%.2f</DisplayFormat>\n      <Units>_V</Units>\n      <TestTime></TestTime>\n    </Test>\n    <Test>\n      <Code>10.198</Code>\n      <Name>SELECTOR_99_H</Name>\n      <Description></Description>\n      <Group>Pin_Tests</Group>\n      <IsGroup>No</IsGroup>\n      <Tag>Pin_Tests:SELECTOR_99_H</Tag>\n      <Method>Test_Pin_N_High</Method>\n      <Parameter>CH99</Parameter>\n      <DataType>Dbl</DataType>\n      <Value></Value>\n      <Status></Status>\n      <LimitLo>3.2</LimitLo>\n      <LimitHi>3.4</LimitHi>\n      <StringMatch></StringMatch>\n      <BooleanMatch></BooleanMatch>\n      <DisplayFormat>%.2f</DisplayFormat>\n      <Units>_V</Units>\n      <TestTime></TestTime>\n    </Test>\n    <Test>\n      <Code>10.199</Code>\n      <Name>SELECTOR_99_L</Name>\n      <Description></Description>\n      <Group>Pin_Tests</Group>\n      <IsGroup>No</IsGroup>\n      <Tag>Pin_Tests:SELECTOR_99_L</Tag>\n      <Method>Test_Pin_N_Low</Method>\n      <Parameter>CH99</Parameter>\n      <DataType>Dbl</DataType>\n      <Value></Value>\n      <Status></Status>\n      <LimitLo>0</LimitLo>\n      <LimitHi>0.01</LimitHi>\n      <StringMatch></StringMatch>\n      <BooleanMatch></BooleanMatch>\n      <DisplayFormat>%.2f</DisplayFormat>\n      <Units>_V</Units>\n      <TestTime></TestTime>\n    </Test>\n    <Test>\n      <Code>10.200</Code>\n      <Name>SELECTOR_100_H</Name>\n      <Description></Description>\n      <Group>Pin_Tests</Group>\n      <IsGroup>No</IsGroup>\n      <Tag>Pin_Tests:SELECTOR_100_H</Tag>\n      <Method>Test_Pin_N_High</Method>\n      <Parameter>CH100</Parameter>\n      <DataType>Dbl</DataType>\n      <Value></Value>\n      <Status></Status>\n      <LimitLo>3.2</LimitLo>\n      <LimitHi>3.4</LimitHi>\n      <StringMatch></StringMatch>\n      <BooleanMatch></BooleanMatch>\n      <DisplayFormat>%.2f</DisplayFormat>\n      <Units>_V</Units>\n      <TestTime></TestTime>\n    </Test>\n    <Test>\n      <Code>10.201</Code>\n      <Name>SELECTOR_100_L</Name>\n      <Description></Description>\n      <Group>Pin_Tests</Group>\n      <IsGroup>No</IsGroup>\n      <Tag>Pin_Tests:SELECTOR_100_L</Tag>\n      <Method>Test_Pin_N_Low</Method>\n      <Parameter>CH100</Parameter>\n      <DataType>Dbl</DataType>\n      <Value></Value>\n      <Status></Status>\n      <LimitLo>0</LimitLo>\n      <LimitHi>0.01</LimitHi>\n      <StringMatch></StringMatch>\n      <BooleanMatch></BooleanMatch>\n      <DisplayFormat>%.2f</DisplayFormat>\n      <Units>_V</Units>\n      <TestTime></TestTime>\n    </Test>\n    <Test>\n      <Code>10.202</Code>\n      <Name>SELECTOR_101_H</Name>\n      <Description></Description>\n      <Group>Pin_Tests</Group>\n      <IsGroup>No</IsGroup>\n      <Tag>Pin_Tests:SELECTOR_101_H</Tag>\n      <Method>Test_Pin_N_High</Method>\n      <Parameter>CH101</Parameter>\n      <DataType>Dbl</DataType>\n      <Value></Value>\n      <Status></Status>\n      <LimitLo>3.2</LimitLo>\n      <LimitHi>3.4</LimitHi>\n      <StringMatch></StringMatch>\n      <BooleanMatch></BooleanMatch>\n      <DisplayFormat>%.2f</DisplayFormat>\n      <Units>_V</Units>\n      <TestTime></TestTime>\n    </Test>\n    <Test>\n      <Code>10.203</Code>\n      <Name>SELECTOR_101_L</Name>\n      <Description></Description>\n      <Group>Pin_Tests</Group>\n      <IsGroup>No</IsGroup>\n      <Tag>Pin_Tests:SELECTOR_101_L</Tag>\n      <Method>Test_Pin_N_Low</Method>\n      <Parameter>CH101</Parameter>\n      <DataType>Dbl</DataType>\n      <Value></Value>\n      <Status></Status>\n      <LimitLo>0</LimitLo>\n      <LimitHi>0.01</LimitHi>\n      <StringMatch></StringMatch>\n      <BooleanMatch></BooleanMatch>\n      <DisplayFormat>%.2f</DisplayFormat>\n      <Units>_V</Units>\n      <TestTime></TestTime>\n    </Test>\n    <Test>\n      <Code>10.204</Code>\n      <Name>SELECTOR_102_H</Name>\n      <Description></Description>\n      <Group>Pin_Tests</Group>\n      <IsGroup>No</IsGroup>\n      <Tag>Pin_Tests:SELECTOR_102_H</Tag>\n      <Method>Test_Pin_N_High</Method>\n      <Parameter>CH102</Parameter>\n      <DataType>Dbl</DataType>\n      <Value></Value>\n      <Status></Status>\n      <LimitLo>3.2</LimitLo>\n      <LimitHi>3.4</LimitHi>\n      <StringMatch></StringMatch>\n      <BooleanMatch></BooleanMatch>\n      <DisplayFormat>%.2f</DisplayFormat>\n      <Units>_V</Units>\n      <TestTime></TestTime>\n    </Test>\n    <Test>\n      <Code>10.205</Code>\n      <Name>SELECTOR_102_L</Name>\n      <Description></Description>\n      <Group>Pin_Tests</Group>\n      <IsGroup>No</IsGroup>\n      <Tag>Pin_Tests:SELECTOR_102_L</Tag>\n      <Method>Test_Pin_N_Low</Method>\n      <Parameter>CH102</Parameter>\n      <DataType>Dbl</DataType>\n      <Value></Value>\n      <Status></Status>\n      <LimitLo>0</LimitLo>\n      <LimitHi>0.01</LimitHi>\n      <StringMatch></StringMatch>\n      <BooleanMatch></BooleanMatch>\n      <DisplayFormat>%.2f</DisplayFormat>\n      <Units>_V</Units>\n      <TestTime></TestTime>\n    </Test>\n    <Test>\n      <Code>10.206</Code>\n      <Name>SELECTOR_103_H</Name>\n      <Description></Description>\n      <Group>Pin_Tests</Group>\n      <IsGroup>No</IsGroup>\n      <Tag>Pin_Tests:SELECTOR_103_H</Tag>\n      <Method>Test_Pin_N_High</Method>\n      <Parameter>CH103</Parameter>\n      <DataType>Dbl</DataType>\n      <Value></Value>\n      <Status></Status>\n      <LimitLo>3.2</LimitLo>\n      <LimitHi>3.4</LimitHi>\n      <StringMatch></StringMatch>\n      <BooleanMatch></BooleanMatch>\n      <DisplayFormat>%.2f</DisplayFormat>\n      <Units>_V</Units>\n      <TestTime></TestTime>\n    </Test>\n    <Test>\n      <Code>10.207</Code>\n      <Name>SELECTOR_103_L</Name>\n      <Description></Description>\n      <Group>Pin_Tests</Group>\n      <IsGroup>No</IsGroup>\n      <Tag>Pin_Tests:SELECTOR_103_L</Tag>\n      <Method>Test_Pin_N_Low</Method>\n      <Parameter>CH103</Parameter>\n      <DataType>Dbl</DataType>\n      <Value></Value>\n      <Status></Status>\n      <LimitLo>0</LimitLo>\n      <LimitHi>0.01</LimitHi>\n      <StringMatch></StringMatch>\n      <BooleanMatch></BooleanMatch>\n      <DisplayFormat>%.2f</DisplayFormat>\n      <Units>_V</Units>\n      <TestTime></TestTime>\n    </Test>\n    <Test>\n      <Code>10.208</Code>\n      <Name>SELECTOR_104_H</Name>\n      <Description></Description>\n      <Group>Pin_Tests</Group>\n      <IsGroup>No</IsGroup>\n      <Tag>Pin_Tests:SELECTOR_104_H</Tag>\n      <Method>Test_Pin_N_High</Method>\n      <Parameter>CH104</Parameter>\n      <DataType>Dbl</DataType>\n      <Value></Value>\n      <Status></Status>\n      <LimitLo>3.2</LimitLo>\n      <LimitHi>3.4</LimitHi>\n      <StringMatch></StringMatch>\n      <BooleanMatch></BooleanMatch>\n      <DisplayFormat>%.2f</DisplayFormat>\n      <Units>_V</Units>\n      <TestTime></TestTime>\n    </Test>\n    <Test>\n      <Code>10.209</Code>\n      <Name>SELECTOR_104_L</Name>\n      <Description></Description>\n      <Group>Pin_Tests</Group>\n      <IsGroup>No</IsGroup>\n      <Tag>Pin_Tests:SELECTOR_104_L</Tag>\n      <Method>Test_Pin_N_Low</Method>\n      <Parameter>CH104</Parameter>\n      <DataType>Dbl</DataType>\n      <Value></Value>\n      <Status></Status>\n      <LimitLo>0</LimitLo>\n      <LimitHi>0.01</LimitHi>\n      <StringMatch></StringMatch>\n      <BooleanMatch></BooleanMatch>\n      <DisplayFormat>%.2f</DisplayFormat>\n      <Units>_V</Units>\n      <TestTime></TestTime>\n    </Test>\n    <Test>\n      <Code>10.210</Code>\n      <Name>SELECTOR_105_H</Name>\n      <Description></Description>\n      <Group>Pin_Tests</Group>\n      <IsGroup>No</IsGroup>\n      <Tag>Pin_Tests:SELECTOR_105_H</Tag>\n      <Method>Test_Pin_N_High</Method>\n      <Parameter>CH105</Parameter>\n      <DataType>Dbl</DataType>\n      <Value></Value>\n      <Status></Status>\n      <LimitLo>3.2</LimitLo>\n      <LimitHi>3.4</LimitHi>\n      <StringMatch></StringMatch>\n      <BooleanMatch></BooleanMatch>\n      <DisplayFormat>%.2f</DisplayFormat>\n      <Units>_V</Units>\n      <TestTime></TestTime>\n    </Test>\n    <Test>\n      <Code>10.211</Code>\n      <Name>SELECTOR_105_L</Name>\n      <Description></Description>\n      <Group>Pin_Tests</Group>\n      <IsGroup>No</IsGroup>\n      <Tag>Pin_Tests:SELECTOR_105_L</Tag>\n      <Method>Test_Pin_N_Low</Method>\n      <Parameter>CH105</Parameter>\n      <DataType>Dbl</DataType>\n      <Value></Value>\n      <Status></Status>\n      <LimitLo>0</LimitLo>\n      <LimitHi>0.01</LimitHi>\n      <StringMatch></StringMatch>\n      <BooleanMatch></BooleanMatch>\n      <DisplayFormat>%.2f</DisplayFormat>\n      <Units>_V</Units>\n      <TestTime></TestTime>\n    </Test>\n    <Test>\n      <Code>10.212</Code>\n      <Name>SELECTOR_106_H</Name>\n      <Description></Description>\n      <Group>Pin_Tests</Group>\n      <IsGroup>No</IsGroup>\n      <Tag>Pin_Tests:SELECTOR_106_H</Tag>\n      <Method>Test_Pin_N_High</Method>\n      <Parameter>CH106</Parameter>\n      <DataType>Dbl</DataType>\n      <Value></Value>\n      <Status></Status>\n      <LimitLo>3.2</LimitLo>\n      <LimitHi>3.4</LimitHi>\n      <StringMatch></StringMatch>\n      <BooleanMatch></BooleanMatch>\n      <DisplayFormat>%.2f</DisplayFormat>\n      <Units>_V</Units>\n      <TestTime></TestTime>\n    </Test>\n    <Test>\n      <Code>10.213</Code>\n      <Name>SELECTOR_106_L</Name>\n      <Description></Description>\n      <Group>Pin_Tests</Group>\n      <IsGroup>No</IsGroup>\n      <Tag>Pin_Tests:SELECTOR_106_L</Tag>\n      <Method>Test_Pin_N_Low</Method>\n      <Parameter>CH106</Parameter>\n      <DataType>Dbl</DataType>\n      <Value></Value>\n      <Status></Status>\n      <LimitLo>0</LimitLo>\n      <LimitHi>0.01</LimitHi>\n      <StringMatch></StringMatch>\n      <BooleanMatch></BooleanMatch>\n      <DisplayFormat>%.2f</DisplayFormat>\n      <Units>_V</Units>\n      <TestTime></TestTime>\n    </Test>\n    <Test>\n      <Code>10.214</Code>\n      <Name>SELECTOR_107_H</Name>\n      <Description></Description>\n      <Group>Pin_Tests</Group>\n      <IsGroup>No</IsGroup>\n      <Tag>Pin_Tests:SELECTOR_107_H</Tag>\n      <Method>Test_Pin_N_High</Method>\n      <Parameter>CH107</Parameter>\n      <DataType>Dbl</DataType>\n      <Value></Value>\n      <Status></Status>\n      <LimitLo>3.2</LimitLo>\n      <LimitHi>3.4</LimitHi>\n      <StringMatch></StringMatch>\n      <BooleanMatch></BooleanMatch>\n      <DisplayFormat>%.2f</DisplayFormat>\n      <Units>_V</Units>\n      <TestTime></TestTime>\n    </Test>\n    <Test>\n      <Code>10.215</Code>\n      <Name>SELECTOR_107_L</Name>\n      <Description></Description>\n      <Group>Pin_Tests</Group>\n      <IsGroup>No</IsGroup>\n      <Tag>Pin_Tests:SELECTOR_107_L</Tag>\n      <Method>Test_Pin_N_Low</Method>\n      <Parameter>CH107</Parameter>\n      <DataType>Dbl</DataType>\n      <Value></Value>\n      <Status></Status>\n      <LimitLo>0</LimitLo>\n      <LimitHi>0.01</LimitHi>\n      <StringMatch></StringMatch>\n      <BooleanMatch></BooleanMatch>\n      <DisplayFormat>%.2f</DisplayFormat>\n      <Units>_V</Units>\n      <TestTime></TestTime>\n    </Test>\n    <Test>\n      <Code>10.216</Code>\n      <Name>SELECTOR_108_H</Name>\n      <Description></Description>\n      <Group>Pin_Tests</Group>\n      <IsGroup>No</IsGroup>\n      <Tag>Pin_Tests:SELECTOR_108_H</Tag>\n      <Method>Test_Pin_N_High</Method>\n      <Parameter>CH108</Parameter>\n      <DataType>Dbl</DataType>\n      <Value></Value>\n      <Status></Status>\n      <LimitLo>3.2</LimitLo>\n      <LimitHi>3.4</LimitHi>\n      <StringMatch></StringMatch>\n      <BooleanMatch></BooleanMatch>\n      <DisplayFormat>%.2f</DisplayFormat>\n      <Units>_V</Units>\n      <TestTime></TestTime>\n    </Test>\n    <Test>\n      <Code>10.217</Code>\n      <Name>SELECTOR_108_L</Name>\n      <Description></Description>\n      <Group>Pin_Tests</Group>\n      <IsGroup>No</IsGroup>\n      <Tag>Pin_Tests:SELECTOR_108_L</Tag>\n      <Method>Test_Pin_N_Low</Method>\n      <Parameter>CH108</Parameter>\n      <DataType>Dbl</DataType>\n      <Value></Value>\n      <Status></Status>\n      <LimitLo>0</LimitLo>\n      <LimitHi>0.01</LimitHi>\n      <StringMatch></StringMatch>\n      <BooleanMatch></BooleanMatch>\n      <DisplayFormat>%.2f</DisplayFormat>\n      <Units>_V</Units>\n      <TestTime></TestTime>\n    </Test>\n    <Test>\n      <Code>10.218</Code>\n      <Name>SELECTOR_109_H</Name>\n      <Description></Description>\n      <Group>Pin_Tests</Group>\n      <IsGroup>No</IsGroup>\n      <Tag>Pin_Tests:SELECTOR_109_H</Tag>\n      <Method>Test_Pin_N_High</Method>\n      <Parameter>CH109</Parameter>\n      <DataType>Dbl</DataType>\n      <Value></Value>\n      <Status></Status>\n      <LimitLo>3.2</LimitLo>\n      <LimitHi>3.4</LimitHi>\n      <StringMatch></StringMatch>\n      <BooleanMatch></BooleanMatch>\n      <DisplayFormat>%.2f</DisplayFormat>\n      <Units>_V</Units>\n      <TestTime></TestTime>\n    </Test>\n    <Test>\n      <Code>10.219</Code>\n      <Name>SELECTOR_109_L</Name>\n      <Description></Description>\n      <Group>Pin_Tests</Group>\n      <IsGroup>No</IsGroup>\n      <Tag>Pin_Tests:SELECTOR_109_L</Tag>\n      <Method>Test_Pin_N_Low</Method>\n      <Parameter>CH109</Parameter>\n      <DataType>Dbl</DataType>\n      <Value></Value>\n      <Status></Status>\n      <LimitLo>0</LimitLo>\n      <LimitHi>0.01</LimitHi>\n      <StringMatch></StringMatch>\n      <BooleanMatch></BooleanMatch>\n      <DisplayFormat>%.2f</DisplayFormat>\n      <Units>_V</Units>\n      <TestTime></TestTime>\n    </Test>\n    <Test>\n      <Code>10.220</Code>\n      <Name>SELECTOR_110_H</Name>\n      <Description></Description>\n      <Group>Pin_Tests</Group>\n      <IsGroup>No</IsGroup>\n      <Tag>Pin_Tests:SELECTOR_110_H</Tag>\n      <Method>Test_Pin_N_High</Method>\n      <Parameter>CH110</Parameter>\n      <DataType>Dbl</DataType>\n      <Value></Value>\n      <Status></Status>\n      <LimitLo>3.2</LimitLo>\n      <LimitHi>3.4</LimitHi>\n      <StringMatch></StringMatch>\n      <BooleanMatch></BooleanMatch>\n      <DisplayFormat>%.2f</DisplayFormat>\n      <Units>_V</Units>\n      <TestTime></TestTime>\n    </Test>\n    <Test>\n      <Code>10.221</Code>\n      <Name>SELECTOR_110_L</Name>\n      <Description></Description>\n      <Group>Pin_Tests</Group>\n      <IsGroup>No</IsGroup>\n      <Tag>Pin_Tests:SELECTOR_110_L</Tag>\n      <Method>Test_Pin_N_Low</Method>\n      <Parameter>CH110</Parameter>\n      <DataType>Dbl</DataType>\n      <Value></Value>\n      <Status></Status>\n      <LimitLo>0</LimitLo>\n      <LimitHi>0.01</LimitHi>\n      <StringMatch></StringMatch>\n      <BooleanMatch></BooleanMatch>\n      <DisplayFormat>%.2f</DisplayFormat>\n      <Units>_V</Units>\n      <TestTime></TestTime>\n    </Test>\n    <Test>\n      <Code>10.222</Code>\n      <Name>SELECTOR_111_H</Name>\n      <Description></Description>\n      <Group>Pin_Tests</Group>\n      <IsGroup>No</IsGroup>\n      <Tag>Pin_Tests:SELECTOR_111_H</Tag>\n      <Method>Test_Pin_N_High</Method>\n      <Parameter>CH111</Parameter>\n      <DataType>Dbl</DataType>\n      <Value></Value>\n      <Status></Status>\n      <LimitLo>3.2</LimitLo>\n      <LimitHi>3.4</LimitHi>\n      <StringMatch></StringMatch>\n      <BooleanMatch></BooleanMatch>\n      <DisplayFormat>%.2f</DisplayFormat>\n      <Units>_V</Units>\n      <TestTime></TestTime>\n    </Test>\n    <Test>\n      <Code>10.223</Code>\n      <Name>SELECTOR_111_L</Name>\n      <Description></Description>\n      <Group>Pin_Tests</Group>\n      <IsGroup>No</IsGroup>\n      <Tag>Pin_Tests:SELECTOR_111_L</Tag>\n      <Method>Test_Pin_N_Low</Method>\n      <Parameter>CH111</Parameter>\n      <DataType>Dbl</DataType>\n      <Value></Value>\n      <Status></Status>\n      <LimitLo>0</LimitLo>\n      <LimitHi>0.01</LimitHi>\n      <StringMatch></StringMatch>\n      <BooleanMatch></BooleanMatch>\n      <DisplayFormat>%.2f</DisplayFormat>\n      <Units>_V</Units>\n      <TestTime></TestTime>\n    </Test>\n    <Test>\n      <Code>10.224</Code>\n      <Name>SELECTOR_112_H</Name>\n      <Description></Description>\n      <Group>Pin_Tests</Group>\n      <IsGroup>No</IsGroup>\n      <Tag>Pin_Tests:SELECTOR_112_H</Tag>\n      <Method>Test_Pin_N_High</Method>\n      <Parameter>CH112</Parameter>\n      <DataType>Dbl</DataType>\n      <Value></Value>\n      <Status></Status>\n      <LimitLo>3.2</LimitLo>\n      <LimitHi>3.4</LimitHi>\n      <StringMatch></StringMatch>\n      <BooleanMatch></BooleanMatch>\n      <DisplayFormat>%.2f</DisplayFormat>\n      <Units>_V</Units>\n      <TestTime></TestTime>\n    </Test>\n    <Test>\n      <Code>10.225</Code>\n      <Name>SELECTOR_112_L</Name>\n      <Description></Description>\n      <Group>Pin_Tests</Group>\n      <IsGroup>No</IsGroup>\n      <Tag>Pin_Tests:SELECTOR_112_L</Tag>\n      <Method>Test_Pin_N_Low</Method>\n      <Parameter>CH112</Parameter>\n      <DataType>Dbl</DataType>\n      <Value></Value>\n      <Status></Status>\n      <LimitLo>0</LimitLo>\n      <LimitHi>0.01</LimitHi>\n      <StringMatch></StringMatch>\n      <BooleanMatch></BooleanMatch>\n      <DisplayFormat>%.2f</DisplayFormat>\n      <Units>_V</Units>\n      <TestTime></TestTime>\n    </Test>\n    <Test>\n      <Code>10.226</Code>\n      <Name>SELECTOR_113_H</Name>\n      <Description></Description>\n      <Group>Pin_Tests</Group>\n      <IsGroup>No</IsGroup>\n      <Tag>Pin_Tests:SELECTOR_113_H</Tag>\n      <Method>Test_Pin_N_High</Method>\n      <Parameter>CH113</Parameter>\n      <DataType>Dbl</DataType>\n      <Value></Value>\n      <Status></Status>\n      <LimitLo>3.2</LimitLo>\n      <LimitHi>3.4</LimitHi>\n      <StringMatch></StringMatch>\n      <BooleanMatch></BooleanMatch>\n      <DisplayFormat>%.2f</DisplayFormat>\n      <Units>_V</Units>\n      <TestTime></TestTime>\n    </Test>\n    <Test>\n      <Code>10.227</Code>\n      <Name>SELECTOR_113_L</Name>\n      <Description></Description>\n      <Group>Pin_Tests</Group>\n      <IsGroup>No</IsGroup>\n      <Tag>Pin_Tests:SELECTOR_113_L</Tag>\n      <Method>Test_Pin_N_Low</Method>\n      <Parameter>CH113</Parameter>\n      <DataType>Dbl</DataType>\n      <Value></Value>\n      <Status></Status>\n      <LimitLo>0</LimitLo>\n      <LimitHi>0.01</LimitHi>\n      <StringMatch></StringMatch>\n      <BooleanMatch></BooleanMatch>\n      <DisplayFormat>%.2f</DisplayFormat>\n      <Units>_V</Units>\n      <TestTime></TestTime>\n    </Test>\n    <Test>\n      <Code>11</Code>\n      <Name>Wait_SPI_Flash</Name>\n      <Description>Wait SPI Flash Programing</Description>\n      <Group></Group>\n      <IsGroup>Yes</IsGroup>\n      <Tag>Wait_SPI_Flash</Tag>\n      <Method></Method>\n      <Parameter />\n      <DataType></DataType>\n      <Value></Value>\n      <Status></Status>\n      <LimitLo></LimitLo>\n      <LimitHi></LimitHi>\n      <StringMatch></StringMatch>\n      <BooleanMatch></BooleanMatch>\n      <DisplayFormat></DisplayFormat>\n      <Units></Units>\n      <TestTime></TestTime>\n    </Test>\n    <Test>\n      <Code>11.1</Code>\n      <Name>Wait_Program</Name>\n      <Description>Wait Program the fremont</Description>\n      <Group>Wait_SPI_Flash</Group>\n      <IsGroup>No</IsGroup>\n      <Tag>Wait_SPI_Flash:Wait_Program</Tag>\n      <Method>WaitFlash</Method>\n      <Parameter></Parameter>\n      <DataType>Boolean</DataType>\n      <Value></Value>\n      <Status></Status>\n      <LimitLo></LimitLo>\n      <LimitHi></LimitHi>\n      <StringMatch></StringMatch>\n      <BooleanMatch>1</BooleanMatch>\n      <DisplayFormat></DisplayFormat>\n      <Units></Units>\n      <TestTime></TestTime>\n    </Test>\n  </Tests>\n</Medulla>") -> (0 "error out":errorcluster, 3 "Spec":T1)   [LabVIEW 2022 SP3, in "MES_Base.lvlib" / "MES_Base.lvclass"]
uses:
  MES_Base.lvclass
  Controls/Spec.ctl
  Controls/SpecHeader.ctl
  Controls/Status.ctl
  Controls/SpecComponent.ctl
  Controls/SpecAttribute.ctl
  Controls/DataType.ctl
  Controls/Test.ctl
panel:
  # "<SerialNumber>23214</SerialNumber>\n      <PartNumber>1234</PartNumber>\n      <Revision>A</Revision>\n      <BatchNumber></BatchNumber>\n      <Name>Grism</Name>\n      <Description>The Grism</Description>\n      <Attached>Yes</Attached>"
  # "<Attribute>\n      <Name>Address</Name>\n      <Description>The IP of the Unit</Description>\n      <DataType>String</DataType>\n      <Value>192.168.1.7</Value>\n      <Access>R</Access>\n      <Required>NA</Required>\n    </Attribute>"
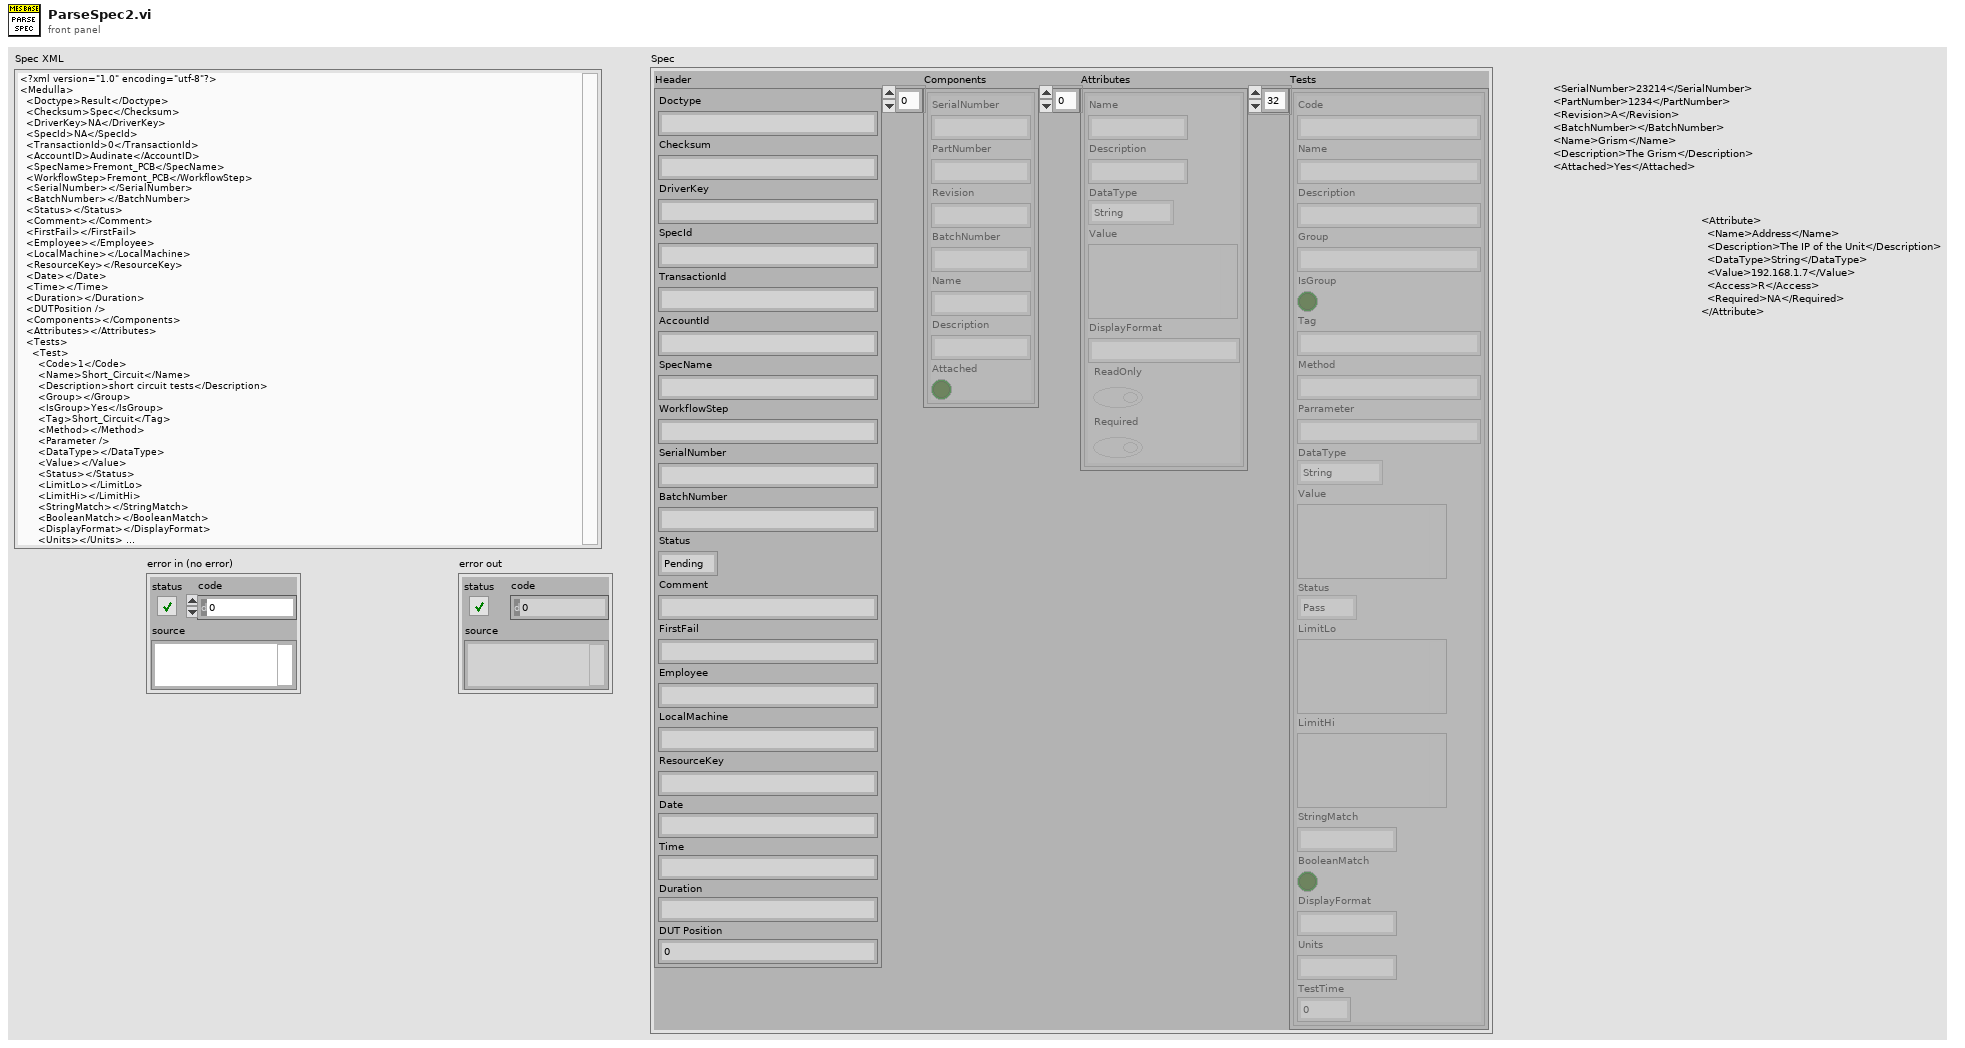
[diagram p1: front panel]
types:
  T1 = typedef "MES_Base.lvlib/MES_Base.lvclass/Spec.ctl" = cluster{"Header":T2, "Components":T4[], "Attributes":T5[], "Tests":T7[]}
  T2 = typedef "MES_Base.lvlib/MES_Base.lvclass/SpecHeader.ctl" = cluster{"Doctype":string, "Checksum":string, "DriverKey":string, "SpecId":string, "TransactionId":string, "AccountId":string, "SpecName":string, "WorkflowStep":string, "SerialNumber":string, "BatchNumber":string, "Status":T3, "Comment":string, "FirstFail":string, "Employee":string, "LocalMachine":string, "ResourceKey":string, "Date":string, "Time":string, "Duration":string, "DUT Position":i32}
  T3 = typedef "MES_Base.lvlib/MES_Base.lvclass/Status.ctl" = enum16{"Pending", "Pass", "Fail"}
  T4 = typedef "MES_Base.lvlib/MES_Base.lvclass/SpecComponent.ctl" = cluster{"SerialNumber":string, "PartNumber":string, "Revision":string, "BatchNumber":string, "Name":string, "Description":string, "Attached":bool}
  T5 = typedef "MES_Base.lvlib/MES_Base.lvclass/SpecAttribute.ctl" = cluster{"Name":string, "Description":string, "DataType":T6, "Value":variant, "DisplayFormat":string, "ReadOnly":bool, "Required":bool}
  T6 = typedef "MES_Base.lvlib/MES_Base.lvclass/DataType.ctl" = enum16{"NA", "String", "Boolean", "Int", "Dbl"}
  T7 = typedef "MES_Base.lvlib/MES_Base.lvclass/Test.ctl" = cluster{"Code":string, "Name":string, "Description":string, "Group":string, "IsGroup":bool, "Tag":string, "Method":string, "Parrameter":string, "DataType":T6, "Value":variant, "Status":T3, "LimitLo":variant, "LimitHi":variant, "StringMatch":string, "BooleanMatch":bool, "DisplayFormat":string, "Units":string, "TestTime":dbl}
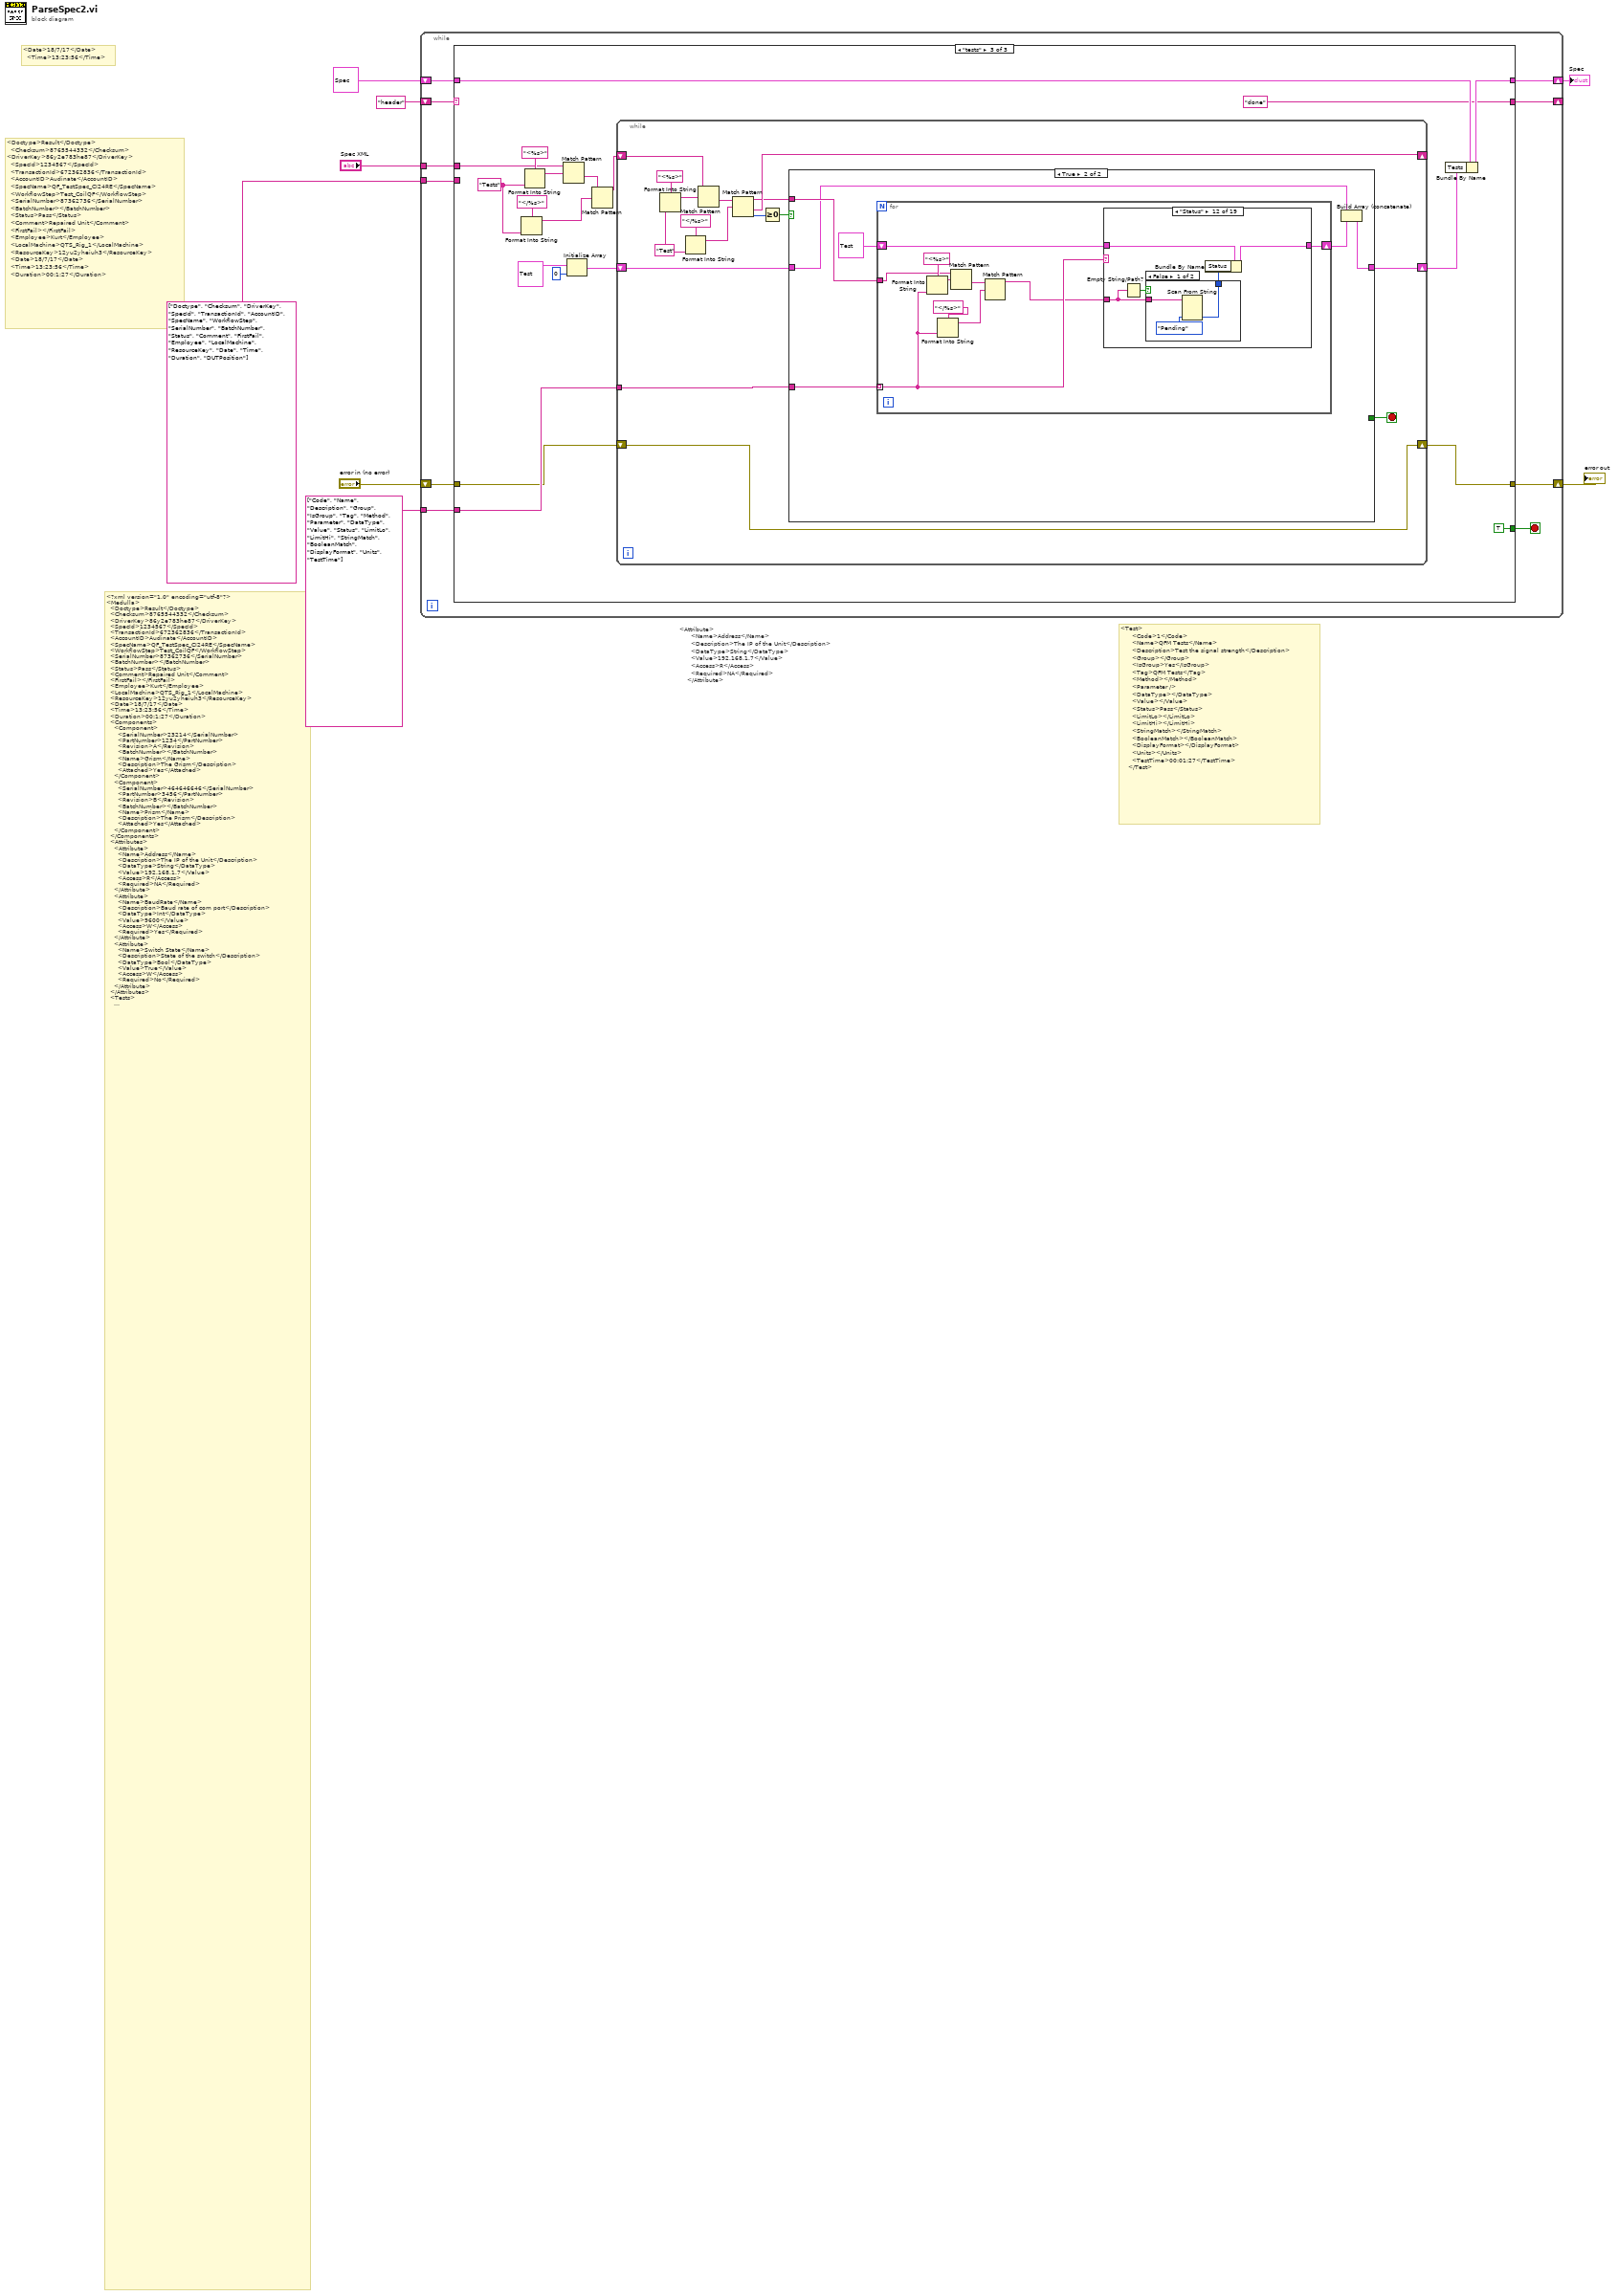
[diagram p0: block diagram]
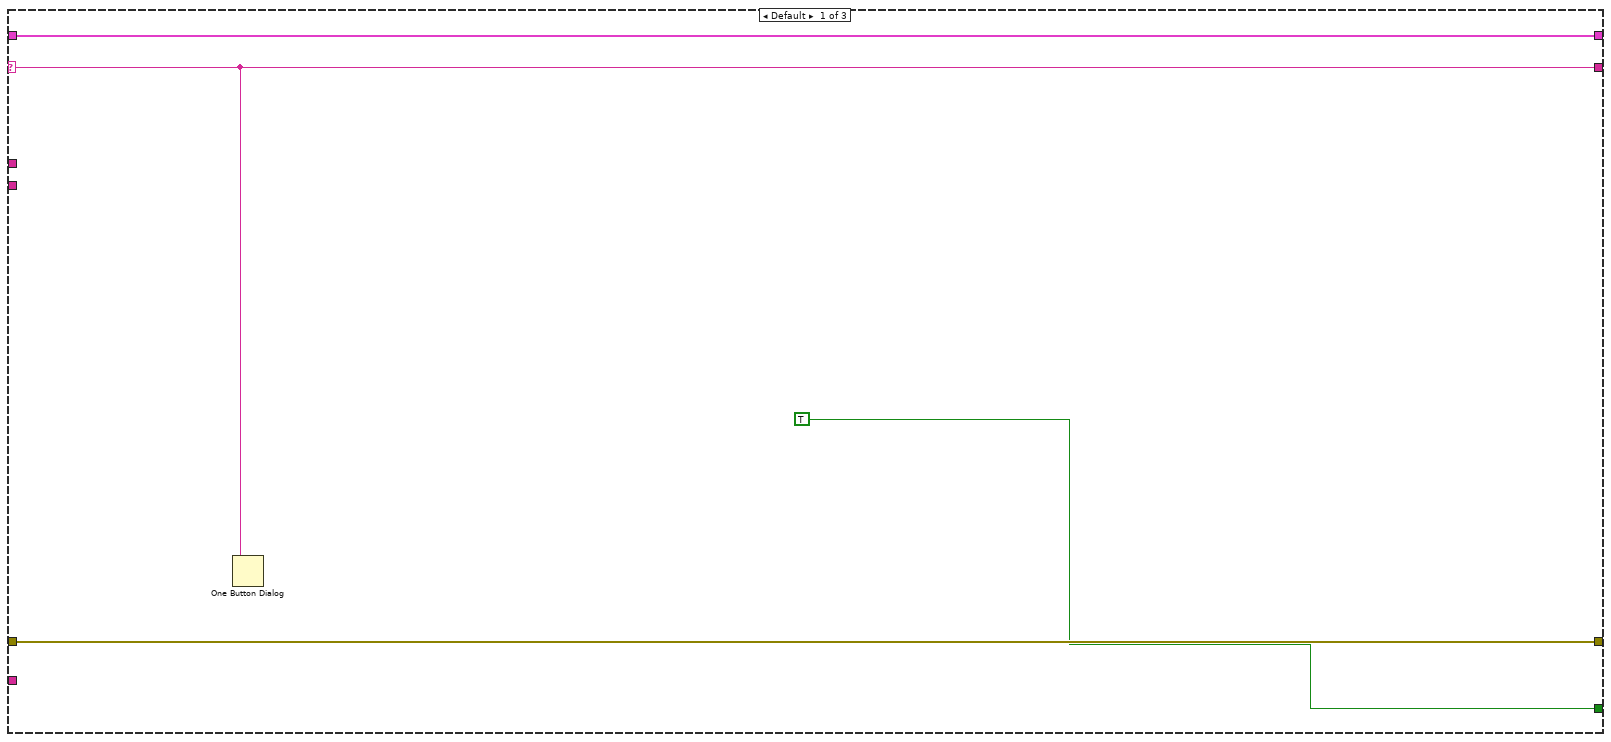
[diagram p2: hidden frame]
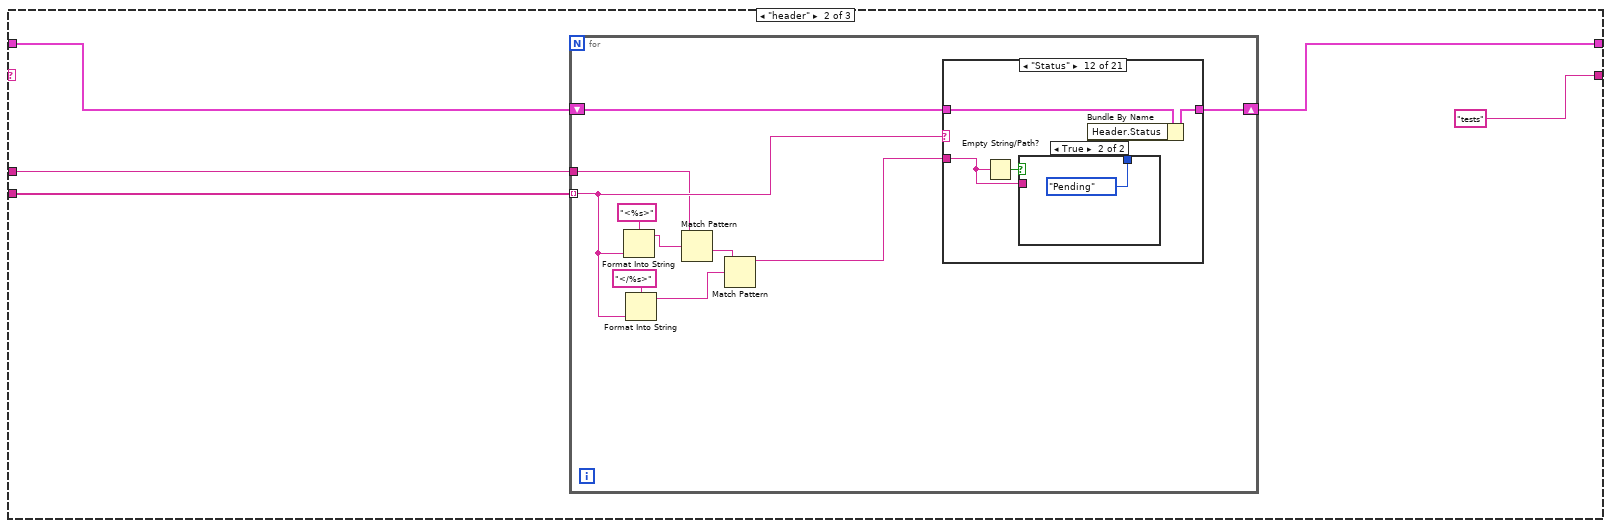
[diagram p3: hidden frame]
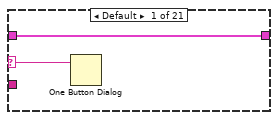
[diagram p4: hidden frame]
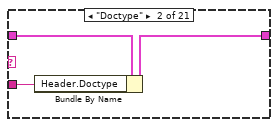
[diagram p5: hidden frame]
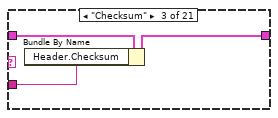
[diagram p6: hidden frame]
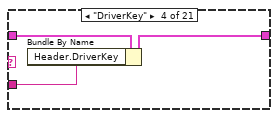
[diagram p7: hidden frame]
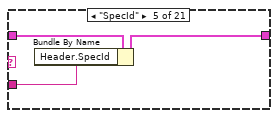
[diagram p8: hidden frame]
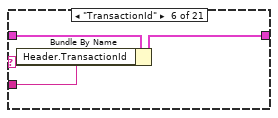
[diagram p9: hidden frame]
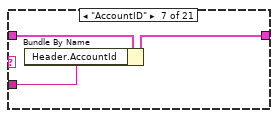
[diagram p10: hidden frame]
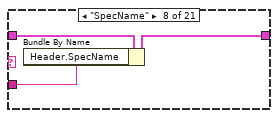
[diagram p11: hidden frame]
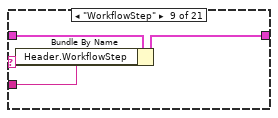
[diagram p12: hidden frame]
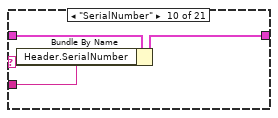
[diagram p13: hidden frame]
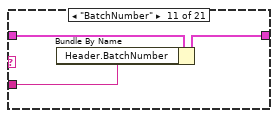
[diagram p14: hidden frame]
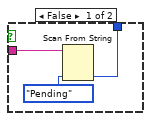
[diagram p15: hidden frame]
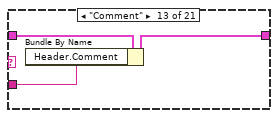
[diagram p16: hidden frame]
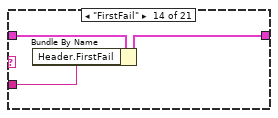
[diagram p17: hidden frame]
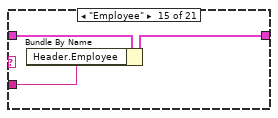
[diagram p18: hidden frame]
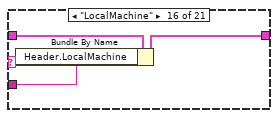
[diagram p19: hidden frame]
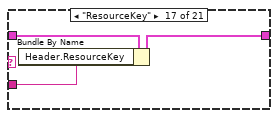
[diagram p20: hidden frame]
diagram:
  # "<Date>18/7/17</Date>\n  <Time>13:23:56</Time>"
  # "<Test>\n      <Code>1</Code>\n      <Name>QFM Tests</Name>\n      <Description>Test the signal strength</Description>\n      <Group></Group>\n      <IsGroup>Yes</IsGroup>\n      <Tag>QFM Tests</Tag>\n      <Method></Method>\n      <Parameter />\n      <DataType></DataType>\n      <Value></Value>\n      <Status>Pass</Status>\n      <LimitLo></LimitLo>\n      <LimitHi></LimitHi>\n      <StringMatch></StringMatch>\n      <BooleanMatch></BooleanMatch>\n      <DisplayFormat></DisplayFormat>\n      <Units></Units>\n      <TestTime>00:01:27</TestTime>\n    </Test>"
  # "<Attribute>\n      <Name>Address</Name>\n      <Description>The IP of the Unit</Description>\n      <DataType>String</DataType>\n      <Value>192.168.1.7</Value>\n      <Access>R</Access>\n      <Required>NA</Required>\n    </Attribute>"
  # "<Doctype>Result</Doctype>\n  <Checksum>8765544332</Checksum>\n<DriverKey>86y2e783he87</DriverKey>\n  <SpecId>1234567</SpecId>\n  <TransactionId>672362836</TransactionId>\n  <AccountID>Audinate</AccountID>\n  <SpecName>QF_TestSpec_CI24RE</SpecName>\n  <WorkflowStep>Test_CoilQF</WorkflowStep>\n  <SerialNumber>87362736</SerialNumber>\n  <BatchNumber></BatchNumber>\n  <Status>Pass</Status>\n  <Comment>Repaired Unit</Comment>\n  <FirstFail></FirstFail>\n  <Employee>Kurt</Employee>\n  <LocalMachine>QTS_Rig_1</LocalMachine>\n  <ResourceKey>12yu2yheiuh3</ResourceKey>\n  <Date>18/7/17</Date>\n  <Time>13:23:56</Time>\n  <Duration>00:1:27</Duration>"
  # "<?xml version=\"1.0\" encoding=\"utf-8\"?>\n<Medulla>\n  <Doctype>Result</Doctype>\n  <Checksum>8765544332</Checksum>\n  <DriverKey>86y2e783he87</DriverKey>\n  <SpecId>1234567</SpecId>\n  <TransactionId>672362836</TransactionId>\n  <AccountID>Audinate</AccountID>\n  <SpecName>QF_TestSpec_CI24RE</SpecName>\n  <WorkflowStep>Test_CoilQF</WorkflowStep>\n  <SerialNumber>87362736</SerialNumber>\n  <BatchNumber></BatchNumber>\n  <Status>Pass</Status>\n  <Comment>Repaired Unit</Comment>\n  <FirstFail></FirstFail>\n  <Employee>Kurt</Employee>\n  <LocalMachine>QTS_Rig_1</LocalMachine>\n  <ResourceKey>12yu2yheiuh3</ResourceKey>\n  <Date>18/7/17</Date>\n  <Time>13:23:56</Time>\n  <Duration>00:1:27</Duration>\n  <Components>\n    <Component>\n      <SerialNumber>23214</SerialNumber>\n      <PartNumber>1234</PartNumber>\n      <Revision>A</Revision>\n      <BatchNumber></BatchNumber>\n      <Name>Grism</Name>\n      <Description>The Grism</Description>\n      <Attached>Yes</Attached>\n    </Component>\n    <Component>\n      <SerialNumber>464646646</SerialNumber>\n      <PartNumber>3456</PartNumber>\n      <Revision>B</Revision>\n      <BatchNumber></BatchNumber>\n      <Name>Prism</Name>\n      <Description>The Prism</Description>\n      <Attached>Yes</Attached>\n    </Component>\n  </Components>\n  <Attributes>\n    <Attribute>\n      <Name>Address</Name>\n      <Description>The IP of the Unit</Description>\n      <DataType>String</DataType>\n      <Value>192.168.1.7</Value>\n      <Access>R</Access>\n      <Required>NA</Required>\n    </Attribute>\n    <Attribute>\n      <Name>BaudRate</Name>\n      <Description>Baud rate of com port</Description>\n      <DataType>Int</DataType>\n      <Value>9600</Value>\n      <Access>W</Access>\n      <Required>Yes</Required>\n    </Attribute>\n    <Attribute>\n      <Name>Switch State</Name>\n      <Description>State of the switch</Description>\n      <DataType>Bool</DataType>\n      <Value>True</Value>\n      <Access>W</Access>\n      <Required>No</Required>\n    </Attribute>\n  </Attributes>\n  <Tests>\n    <Test>\n      <Code>1</Code>\n      <Name>QFM Tests</Name>\n      <Description>Test the signal strength</Description>\n      <Group></Group>\n      <IsGroup>Yes</IsGroup>\n      <Tag>QFM Tests</Tag>\n      <Method></Method>\n      <Parameter />\n      <DataType></DataType>\n      <Value></Value>\n      <Status>Pass</Status>\n      <LimitLo></LimitLo>\n      <LimitHi></LimitHi>\n      <StringMatch></StringMatch>\n      <BooleanMatch></BooleanMatch>\n      <DisplayFormat></DisplayFormat>\n      <Units></Units>\n      <TestTime>00:01:27</TestTime>\n    </Test>\n    <Test>\n      <Code>1.1</Code>\n      <Name>Test Signal Strength</Name>\n      <Description>Test the signal strength</Description>\n      <Group>QFM Tests</Group>\n      <IsGroup>No</IsGroup>\n      <Tag>QFM Tests:Test Signal Strength</Tag>\n      <Method>Test_Sig</Method>\n      <Parameter />\n      <DataType>Int</DataType>\n      <Value>34.56</Value>\n      <Status>Pass</Status>\n      <LimitLo>25</LimitLo>\n      <LimitHi>100</LimitHi>\n      <StringMatch></StringMatch>\n      <BooleanMatch></BooleanMatch>\n      <DisplayFormat>%d</DisplayFormat>\n      <Units>Watts</Units>\n      <TestTime>00:00:45</TestTime>\n    </Test>\n    <Test>\n      <Code>1.2</Code>\n      <Name>Test Signal Frequency</Name>\n      <Description>Test the signal frequency</Description>\n      <Group>QFM Tests</Group>\n      <IsGroup>No</IsGroup>\n      <Tag>QFM Tests:Test Signal Frequency</Tag>\n      <Method>Test_Freq</Method>\n      <Parameter />\n      <DataType>DBL</DataType>\n      <Value>45.67</Value>\n      <Status>Pass</Status>\n      <LimitLo>45</LimitLo>\n      <LimitHi>46</LimitHi>\n      <StringMatch></StringMatch>\n      <BooleanMatch></BooleanMatch>\n      <DisplayFormat>%.3f</DisplayFormat>\n      <Units>MHz</Units>\n      <TestTime>00:00:20</TestTime>\n    </Test>\n    <Test>\n      <Code>Code</Code>\n      <Name>Test Firmware Vesion</Name>\n      <Description>Test the Firmware Vesion</Description>\n      <Group>QFM Tests</Group>\n      <IsGroup>No</IsGroup>\n      <Tag>QFM Tests:Test Firmware Vesion</Tag>\n      <Method>Test_FWVer</Method>\n      <Parameter />\n      <DataType>String</DataType>\n      <Value>Ver1.2</Value>\n      <Status>Pass</Status>\n      <LimitLo></LimitLo>\n      <LimitHi></LimitHi>\n      <StringMatch>Ver1.2</StringMatch>\n      <BooleanMatch></BooleanMatch>\n      <DisplayFormat></DisplayFormat>\n      <Units></Units>\n      <TestTime>00:00:12</TestTime>\n    </Test>\n    <Test>\n      <Code>Test LED State</Code>\n      <Name>Test LED State</Name>\n      <Description>Tests that the LED is On</Description>\n      <Group>QFM Tests</Group>\n      <IsGroup>No</IsGroup>\n      <Tag>QFM Tests:Test LED State</Tag>\n      <Method>Test_LED</Method>\n      <Parameter />\n      <DataType>Boolean</DataType>\n      <Value>True</Value>\n      <Status>True</Status>\n      <LimitLo></LimitLo>\n      <LimitHi></LimitHi>\n      <StringMatch></StringMatch>\n      <BooleanMatch>True</BooleanMatch>\n      <DisplayFormat></DisplayFormat>\n      <Units></Units>\n      <TestTime>00:00:10</TestTime>\n    </Test>\n  </Tests>\n</Medulla>"
  n1 = while {
    shift-right: [w13] -> w4
    shift-left: "error in (no error)" -> [w17]
    tunnel: "Spec XML" -> [w16]
    shift-right: [w11] -> _
    shift-left: "header" -> [w18]
    shift-right: [w12] -> w2
    shift-left: T1 {"Header"={"Doctype"="", "Checksum"="", "DriverKey"="", "SpecId"="", "TransactionId"="", "AccountId"="", "SpecName"="", "WorkflowStep"="", "SerialNumber"="", "BatchNumber"="", "Status"=enum."Pending", "Comment"="", "FirstFail"="", "Employee"="", "LocalMachine"="", "ResourceKey"="", "Date"="", "Time"="", "Duration"="", "DUT Position"=0}, "Components"=[], "Attributes"=[], "Tests"=[]} ("Spec") -> [w15]
    tunnel: string[] ["Doctype", "Checksum", "DriverKey", "SpecId", "TransactionId", "AccountID", "SpecName", "WorkflowStep", "SerialNumber", "BatchNumber", "Status", "Comment", "FirstFail", "Employee", "LocalMachine", "ResourceKey", "Date", "Time", "Duration", "DUTPosition"] -> [w14]
    tunnel: string[] ["Code", "Name", "Description", "Group", "IsGroup", "Tag", "Method", "Parameter", "DataType", "Value", "Status", "LimitLo", "LimitHi", "StringMatch", "BooleanMatch", "DisplayFormat", "Units", "TestTime"] -> [w9]
    stop <- w10 stop-if-true
    n2 = case shown="\"tests\"" w18 {
      selector: w18 -> [w19 _ _]
      tunnel: w17 -> [w22 _ w113]
      tunnel: w16 -> [_ w23 w115]
      tunnel: w15 -> [w20 w26 w124]
      tunnel: w14 -> [_ w27 _]
      tunnel: [w22 _ w125] -> w13
      tunnel: [w20 w25 w123] -> w12
      tunnel: [w19 "tests" "done"] -> w11
      tunnel: [TRUE _ TRUE] -> w10
      tunnel: w9 -> [_ _ w121]
      frame Default {
        n3 = One Button Dialog(message=w19) -> ()  [unwired: 1 in, 1 out]
      }
      frame "header" {
        n4 = for {
          tunnel: w27 -> [w34] mode=indexing
          shift-right: [w36] -> w25
          shift-left: w26 -> [w37]
          tunnel: w23 -> [w29]
          n5 = Format Into String(format string="<%s>" ("string"), w34) -> (resulting string=w30:string)  [unwired: 2 in, 1 out]
          n6 = Format Into String(format string="</%s>" ("string"), w34) -> (resulting string=w32:string)  [unwired: 2 in, 1 out]
          n7 = Match Pattern(string=w29, regular expression=w30) -> (after substring=w33:string)  [unwired: 1 in, 3 out]
          n8 = Match Pattern(string=w33, regular expression=w32) -> (before substring=w31:string)  [unwired: 1 in, 3 out]
          n9 = case shown="\"Status\"" w34 {
            selector: w34 -> [w38 _ _ _ _ _ _ _ _ _ _ _ _ _ _ _ _ _ _ _ _]
            tunnel: w37 -> [w39 w42 w45 w48 w51 w54 w57 w60 w63 w66 w69 w74 w81 w84 w87 w90 w93 w96 w99 w102 w106]
            tunnel: w31 -> [_ w40 w43 w46 w49 w52 w55 w58 w61 w64 w67 w70 w79 w82 w85 w88 w91 w94 w97 w100 w104]
            tunnel: [w39 w41 w44 w47 w50 w53 w56 w59 w62 w65 w68 w73 w80 w83 w86 w89 w92 w95 w98 w101 w105] -> w36
            frame Default {
              n10 = One Button Dialog(message=w38) -> ()  [unwired: 1 in, 1 out]
            }
            frame "Doctype" {
              n11 = Bundle By Name(cluster=w42, "Header.Doctype"=w40) -> (w41:T1)
            }
            frame "Checksum" {
              n12 = Bundle By Name(cluster=w45, "Header.Checksum"=w43) -> (w44:T1)
            }
            frame "DriverKey" {
              n13 = Bundle By Name(cluster=w48, "Header.DriverKey"=w46) -> (w47:T1)
            }
            frame "SpecId" {
              n14 = Bundle By Name(cluster=w51, "Header.SpecId"=w49) -> (w50:T1)
            }
            frame "TransactionId" {
              n15 = Bundle By Name(cluster=w54, "Header.TransactionId"=w52) -> (w53:T1)
            }
            frame "AccountID" {
              n16 = Bundle By Name(cluster=w57, "Header.AccountId"=w55) -> (w56:T1)
            }
            frame "SpecName" {
              n17 = Bundle By Name(cluster=w60, "Header.SpecName"=w58) -> (w59:T1)
            }
            frame "WorkflowStep" {
              n18 = Bundle By Name(cluster=w63, "Header.WorkflowStep"=w61) -> (w62:T1)
            }
            frame "SerialNumber" {
              n19 = Bundle By Name(cluster=w66, "Header.SerialNumber"=w64) -> (w65:T1)
            }
            frame "BatchNumber" {
              n20 = Bundle By Name(cluster=w69, "Header.BatchNumber"=w67) -> (w68:T1)
            }
            frame "Status" {
              n21 = Empty String/Path?(string/path=w70) -> (empty?=w72:bool)
              n22 = case shown="True" w72 {
                tunnel: [w76 Status."Pending" ("Status")] -> w71
                tunnel: w70 -> [w75 _]
                frame False {
                  n23 = Scan From String(input string=w75, default 1=Status."Pending" ("Status")) -> (output 1=w76:T3)  [unwired: 3 in, 3 out]
                }
                frame True {
                }
              }
              n24 = Bundle By Name(cluster=w74, "Header.Status"=w71) -> (w73:T1)
            }
            frame "Comment" {
              n25 = Bundle By Name(cluster=w81, "Header.Comment"=w79) -> (w80:T1)
            }
            frame "FirstFail" {
              n26 = Bundle By Name(cluster=w84, "Header.FirstFail"=w82) -> (w83:T1)
            }
            frame "Employee" {
              n27 = Bundle By Name(cluster=w87, "Header.Employee"=w85) -> (w86:T1)
            }
            frame "LocalMachine" {
              n28 = Bundle By Name(cluster=w90, "Header.LocalMachine"=w88) -> (w89:T1)
            }
            frame "ResourceKey" {
              n29 = Bundle By Name(cluster=w93, "Header.ResourceKey"=w91) -> (w92:T1)
            }
            frame "Date" {
              n30 = Bundle By Name(cluster=w96, "Header.Date"=w94) -> (w95:T1)
            }
            frame "Time" {
              n31 = Bundle By Name(cluster=w99, "Header.Time"=w97) -> (w98:T1)
            }
            frame "Duration" {
              n32 = Bundle By Name(cluster=w102, "Header.Duration"=w100) -> (w101:T1)
            }
            frame "DUTPosition" {
              n33 = Decimal String To Number(string=w104) -> (number=w103:i32)  [unwired: 2 in, 1 out]
              n34 = Bundle By Name(cluster=w106, "Header.DUT Position"=w103) -> (w105:T1)
            }
          }
        }
      }
      frame "tests" {
        w114 = "Tests" ("input 1")
        n35 = Format Into String(format string="</%s>" ("string"), w114) -> (resulting string=w119:string)  [unwired: 2 in, 1 out]
        n36 = Format Into String(format string="<%s>" ("string"), w114) -> (resulting string=w120:string)  [unwired: 2 in, 1 out]
        n37 = Match Pattern(string=w115, regular expression=w120) -> (after substring=w118:string)  [unwired: 1 in, 3 out]
        n38 = Initialize Array(T7 {"Code"="", "Name"="", "Description"="", "Group"="", "IsGroup"=FALSE, "Tag"="", "Method"="", "Parrameter"="", "DataType"=enum."String", "Value"=variant, "Status"=enum."Pass", "LimitLo"=variant, "LimitHi"=variant, "StringMatch"="", "BooleanMatch"=FALSE, "DisplayFormat"="", "Units"="", "TestTime"=0.0} ("Cluster 2"), 0 ("dimension size")) -> (w109:T7[])
        n39 = Match Pattern(string=w118, regular expression=w119) -> (before substring=w112:string)  [unwired: 1 in, 3 out]
        n40 = while {
          shift-right: [w127] -> w125
          shift-left: w113 -> [w127]
          tunnel: w121 -> [w130]
          shift-right: [w132] -> _
          shift-left: w112 -> [w136]
          shift-right: [w128] -> w108
          shift-left: w109 -> [w129]
          stop <- w126 stop-if-true
          w135 = "Test" ("input 1")
          n41 = Format Into String(format string="<%s>" ("string"), w135) -> (resulting string=w141:string)  [unwired: 2 in, 1 out]
          n42 = Format Into String(format string="</%s>" ("string"), w135) -> (resulting string=w140:string)  [unwired: 2 in, 1 out]
          n43 = Match Pattern(string=w136, regular expression=w141) -> (after substring=w139:string)  [unwired: 1 in, 3 out]
          n44 = Match Pattern(string=w139, regular expression=w140) -> (before substring=w131:string, after substring=w132:string, offset past match=w134:i32)  [unwired: 1 in, 1 out]
          n45 = Greater Or Equal To 0?(x=w134) -> (x >= 0?=w133:bool)
          n46 = case shown="True" w133 {
            tunnel: w131 -> [_ w147]
            tunnel: w130 -> [_ w148]
            tunnel: w129 -> [w143 w145]
            tunnel: [w143 w144] -> w128
            tunnel: [TRUE _] -> w126
            frame False {
            }
            frame True {
              n47 = for {
                tunnel: w148 -> [w151] mode=indexing
                shift-right: [w158] -> w146
                shift-left: T7 {"Code"="", "Name"="", "Description"="", "Group"="", "IsGroup"=FALSE, "Tag"="", "Method"="", "Parrameter"="", "DataType"=enum."String", "Value"=variant, "Status"=enum."Pass", "LimitLo"=variant, "LimitHi"=variant, "StringMatch"="", "BooleanMatch"=FALSE, "DisplayFormat"="", "Units"="", "TestTime"=0.0} ("Cluster 2") -> [w159]
                tunnel: w147 -> [w152]
                n48 = Format Into String(format string="<%s>" ("string"), w151) -> (resulting string=w157:string)  [unwired: 2 in, 1 out]
                n49 = Format Into String(format string="</%s>" ("string"), w151) -> (resulting string=w156:string)  [unwired: 2 in, 1 out]
                n50 = Match Pattern(string=w152, regular expression=w157) -> (after substring=w155:string)  [unwired: 1 in, 3 out]
                n51 = Match Pattern(string=w155, regular expression=w156) -> (before substring=w150:string)  [unwired: 1 in, 3 out]
                n52 = case shown="\"Status\"" w151 {
                  tunnel: w159 -> [w160 w163 w166 w169 w172 w177 w180 w183 w186 w188 w199 w218 w225 w236 w247 w252 w254 w258 w262]
                  tunnel: [w160 w162 w165 w168 w171 w176 w179 w182 w185 w191 w200 w217 w224 w235 w246 w251 w255 w257 w261] -> w158
                  tunnel: w150 -> [_ w161 w164 w167 w170 w175 w178 w181 w184 w190 w197 w215 w226 w237 w245 w250 w253 w256 w260]
                  frame Default {
                  }
                  frame "Code" {
                    n53 = Bundle By Name(cluster=w163, "Code"=w161) -> (w162:T7)
                  }
                  frame "Name" {
                    n54 = Bundle By Name(cluster=w166, "Name"=w164) -> (w165:T7)
                  }
                  frame "Description" {
                    n55 = Bundle By Name(cluster=w169, "Description"=w167) -> (w168:T7)
                  }
                  frame "Group" {
                    n56 = Bundle By Name(cluster=w172, "Group"=w170) -> (w171:T7)
                  }
                  frame "IsGroup" {
                    n57 = Equal?(x="Yes", y=w175) -> (x = y?=w173:bool)
                    n58 = Bundle By Name(cluster=w177, "IsGroup"=w173) -> (w176:T7)
                  }
                  frame "Tag" {
                    n59 = Bundle By Name(cluster=w180, "Tag"=w178) -> (w179:T7)
                  }
                  frame "Method" {
                    n60 = Bundle By Name(cluster=w183, "Method"=w181) -> (w182:T7)
                  }
                  frame "Parameter" {
                    n61 = Bundle By Name(cluster=w186, "Parrameter"=w184) -> (w185:T7)
                  }
                  frame "DataType" {
                    n62 = Unbundle By Name(w188) -> ("IsGroup"=w187:bool)
                    n63 = case shown="True" w187 {
                      tunnel: w190 -> [w194 _]
                      tunnel: [w193 DataType."NA" ("DataType")] -> w189
                      frame False {
                        n64 = Scan From String(input string=w194, default 1=DataType."NA" ("DataType")) -> (output 1=w193:T6)  [unwired: 3 in, 3 out]
                      }
                      frame True {
                      }
                    }
                    n65 = Bundle By Name(cluster=w188, "DataType"=w189) -> (w191:T7)
                  }
                  frame "Value" {
                    n66 = Unbundle By Name(w199) -> ("DataType"=w198:T6)
                    n67 = case shown="\"Dbl\"" w198 {
                      tunnel: w197 -> [w202 w206 w210 w212]
                      tunnel: [w201 w203 w207 w213] -> w196
                      frame "String", Default {
                        n68 = To Variant(anything=w202) -> (Variant=w201:variant)
                      }
                      frame "Boolean" {
                        n69 = Equal?(x="1", y=w206) -> (x = y?=w204:bool)
                        n70 = To Variant(anything=w204) -> (Variant=w203:variant)
                      }
                      frame "Int" {
                        n71 = Decimal String To Number(string=w210, default (0L)=i64 0 ("default (0 I32)")) -> (number=w208:i64)  [unwired: 1 in, 1 out]
                        n72 = To Variant(anything=w208) -> (Variant=w207:variant)
                      }
                      frame "Dbl" {
                        n73 = Fract/Exp String To Number(string=w212) -> (number=w211:dbl)  [unwired: 3 in, 1 out]
                        n74 = To Variant(anything=w211) -> (Variant=w213:variant)
                      }
                    }
                    n75 = Bundle By Name(cluster=w199, "Value"=w196) -> (w200:T7)
                  }
                  frame "Status" {
                    n76 = Empty String/Path?(string/path=w215) -> (empty?=w214:bool)
                    n77 = case shown="False" w214 {
                      tunnel: [w220 Status."Pending" ("Status")] -> w216
                      tunnel: w215 -> [w219 _]
                      frame False {
                        n78 = Scan From String(input string=w219, default 1=Status."Pending" ("Status")) -> (output 1=w220:T3)  [unwired: 3 in, 3 out]
                      }
                      frame True {
                      }
                    }
                    n79 = Bundle By Name(cluster=w218, "Status"=w216) -> (w217:T7)
                  }
                  frame "LimitLo" {
                    n80 = Unbundle By Name(w225) -> ("DataType"=w227:T6)
                    n81 = case shown="Default" w227 {
                      tunnel: w226 -> [_ w230 w233]
                      tunnel: [_ w228 w231] -> w223
                      frame Default {
                      }
                      frame "Dbl" {
                        n82 = Fract/Exp String To Number(string=w230) -> (number=w229:dbl)  [unwired: 3 in, 1 out]
                        n83 = To Variant(anything=w229) -> (Variant=w228:variant)
                      }
                      frame "Int" {
                        n84 = Decimal String To Number(string=w233) -> (number=w232:i32)  [unwired: 2 in, 1 out]
                        n85 = To Variant(anything=w232) -> (Variant=w231:variant)
                      }
                    }
                    n86 = Bundle By Name(cluster=w225, "LimitLo"=w223) -> (w224:T7)
                  }
                  frame "LimitHi" {
                    n87 = Unbundle By Name(w236) -> ("DataType"=w238:T6)
                    n88 = case shown="Default" w238 {
                      tunnel: w237 -> [_ w241 w244]
                      tunnel: [_ w239 w242] -> w234
                      frame Default {
                      }
                      frame "Dbl" {
                        n89 = Fract/Exp String To Number(string=w241) -> (number=w240:dbl)  [unwired: 3 in, 1 out]
                        n90 = To Variant(anything=w240) -> (Variant=w239:variant)
                      }
                      frame "Int" {
                        n91 = Decimal String To Number(string=w244) -> (number=w243:i32)  [unwired: 2 in, 1 out]
                        n92 = To Variant(anything=w243) -> (Variant=w242:variant)
                      }
                    }
                    n93 = Bundle By Name(cluster=w236, "LimitHi"=w234) -> (w235:T7)
                  }
                  frame "StringMatch" {
                    n94 = Bundle By Name(cluster=w247, "StringMatch"=w245) -> (w246:T7)
                  }
                  frame "BooleanMatch" {
                    n95 = Equal?(x="1", y=w250) -> (x = y?=w248:bool)
                    n96 = Bundle By Name(cluster=w252, "BooleanMatch"=w248) -> (w251:T7)
                  }
                  frame "DisplayFormat" {
                    n97 = Bundle By Name(cluster=w254, "DisplayFormat"=w253) -> (w255:T7)
                  }
                  frame "Units" {
                    n98 = Bundle By Name(cluster=w258, "Units"=w256) -> (w257:T7)
                  }
                  frame "TestTime" {
                    n99 = Fract/Exp String To Number(string=w260) -> (number=w259:dbl)  [unwired: 3 in, 1 out]
                    n100 = Bundle By Name(cluster=w262, "TestTime"=w259) -> (w261:T7)
                  }
                }
              }
              n101 = Build Array (concatenate)(w145, w146) -> (w144:T7[])
            }
          }
        }
        n102 = Bundle By Name(cluster=w124, "Tests"=w108) -> (w123:T1)
      }
    }
  }
  "error out" <- w4
  "Spec" <- w2
